vi "Main_Marvin.vi"() -> ()   [LabVIEW 2017]
uses:
  PCAN_Driver/ControlCAN.llb/DevType.ctl
  PCAN_Driver/ControlCAN.llb/CAN Channel.ctl
  PCAN_Driver/ControlCAN.llb/VCI_INIT_CONFIG.ctl
  PCAN_Driver/ControlCAN.llb/InitFlag.ctl
  PCAN_Driver/ControlCAN.llb/Fliter.ctl
  PCAN_Driver/ControlCAN.llb/Mode.ctl
  <vilib>/Utility/miscctls.llb/LVRowAndColumnTypeDef.ctl
  <vilib>/Utility/config.llb/Read Key (String).vi
  <vilib>/Utility/config.llb/Write Key (String).vi
  <vilib>/Utility/cursorutil.llb/Set Cursor (Icon Pict).vi
  PCAN_Driver/ControlCAN.lvlib
  <vilib>/Utility/config.llb/NI_LVConfig.lvlib
panel:
  in  "Index":string="5"
  out "Automation":bool
  out "ClosePanel 2":bool=TRUE
  out "ClosePanel":bool=TRUE
  out "Next SN":string
  out "Curret SN":string
  out "Array 5":dbl[](array[numeric])
  out "Array 4":dbl[](array[numeric])
  out "VC1500-2 Vel":dbl
  out "VC15100-1 Vel":dbl
  out "Array Test":T1(array[ring])
  out "TempAlg":bool=TRUE
  out "f":T2(ring)=enum."Empty"
  out "VC15100-2":dbl
  out "VC15100-1 Cur":dbl
  out "Auxiind":bool
  out "TempSensCalind":bool
  out "VisualInspectionResult":bool
  out "Burninind":bool
  out "TempControlind":bool
  out "MotorTempind":bool
  out "SpeedStopind":bool
  out "EnableTestind":bool
  out "ComTestind":bool
  out "SoftwareVer":string
  in  "SetSN":bool
  out "CurrentOffset":dbl
  out "Array 3":string[](array[string])
  out "Cal Value":string
  in  "Stop Burn-in":bool
  out "Array 2":dbl[](array[numeric])
  out "VISA resource name out":refnum<visa-resource-name>
  out "UUT":u8
  out "CAN Status":bool
  in  "Channel 2":T3 caption="Channel" items=["Channel 1", "Channel 2"]
  out "Config_CANAT":T9 {"DevType" items=["USB-CAN"=3, "USB-CAN2"=4]; "CanIndex" items=["通道1", "通道2"]; "VCI_INIT_CONFIG"."Fliter" items=["接收所有类型"=3, "只接收标准帧"=4, "只接收扩展帧"=7]; "VCI_INIT_CONFIG"."Mode" items=["正常工作", "自测模式（环回）", "仅侦听模式"]; "VCI_INIT_CONFIG"."InitFlag" items=["使用Flash参数", "使用界面设置参数"]}
  out "Array":u64[][](array[numeric]) format="%016x"
  out "Motor Phase Current RMS":dbl
  out "Ambient Temperature":dbl
  out "Speed error":bool
  out "Commutation err":bool
  out "Under voltage/Over voltage":bool
  out "Derated drive temp":bool
  out "Motor Over temperature":bool
  out "Motor Sensor temp Fauilre":bool
  out "Drive Over temperature":bool
  out "Drive Sensor temp Failure":bool
  out "Ambient Over temp":bool
  out "Ambient Sensor temp":bool
  out "DC Voltage":dbl
  out "DC Current":dbl
  out "Power transistor Heat sink Temp.":dbl
  out "Motor Stator Temp.":dbl
  out "Motor Speed RPM":dbl
  out "ECS State":u16
  out "Waveform Chart":dbl[](graph)
  out "UUT":string="EBAY"
  in  "Logger Path":path
  in  "Report":bool
  in  "Start":bool
  out "Table Out":string[][](table)=[["Led -Test & On/Rst.Msg.", "", "", "", "", "", "", "", "", " ", "", "", "", "", " "], ["Led Test", "", "#1", "-", "-", "", "", "", "", " ", "", "", "", "", ""], ["Com.RS232 Rst.Msg", "", "#2", "-", "-", "", "", "", "", " ", "", "", "", "", ""], ["Com.RS232 Ans.Msg", "", "#3", "-", "-", "", "", "", "", "", "", "", "", "", ""], ["", "", "", "", "", "", "", "", "", "", "", "", "", "", ""], ["Servo Voltage & Current", "", "", "", "", "", "", "", "FAIL", "", "", "", "", "", ""], ["Servo Voltage", "", "28.0", "+/-1", "V", "", "NaN", "", "FAIL", "", "6.0", "0.0", "100", "Average", ""], ["Servo Current", "", "0.15", "Max", "A", "", "NaN", "", "FAIL", "", "1.0", "0.0", "100", "Average", ""], ["", "", "", "", "", "", "", "", "", "", "", "", "", "", ""], ["Voltages Accurance", "", "", "", "", "", "", "", "FAIL", "", "", "", "", "", ""], ["Servo VCC 5V    ", "", "5.0", "+/-0.1", "V", "", "NaN", "", "FAIL", "", "1.0", "0.0", "100", "Average", ""], ["Servo VEE -6.8V", "", "-6.8", "+/-0.15", "V", "", "NaN", "", "FAIL", "", "1.0", "0.0", "100", "Average", ""], ["Ref_1_4.096V ?", "", "4.096", "+/-0.1", "V", "", "NaN", "", "FAIL", "", "1.0", "0.0", "100", "Average", ""], ["", "", "", "", "", "", "", "", "", "", "", "", "", "", ""], ["Power-Supply Changing", "", "", "", "", "", "", "", "", "", "", "", "", "", ""], ["Min. Power-Supply Volt. 18v ", "", "Led Flashes", "-", "-", "", "", "", "", "", "", "", "", "", ""], ["Max. Power-Supply Volt. 32v ", "", "Led Flashes", "-", "-", "", "", "", "", "", "", "", "", "", ""], ["Under Volt.Prot.28->5->18v", "", "Led Flashes", "-", "-", "", "", "", "", "", "", "", "", "", ""], ["", "", "", "", "", "", "", "", "", "", "", "", "", "", ""], ["Pos.Cmd.Accur.@Mode1", "", "Mxxxx=", "", "", "", "", "", "", "", "", "", "", "", ""], ["Pos.Cmnd.=0.5V F.B.", "", "59h", "+/-5", "", "", "", "", "", "", "1.0", "0.0", "1", "Average", ""], ["Pos.Cmnd.=2.0V F.B.", "", "195h", "+/-5", "", "", "", "", "", "", "1.0", "0.0", "1", "Average", ""], ["Pos.Cmnd.=4.5V F.B.", "", "3A5h", "+/-5", "", "", "", "", "", "", "1.0", "0.0", "1", "Average", ""], ["", "", "", "", "", "", "", "", "", "", "", "", "", "", ""], ["Pos.Cmd.Accur.@Mode2", "", "Mxxxx=", "", "", "", "", "", "FAIL", "", "", "", "", "", ""], ["Pos.Cmnd.=0.5V F.B", "", "59h", "+/-5", "", "", "57h", "", "PASS", "", "1.0", "0.0", "1", "Average", ""], ["Pos.Cmnd.=2.0V F.B.", "", "195h", "+/-5", "", "", "1CEh", "", "FAIL", "", "1.0", "0.0", "1", "Average", ""], ["Pos.Cmnd.=4.5V F.B.", "", "3A5h", "+/-5", "", "", "2BAh", "", "FAIL", "", "1.0", "0.0", "1", "Average", ""], ["", "", "", "", "", "", "", "", "", "", "", "", "", "", ""], ["Pot.Accur.@Mode1 ", "", "Rxxxx=", "", "", "", "", "", "FAIL", "", "", "", "", "", ""], ["Pot.simulate=0.5v Pot.Code.:", "", "173h", "+/-5", "", "", "7Bh", "", "FAIL", "", "1.0", "0.0", "1", "Average", ""], ["Pot.simulate=2.0v Pot.Code.:", "", "1F3h", "+/-5", "", "", "1F1h", "", "PASS", "", "1.0", "0.0", "1", "Average", ""], ["Pot.simulate=3.5v Pot.Code.:", "", "372h", "+/-5", "", "", "368h", "", "FAIL", "", "1.0", "0.0", "1", "Average", ""], ["", "", "", "", "", "", "", "", "", "", "", "", "", "", ""], ["Pot.Accur.@Mode2 ", "", "Rxxxx=", "", "", "", "", "", "FAIL", "", "", "", "", "", ""], ["Pot.simulate=0.5v Pot.Code.:", "", "C4h", "+/-5", "", "", "7Bh", "", "FAIL", "", "1.0", "0.0", "1", "Average", ""], ["Pot.simulate=2.0v Pot.Code.:", "", "1E3h", "+/-5", "", "", "1F1h", "", "FAIL", "", "1.0", "0.0", "1", "Average", ""], ["Pot.simulate=3.5v Pot.Code.:", "", "541h", "+/-5", "", "", "368h", "", "FAIL", "", "1.0", "0.0", "1", "Average", ""], ["", "", "", "", "", "", "", "", "", "", "", "", "", "", ""], ["Status Accur.@Mode1", "", "", "", "", "", "", "", "", "", "", "", "", "", ""], ["Pot. / Pos.Cmnd. 1.5v", "", "-1.8084", "+/-0.1", "V", "", "", "", "", "", "1.0", "0.0", "100", "Average", ""], ["Pot. / Pos.Cmnd. 2.0v", "", "-0.1584", "+/-0.1", "V", "", "", "", "", "", "1.0", "0.0", "100", "Average", ""], ["Pot. / Pos.Cmnd. 3.5v", "", "4.7916", "+/-0.1", "V", "", "", "", "", "", "1.0", "0.0", "100", "Average", ""]]
  in  "ATR":string[][](table)=[["Test Communication", "-", "-", "-", "-", ""], ["Set S/N", "-", "-", "-", "-", ""], ["Set Board Number", "-", "-", "-", "-", ""], [" ", "", "", "", "", ""], ["Test Communication", "-", "-", "-", "-", ""], ["Get S/N", "-", "-", "-", "", ""], ["Get Board Number", "-", "-", "-", "", ""], ["Get FW", "-", "-", "-", "", ""], ["Enable Motor", "", "", "", "", ""], ["Small position command", "", "", "", "", ""], ["Measure delta", "", "", "", "", ""], ["Velocity command", "", "", "", "", ""]]
  in  "Settings":bool
  in  "Refresh Button":bool
  out "Serial":bool
  in  "VISA resource name":refnum<visa-resource-name>="COM6"
  in  "Serial Com":bool
  in  "Help Button":bool
  out "Pannel User Message":string
  in  "Stop Button":bool
  # "Marvin"
  # "REDLER TECHNOLOGIES LTD"
  # "ver 1.2g"
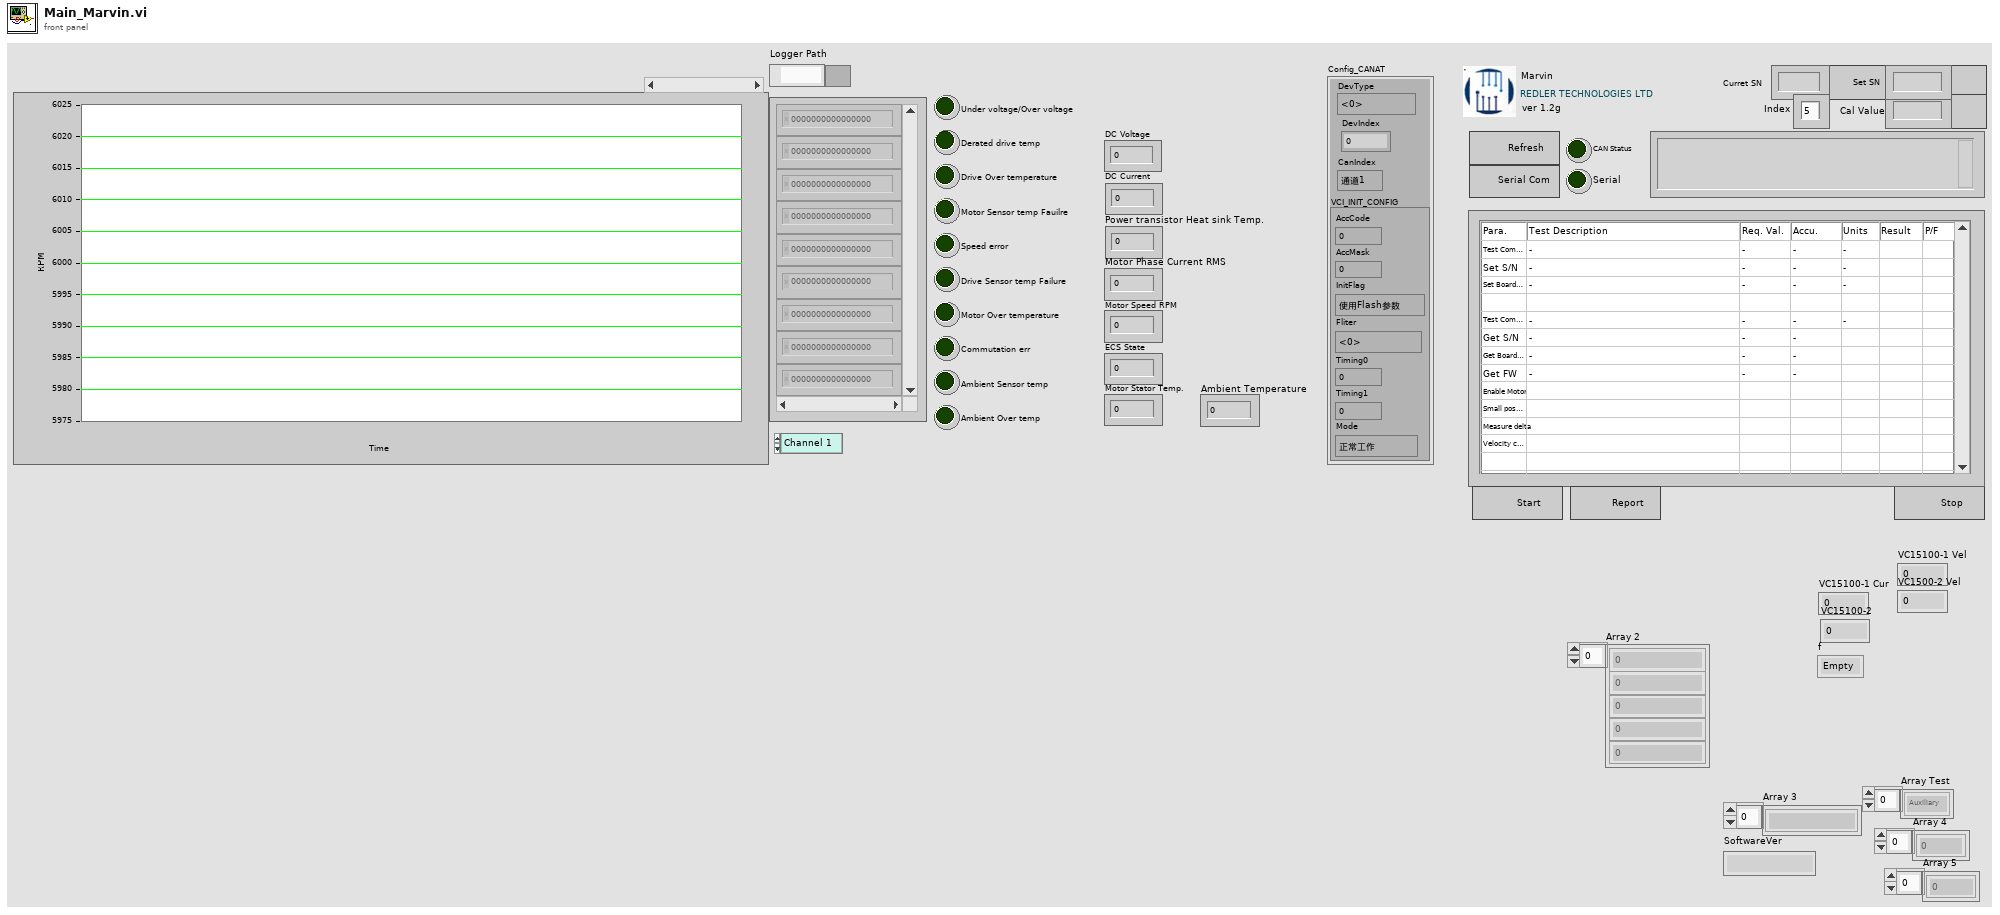
[diagram p1: front panel]
types:
  T1 = enum16{"Auxiliary", "Temp Sens Cal", "Com Test", "Enable Test", "Speed Command", "Stop Time", "Temp Control", "Burn in", "Visual Inspec", "Empty"}[]
  T2 = enum16{"Auxiliary", "Temp Sens Cal", "Com Test", "Enable Test", "Speed Command", "Stop Time", "Temp Control", "Burn in", "Visual Inspec", "Empty"}
  T3 = typedef "ControlCAN.lvlib/CAN Channel.ctl" = u32
  T4 = typedef "ControlCAN.lvlib/DevType.ctl" = u32
  T5 = typedef "ControlCAN.lvlib/VCI_INIT_CONFIG.ctl" = cluster{"AccCode":u32, "AccMask":u32, "InitFlag":T6, "Fliter":T7, "Timing0":u8, "Timing1":u8, "Mode":T8}
  T6 = typedef "ControlCAN.lvlib/InitFlag.ctl" = u32
  T7 = typedef "ControlCAN.lvlib/Fliter.ctl" = u8
  T8 = typedef "ControlCAN.lvlib/Mode.ctl" = u8
  T9 = cluster{"DevType":T4, "DevIndex":u32, "CanIndex":T3, "VCI_INIT_CONFIG":T5}
  T10 = cluster{"VISA":refnum<visa-resource-name>, "Array Test":enum16{"Auxiliary", "Temp Sens Cal", "Com Test", "Enable Test", "Speed Command", "Stop Time", "Temp Control", "Burn in", "Visual Inspec", "Empty"}[]}
  T11 = cluster{"ID":u32, "MSGTYPE":u8, "LEN":u8, "aDATA":u8[]}[]
  T12 = enum16{"Erase ATR Table", "Stop", "MainProgram", "Initialize"}
  T13 = enum8{"Enabled", "Disabled", "Disabled and Grayed Out"}
  T14 = enum16{"STOP", "VC15100-2", "RESET", "VC15100-1", "MD0"}
  T15 = typedef "NI_LVConfig.lvlib/Config Data RefNum.ctl" = refnum<k1>
  T16 = typedef "LVRowAndColumnTypeDef.ctl" = cluster{"Row":i32, "Column":i32}
  T17 = cluster{"ID":u32, "MSGTYPE":u8, "LEN":u8, "aDATA":u8[]}
  T18 = enum32{"Invalid", "Standard", "Closed", "Hidden", "Minimized", "Maximized"}
  T19 = enum16{"End", "Start", "Verify VR", "Verify UUT"}
  T20 = enum16{"open", "replace", "create", "open or create", "replace or create", "replace or create with confirmation"}
  T21 = typedef "ControlCAN.lvlib/VCI_CAN_OBJ.ctl" = cluster{"ID":u32, "TimeStamp":u32, "TimeFlag":u8, "SendType":u8, "RemoteFlag":u8, "ExternFlag":u8, "DataLen":u8, "Data":u8[], "Reserved":u8[]}
  T22 = cluster{"Type":enum16{"接收", "发送"}, "Channel":T3, "Time":timestamp, "VCI_CAN_OBJ":T21}[]
  T23 = cluster{"Type":enum16{"接收", "发送"}, "Channel":T3, "Time":timestamp, "VCI_CAN_OBJ":T21}
  T24 = typedef "LVPoint32TypeDef.ctl" = cluster{"Horizontal":i32, "Vertical":i32}
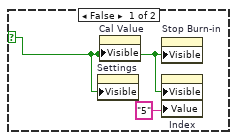
[diagram p3: hidden frame]
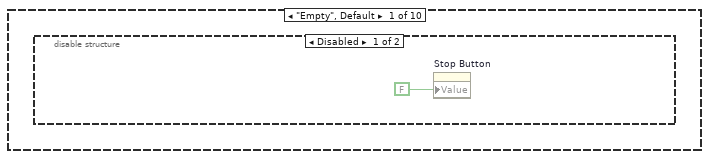
[diagram p6: hidden frame]
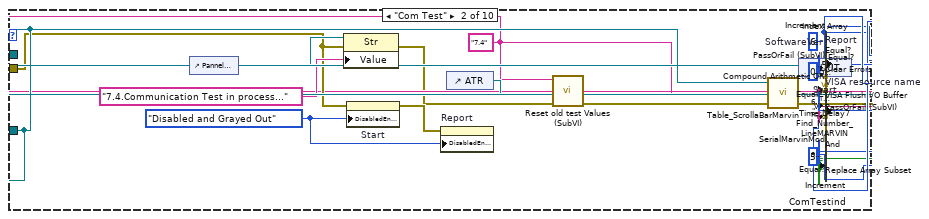
[diagram p8: hidden frame]
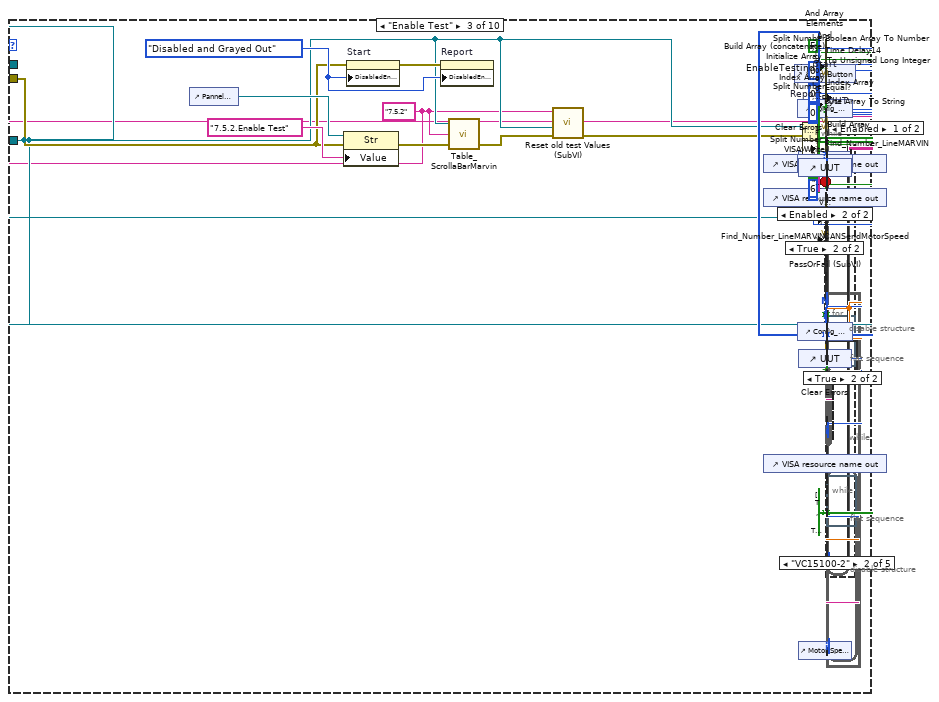
[diagram p9: hidden frame]
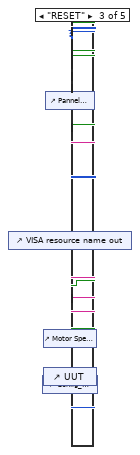
[diagram p17: hidden frame]
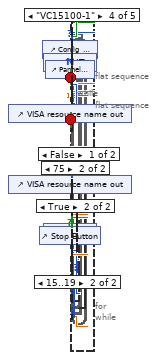
[diagram p18: hidden frame]
diagram:
  w1 = FALSE ("ClosePanel")
  w2 = "0" ("Next SN")
  w7 = 0.0 ("Val")
  (unwired) "[Marvin]\nEBAY Software Version = \"5.3.9\"\nAHU Software Version = \"5.3.8d\"\nEBAY Serial Number = \"0\"\nAHU Serial Number = \"0\""
  w21 = errorcluster {"status"=FALSE, "code"=0, "source"=""} ("error in (no error)")
  (unwired) string[][] [["6.1", "Visual Inspection", "", "", "", "", ""], ["6.1.1", "Verification of Components Not Installed", "N/A", "-", "", "", ""], ["", "", "", "", "", "", ""], ["6.1.2", "Manufacturing Defects", "N/A", "-", "", "", ""], ["", "", "", "", "", "", ""], ["6.2", "Power Supply Testing", "", "", "", "", ""], ["6.2.1", "Input Current Drawn", "", "", "", "", ""], ["6.2.1.1", "DC Input Current", "< 150", "-", "mA", "", ""], ["", "", "", "", "", "", ""], ["6.2.2", "Power Supply Voltages", "", "", "", "", ""], ["6.2.2.1", "12V", "12.0", "+/-0.500", "V", "", ""], ["6.2.2.2", "5V", "5.0", "+/-0.200", "V", "", ""], ["6.2.2.3", "3.3V", "3.3", "+/-0.100", "V", "", ""], ["6.2.2.4", "1.8V", "1.8", "+/-0.100", "V", "", ""], ["", "", "", "", "", "", ""], ["7", "Functional Test Procedure", "", "", "", "", ""], ["7.1", "Weight Check", "4180", "+/-10.00", "gr", "", ""], ["", "", "", "", "", "", ""], ["7.2", "Insulation Resistance Test", "", "", "", "", ""], ["7.2.1", "J3.B to Chassis", "> 1M", "-", "ohms", "", ""], ["7.2.2", "J1.16 to Chassis", "> 100K", "-", "ohms", "", ""], ["", "", "", "", "", "", ""], ["7.2", "Bonding Resistance", "", "", "", "", ""], ["7.2.3", "J1 Body to Chassis", "< 2m", "-", "ohms", "", ""], ["7.2.4", "J2  Body to Chassis", "< 2m", "-", "ohms", "", ""], ["7.2.5", "J3  Body to Chassis", "< 2m", "-", "ohms", "", ""], ["", "", "", "", "", "", ""], ["7.2.1", "CANbus Resistance Test", "", "", "", "", ""], ["7.2.1.1", "J1.17 to J1.18", "> 10K", "-", "ohms", "", ""], ["", "", "", "", "", "", ""], ["7.3", "Sealing Test", "N/A", "-", "", "", ""], ["", "", "", "", "", "", ""], ["7.4", "Communication Test", "", "", "", "", ""], ["7.4.1", "Serial RS-232", "N/A", "-", "", "", ""], ["7.4.2", "CAN Bus", "N/A", "-", "", "", ""], ["", "", "", "", "", "", ""], ["7.5", "Performances Tests", "", "", "", "", ""], ["7.5.1", "Reverse Polarity Test", "", "", "", "", ""], ["7.5.1.1", "DC Input Current", "< 1", "-", "mA", "", ""], ["", "", "", "", "", "", ""], ["7.5.2", "Enable Test", "", "", "", "", ""], ["7.5.2.1", "Fan Speed at Opened Enable ", "0", "-", "rpm", "", ""], ["7.5.2.2", "Fan Speed at Closed Enable ", "6000", "+/-200.0", "rpm", "", ""], ["7.5.2.3", "Motor Rotation Direction", "Counter-clockwise (Inlet)", "-", "", "", ""], ["", "", "", "", "", "", ""], ["7.5.3", "Stop Time Test ", "", "", "", "", ""], ["7.5.3.1", "Motor Stop time", "< 50", "-", "sec", "", ""], ["", "", "", "", "", "", ""], ["7.5.4", "Speed Command Test", "", "", "", "", ""], ["7.5.4.1", "Fan Speed", "6000", "+/-200.0", "rpm", "", ""], ["7.5.4.2", "Fan Speed", "11500", "+/-200.0", "rpm", "", ""], ["7.5.4.3", "Fan Speed", "15100", "+/-200.0", "rpm", "", ""], ["", "", "", "", "", "", ""], ["7.5.5", "Temperature Sensor Calibration Test", "", "", "", "", ""], ["7.5.5.1", "Sensor Reading Analog Offset", "0", "+/-0.100", ".", "", ""], ["", "", "", "", "", "", ""], ["7.5.6", "Temperature Control Algorithm Test", "", "", "", "", ""], ["7.5.6.1", "Tair <   68 ± 2 oC", "6000", "+/-200.0", "rpm", "", ""], ["7.5.6.2", "Tair >= 68 ± 2 oC", "11500", "+/-200.0", "rpm", "", ""], ["7.5.6.3", "Tair >= 88 ± 2 oC", "15100", "+/-400.0", "rpm", "", ""], ["7.5.6.4", "Tair <= 80 ± 2 oC", "11500", "+/-200.0", "rpm", "", ""], ["7.5.6.5", "Tair <= 60 ± 2 oC", "6000", "+/-200.0", "rpm", "", ""], ["", "", "", "", "", "", ""], ["7.5.7", "Burn-in Test", "", "", "", "", ""], ["7.5.7.1", "DC Input Current", "50", "+/-5.000", "A", "", ""], ["7.5.7.2", "Ambient Temperature", "25", "+/-13.00", "Deg.", "", ""], ["7.5.7.3", "After 10 min of operation", "", "", "Deg.", "", ""], ["7.5.7.4", "After 20 min of operation", "", "", "Deg.", "", ""], ["7.5.7.5", "After 30 min of operation", "", "", "Deg.", "", ""], ["7.5.7.6", "Auxiliary Cooling Fan 60 Deg", "On", "-", ".", "", ""], ["7.5.7.7", "Auxiliary Cooling Fan 55 Deg", "Off", "-", ".", "", ""]] ("data")
  n1 = disable-structure shown="Disabled" {
    frame Disabled {
      n2 = case shown="\" float\"" {
        selector: _ -> [_ _]
        tunnel: [u32 0 ("Data I") w30] -> _
        frame "Int", Default {
        }
        frame " float" {
          n3 = To Single Precision Float(number=sgl 0.0 ("Data F")) -> (single precision float=w32:sgl)
          n4 = call "Int_Float.vi"("1 Float in"=w32) -> ("1 Int out"=w31:i32)  [unwired: 1 in, 1 out]
          n5 = To Unsigned Long Integer(number=w31) -> (unsigned 32bit integer=w30:u32)
        }
      }
    }
    frame Enabled {
    }
  }
  n6 = disable-structure shown="Disabled" {
    frame Disabled {
      n7 = control-ref of="ATR"() -> (w34:refnum<vi>)
      n8 = call "Table_Put_Resultes_and_Decided_Pass_Fail.vi"("Table Ref."=w34) -> ("Table Out"=→"Table Out":string[][])  [unwired: 11 in, 3 out]
    }
    frame Enabled {
    }
  }
  n9 = disable-structure shown="Disabled" {
    frame Disabled {
      (unwired) 0.5 ("Delay Time (sec)")
      n10 = call <vilib>:"Unset Busy.vi"() -> ()  [unwired: 11 in, 1 out]
      n11 = call <vilib>:"Set Busy.vi"() -> ()  [unwired: 10 in, 2 out]
      n12 = call "Wait_Sec.vi"() -> ()  [unwired: 4 in, 1 out]
      n13 = call <vilib>:"Clear Errors.vi"() -> ()  [unwired: 6 in, 2 out]
    }
    frame Enabled {
    }
  }
  n14 = disable-structure shown="Disabled" {
    frame Disabled {
      (unwired) 5 ("disabled index (col)")
      (unwired) 3 ("index (row)")
      (unwired) 4 ("disabled index (col)")
      (unwired) 3 ("index (row)")
      n15 = property class="Tbl (strict)"() -> (reference out=w37:refnum<vi>, error out=w38:errorcluster, "Value"=w40:string[][])  [unwired: 2 in]
      n16 = Replace Array Subset(array=w40) -> (w39:string[][])  [unwired: 3 in]
      n17 = property class="Tbl (strict)"(reference=w37, error in=w38, "Value"=w39) -> (reference out=w35:refnum<vi>, error out=w36:errorcluster)
      n18 = call "PassOrFail (SubVI).vi"("error in (no error)"=w36, "Table in"=w35) -> ()  [unwired: 9 in, 1 out]
    }
    frame Enabled {
    }
  }
  n19 = disable-structure shown="Disabled" {
    frame Disabled {
      w43 = T13."Disabled and Grayed Out" ("Disabled")
      w44 = T13."Enabled" ("Disabled")
      n20 = control-ref of="Stop Button"() -> ()  [unwired: 1 out]
      n21 = control-ref of="Config_CANAT"() -> ()  [unwired: 1 out]
      n22 = control-ref of="UUT"() -> ()  [unwired: 1 out]
      n23 = control-ref of="Motor Speed RPM"() -> ()  [unwired: 1 out]
      n24 = control-ref of="Pannel User Message"() -> ()  [unwired: 1 out]
      n25 = control-ref of="ATR"() -> (w41:refnum<vi>)
      n26 = call "Reset old test Values (SubVI).vi"("Atr in"=w41) -> ()  [unwired: 10 in, 1 out]
      n27 = property on="Stop Button" class="Bool (strict)" props=["Value"]() -> ()  [unwired: 2 in, 3 out]
      n28 = property on="Start" class="Bool (strict)"("DisabledEnum"=w43) -> (error out=w42:errorcluster)  [unwired: 2 in, 1 out]
      n29 = property on="Start" class="Bool (strict)"("DisabledEnum"=w44) -> (error out=w45:errorcluster)  [unwired: 2 in, 1 out]
      n30 = property on="Report" class="Bool (strict)"(error in=w42, "DisabledEnum"=w43) -> ()  [unwired: 1 in, 2 out]
      n31 = property on="Report" class="Bool (strict)"(error in=w45, "DisabledEnum"=w44) -> ()  [unwired: 1 in, 2 out]
    }
    frame Enabled {
    }
  }
  n32 = disable-structure shown="Disabled" {
    frame Disabled {
    }
    frame Enabled {
    }
  }
  n33 = disable-structure shown="Disabled" {
    frame Disabled {
      n34 = control-ref of="Pannel User Message"() -> (w46:refnum<vi>)
      n35 = call "Write panel message (SubVI).vi"("Time to wait"=30.0, "String in"=w46) -> ()  [unwired: 9 in, 1 out]
    }
    frame Enabled {
    }
  }
  n36 = Obtain Queue(name (unnamed)="Test", element data type=T10 {"VISA"="COM1", "Array Test"=[]}, error in (no error)=w21) -> (queue out=w19:refnum<queue>)  [unwired: 2 in, 2 out]
  n37 = Obtain Queue(name (unnamed)="CAN RX Data", element data type=T11 [], error in (no error)=w21) -> (queue out=w23:refnum<queue>, error out=w13:errorcluster)  [unwired: 2 in, 1 out]
  n38 = control-ref of="ATR"() -> (w20:refnum<vi>)
  n39 = while {
    tunnel: w20 -> [w56]
    tunnel: w13 -> [w54]
    tunnel: w19 -> [w55]
    stop <- w50 stop-if-true
    n40 = Dequeue Element(queue=w55, error in (no error)=w54) -> (element=w53:T10, error out=w50:errorcluster)  [unwired: 1 in, 2 out]
    n41 = Unbundle By Name(w53) -> ("VISA"=w52:refnum<visa-resource-name>, "Array Test"=w51:T1)
    n42 = for {
      tunnel: w51 -> [w61] mode=indexing
      tunnel: w52 -> [w63]
      tunnel: w56 -> [w62]
      tunnel: w50 -> [w60]
      tunnel: [w60] -> w49
      stop <- w58 stop-if-true
      n43 = case shown="\"Temp Control\"" w61 {
        tunnel: w63 -> [_ _ _ _ _ _ _ _ w1757 _]
        tunnel: w62 -> [_ w97 w116 w768 w964 w1083 w1405 w1716 w1719 w1964]
        tunnel: w60 -> [_ w77 w132 w773 w971 w1095 w1431 w1712 w1752 w1973]
        frame "Empty", Default {
          n44 = disable-structure shown="Disabled" {
            frame Disabled {
              n45 = property on="Stop Button" class="Bool (strict)"("Value"=FALSE ("Stop Button")) -> ()  [unwired: 2 in, 2 out]
            }
            frame Enabled {
            }
          }
        }
        frame "Com Test" {
          w74 = T13."Enabled" ("Disabled")
          w75 = T13."Disabled and Grayed Out" ("Disabled")
          w98 = 6 ("disabled index (col)")
          w67 = "7.4" ("Test Paragraph")
          n46 = control-ref of="Pannel User Message"() -> (w95:refnum<vi>)
          n47 = property class="Str"(reference=w95, error in=w77, "Value"="7.4.Communication Test in process...") -> (error out=w66:errorcluster)  [unwired: 1 out]
          n48 = property on="Start" class="Bool (strict)"(error in=w77, "DisabledEnum"=w75) -> (error out=w76:errorcluster)  [unwired: 1 in, 1 out]
          n49 = property on="Report" class="Bool (strict)"(error in=w76, "DisabledEnum"=w75) -> ()  [unwired: 1 in, 2 out]
          n50 = control-ref of="ATR"() -> (w68:refnum<vi>)
          n51 = call "Reset old test Values (SubVI).vi"("error in"=w66, "Atr in"=w68, "Test Paragraph"=w67) -> ("error out"=w65:errorcluster)  [unwired: 8 in]
          n52 = call "Table_ScrollaBarMarvin.vi"("error in"=w65, "Line to focus"=w67, "reference in"=w97) -> ("error out"=w96:errorcluster)  [unwired: 2 out]
          n53 = control-ref of="UUT"() -> (w108:refnum<vi>)
          n54 = property on="SoftwareVer" class="Str"() -> ("Value"=w81:string)  [unwired: 2 in, 2 out]
          n55 = property on="VISA resource name" class="VISAName"() -> ("Value"=w92:refnum<visa-resource-name>)  [unwired: 2 in, 2 out]
          n56 = property class="Tbl (strict)"(reference=w97, error in=w96) -> (reference out=w85:refnum<vi>, error out=w112:errorcluster, "Value"=w69:string[][])
          n57 = Index Array(array=w69, index (col)=0 ("disabled index (col)")) -> (element=w113:string[])  [unwired: 1 in]
          n58 = call "Find_Number_LineMARVIN.vi"("Test Paragraph"=w67, "error in"=w112, "Row Headers[]"=w113) -> ("error out"=w110:errorcluster, "Line number"=w109:i32)  [unwired: 2 in, 2 out]
          n59 = call <vilib>:"Clear Errors.vi"("error in (no error)"=w110) -> ("error out"=w71:errorcluster)  [unwired: 5 in, 1 out]
          n60 = call "Time Delay7"("error in (no error)"=w71) -> ("error out"=w70:errorcluster)  [unwired: 10 in]
          n61 = VISA Flush I/O Buffer(VISA resource name=w92, error in (no error)=w70) -> (VISA resource name out=w90:refnum<visa-resource-name>, error out=w91:errorcluster)  [unwired: 1 in]
          n62 = call "SerialMarvinMod.vi"("error in (no error)"=w91, "write buffer"="VR\r\n", "VISA resource name"=w90) -> ("error out"=w84:errorcluster, "read buffer"=w87:string)  [unwired: 7 in]
          n63 = Equal?(x=w81, y=w87) -> (x = y?=w79:bool)
          n64 = Increment(x=w109) -> (x+1=w89:i32)
          n65 = Increment(x=w89) -> (x+1=w100:i32)
          n66 = Replace Array Subset(array=w69, new element=w87, index (row)=w89, index (col)=5 ("disabled index (col)")) -> (w86:string[][])
          n67 = property class="Tbl (strict)"(reference=w85, error in=w84, "Value"=w86) -> (error out=w83:errorcluster)  [unwired: 1 out]
          n68 = call "PassOrFail (SubVI).vi"("disabled index (col)"=w98, "index (row)"=w89, "error in (no error)"=w83, "Boolean"=w79, "Table in"=w97) -> ("error out"=w82:errorcluster)  [unwired: 6 in]
          n69 = property class="DigNum (strict)"(reference=w108, error in=w82) -> (error out=w99:errorcluster, "Value"=w107:u8)  [unwired: 1 out]
          n70 = Equal?(x=w107, y=u8 47) -> (x = y?=w103:bool)
          n71 = Equal?(x=w107, y=u8 63) -> (x = y?=w102:bool)
          n72 = Equal?(x=w107, y=u8 95) -> (x = y?=w101:bool)
          n73 = Compound Arithmetic op=OR(w103, w102, w101) -> (w80:bool)
          n74 = call "PassOrFail (SubVI).vi"("disabled index (col)"=w98, "index (row)"=w100, "error in (no error)"=w99, "Boolean"=w80, "Table in"=w97) -> ("error out"=w72:errorcluster)  [unwired: 6 in]
          n75 = property on="Start" class="Bool (strict)"(error in=w72, "DisabledEnum"=w74) -> (error out=w73:errorcluster)  [unwired: 1 in, 1 out]
          n76 = property on="Report" class="Bool (strict)"(error in=w73, "DisabledEnum"=w74) -> ()  [unwired: 1 in, 2 out]
          n77 = And(x=w80, y=w79) -> (x .and. y?=→"ComTestind":bool)
        }
        frame "Enable Test" {
          w131 = T13."Enabled" ("Disabled")
          w134 = T13."Disabled and Grayed Out" ("Disabled")
          w115 = "7.5.2" ("Test Paragraph")
          n78 = control-ref of="Pannel User Message"() -> (w150:refnum<vi>)
          n79 = property class="Str"(reference=w150, error in=w132, "Value"="7.5.2.Enable Test") -> (error out=w149:errorcluster)  [unwired: 1 out]
          n80 = property on="Start" class="Bool (strict)"(error in=w132, "DisabledEnum"=w134) -> (error out=w133:errorcluster)  [unwired: 1 in, 1 out]
          n81 = property on="Report" class="Bool (strict)"(error in=w133, "DisabledEnum"=w134) -> ()  [unwired: 1 in, 2 out]
          n82 = call "Table_ScrollaBarMarvin.vi"("error in"=w149, "Line to focus"=w115, "reference in"=w116) -> ("error out"=w188:errorcluster)  [unwired: 2 out]
          n83 = call "Reset old test Values (SubVI).vi"("error in"=w188, "Atr in"=w116, "Test Paragraph"=w115) -> ("error out"=w117:errorcluster)  [unwired: 8 in]
          n84 = control-ref of="VISA resource name out"() -> (w161:refnum<vi>)
          n85 = control-ref of="Stop Button"() -> (w127:refnum<vi>)
          n86 = control-ref of="Config_CANAT"() -> (w143:refnum<vi>)
          n87 = control-ref of="UUT"() -> (w144:refnum<vi>)
          n88 = property class="Tbl (strict)"(reference=w116, error in=w117) -> (error out=w190:errorcluster, "Value"=w191:string[][])  [unwired: 1 out]
          n89 = Initialize Array(FALSE, 14 ("dimension size")) -> (w173:bool[])
          n90 = Build Array (concatenate)(w173, bool[] [FALSE, FALSE, FALSE, FALSE, FALSE, FALSE, FALSE] ("array")) -> (w174:bool[])
          n91 = Boolean Array To Number(Boolean array=w174) -> (number=w172:u32)
          n92 = To Unsigned Long Integer(number=w172) -> (unsigned 32bit integer=w163:u32)
          n93 = Split Number(x=w163) -> (hi(x)=w168:u16, lo(x)=w169:u16)
          n94 = Split Number(x=w169) -> (hi(x)=w167:u8, lo(x)=w166:u8)
          n95 = Index Array(array=w191, index (col)=0 ("disabled index (col)")) -> (element=w192:string[])  [unwired: 1 in]
          n96 = property on="UUT" class="Str"() -> ("Value"=w125:string)  [unwired: 2 in, 2 out]
          n97 = Equal?(x=w125, y="EBAY") -> (x = y?=w123:bool)
          n98 = case shown="True" w123 {
            tunnel: [u16 12100 ("Motor Speed RPM") u16 15100 ("Motor Speed RPM")] -> w122
            tunnel: [11200.0 ("y") 14800.0 ("y")] -> w121
            tunnel: [13000.0 ("y") 16000.0 ("y")] -> w120
            tunnel: [20.0 ("y") 48.0 ("y")] -> w119
            tunnel: [15.0 ("y") 40.0 ("y")] -> w118
            frame False {
            }
            frame True {
            }
          }
          n99 = call "Find_Number_LineMARVIN.vi"("Test Paragraph"=w115, "error in"=w190, "Row Headers[]"=w192) -> ("error out"=w126:errorcluster, "Line number"=w187:i32)  [unwired: 2 in, 2 out]
          n100 = Split Number(x=w168) -> (hi(x)=w165:u8, lo(x)=w164:u8)
          n101 = Build Array(u8 75, u8 0 ("element"), u8 4 ("Length"), u8 2, w166, w167, w164, w165) -> (w171:u8[])
          n102 = Byte Array To String(unsigned byte array=w171) -> (string=w162:string)
          n103 = for {
            tunnel: w116 -> [w726]
            tunnel: w187 -> [w716]
            tunnel: u16[] [5000, 0, 5000] -> [w691] mode=indexing
            tunnel: [w714] -> w185
            tunnel: w126 -> [w692]
            tunnel: bool[] [TRUE, FALSE, TRUE] -> [w690] mode=indexing
            tunnel: bool[] [TRUE, TRUE, TRUE] -> [w689] mode=indexing
            tunnel: [w688] -> w140 mode=indexing
            i -> [w718]
            w719 = 200.0 ("y")
            n104 = control-ref of="VISA resource name out"() -> (w711:refnum<vi>)
            n105 = control-ref of="Config_CANAT"() -> (w733:refnum<vi>)
            n106 = Add(x=w691, y=w719) -> (x+y=w721:dbl)
            n107 = Increment(x=w718) -> (x+1=w717:i32)
            n108 = Subtract(x=w691, y=w719) -> (x-y=w720:dbl)
            n109 = Add(x=w716, y=w717) -> (x+y=w713:i32)
            n110 = case shown="True" w690 {
              tunnel: [bool[] [FALSE, FALSE, FALSE, FALSE, FALSE, FALSE, FALSE] ("array") bool[] [FALSE, FALSE, FALSE, TRUE, FALSE, FALSE, FALSE] ("array")] -> w698
              frame False {
              }
              frame True {
              }
            }
            n111 = Build Array (concatenate)(bool[] [FALSE, FALSE, FALSE, TRUE, FALSE, FALSE, FALSE, FALSE, FALSE, FALSE, FALSE, FALSE, FALSE, FALSE] ("array"), w698) -> (w699:bool[])
            n112 = Boolean Array To Number(Boolean array=w699) -> (number=w700:u32)
            n113 = To Unsigned Long Integer(number=w700) -> (unsigned 32bit integer=w709:u32)
            n114 = Split Number(x=w709) -> (hi(x)=w704:u16, lo(x)=w703:u16)
            n115 = Split Number(x=w703) -> (hi(x)=w705:u8, lo(x)=w706:u8)
            n116 = property class="VISAName"(reference=w711, error in=w692) -> (error out=w712:errorcluster, "Value"=w702:refnum<visa-resource-name>)  [unwired: 1 out]
            n117 = Split Number(x=w704) -> (hi(x)=w707:u8, lo(x)=w708:u8)
            n118 = Build Array(u8 75, u8 0 ("element"), u8 4 ("Length"), u8 2, w706, w705, w708, w707) -> (w701:u8[])
            n119 = Byte Array To String(unsigned byte array=w701) -> (string=w710:string)
            n120 = VISA Write(VISA resource name=w702, write buffer=w710, error in (no error)=w712) -> (error out=w693:errorcluster)  [unwired: 2 out]
            n121 = flat-sequence {
              tunnel: [w735] -> w687
              tunnel: w686 -> [w734]
              tunnel: [w734] -> w685
              frame #0 {
                n122 = call <vilib>:"High Resolution Relative Seconds.vi"() -> ("relative seconds"=w735:dbl)
              }
            }
            n123 = case shown="True" w689 {
              tunnel: w733 -> [_ w763]
              tunnel: [w758 w762] -> w686
              tunnel: w693 -> [w758 w760]
              frame False {
              }
              frame True {
                n124 = control-ref of="UUT"() -> (w764:refnum<vi>)
                n125 = call "CANSendMotorSpeed.vi"("Remote"=TRUE, "error in (no error)"=w760, "Motor Speed RPM"=u16 5000, "UUT"=w764, "Cluster in"=w763) -> ("error out"=w762:errorcluster)  [unwired: 6 in]
              }
            }
            n126 = while {
              tunnel: [w738] -> w728
              tunnel: [w755] -> w727
              tunnel: w685 -> [w754]
              tunnel: w687 -> [w752]
              stop <- w737 stop-if-true
              w749 = 15.0 ("y")
              n127 = control-ref of="Motor Speed RPM"() -> (w756:refnum<vi>)
              n128 = control-ref of="Pannel User Message"() -> (w750:refnum<vi>)
              n129 = property on="Stop Button" class="Bool (strict)"() -> ("Value"=w736:bool)  [unwired: 2 in, 2 out]
              n130 = Subtract(x=w753, y=w752) -> (x-y=w748:dbl)
              n131 = Greater Or Equal?(x=w748, y=w749) -> (x >= y?=w751:bool)
              n132 = Compound Arithmetic op=OR(w736, w751) -> (w737:bool)
              n133 = Subtract(x=w749, y=w748) -> (x-y=w740:dbl)
              n134 = Number To Fractional String(number=w740, precision (6)=i16 2) -> (F-format string=w746:string)  [unwired: 2 in]
              n135 = property class="DigNum (strict)"(reference=w756, error in=w754) -> (error out=w755:errorcluster, "Value"=w738:dbl)  [unwired: 1 out]
              n136 = Number To Decimal String(number=w738) -> (decimal integer string=w747:string)  [unwired: 1 in]
              n137 = Concatenate Strings("7.5.2.Enable Test in process...\nRemained Time: " ("string"), w746, "  sec." ("string"), "\r\n", "Motor speed [rpm]: " ("string"), w747) -> (w741:string)
              n138 = property class="Str"(reference=w750, "Value"=w741) -> ()  [unwired: 1 in, 2 out]
              n139 = flat-sequence {
                tunnel: [w757] -> w753
                frame #0 {
                  n140 = call <vilib>:"High Resolution Relative Seconds.vi"() -> ("relative seconds"=w757:dbl)
                }
              }
            }
            n141 = In Range and Coerce(upper limit=w721, x=w728, lower limit=w720) -> (In Range?=w688:bool)  [unwired: 1 out]
            n142 = call <vilib>:"Clear Errors.vi"("error in (no error)"=w727) -> ("error out"=w684:errorcluster)  [unwired: 5 in, 1 out]
            n143 = call "PassOrFail (SubVI).vi"("disabled index (col)"=6, "index (row)"=w713, "error in (no error)"=w684, "Boolean"=w688, "Table in"=w726) -> ("error out"=w730:errorcluster)  [unwired: 6 in]
            n144 = property class="Tbl (strict)"(reference=w726, error in=w730) -> (reference out=w722:refnum<vi>, error out=w731:errorcluster, "Value"=w723:string[][])
            n145 = Number To Fractional String(number=w728, precision (6)=i16 2) -> (F-format string=w725:string)  [unwired: 2 in]
            n146 = Replace Array Subset(array=w723, new element=w725, index (row)=w713, index (col)=5 ("disabled index (col)")) -> (w724:string[][])
            n147 = property class="Tbl (strict)"(reference=w722, error in=w731, "Value"=w724) -> (error out=w714:errorcluster)  [unwired: 1 out]
          }
          n148 = And Array Elements(Boolean array=w140) -> (logical AND=w139:bool)
          n149 = call <vilib>:"Clear Errors.vi"("error in (no error)"=w185) -> ("error out"=w136:errorcluster)  [unwired: 5 in, 1 out]
          n150 = disable-structure shown="Enabled" {
            disable-tunnel: w136 -> [w225 w681]
            disable-tunnel: [w224 w680] -> w142
            disable-tunnel: [w223 w682] -> w138
            disable-tunnel: T14."MD0" -> [w222 _]
            disable-tunnel: w127 -> [w221 _]
            disable-tunnel: w122 -> [w220 _]
            disable-tunnel: w121 -> [w219 _]
            disable-tunnel: w120 -> [w218 _]
            disable-tunnel: w119 -> [w217 _]
            disable-tunnel: w118 -> [w216 _]
            frame Enabled {
              n151 = while {
                tunnel: [w237] -> w223
                tunnel: w225 -> [w239]
                tunnel: [w238] -> w224
                shift-right: [w235] -> _
                shift-left: w222 -> [w236]
                tunnel: w221 -> [w231]
                tunnel: w220 -> [w230]
                tunnel: w219 -> [w229]
                tunnel: w218 -> [w228]
                tunnel: w217 -> [w227]
                tunnel: w216 -> [w226]
                stop <- w233 stop-if-true
                n152 = property on="Stop Button" class="Bool (strict)"() -> ("Value"=w232:bool)  [unwired: 2 in, 2 out]
                n153 = case shown="\"VC15100-2\"" w236 {
                  selector: w236 -> [w253 _ _ _ _]
                  tunnel: w239 -> [w254 w282 w436 w476 w642]
                  tunnel: [w254 w275 w442 w470 w641] -> w238
                  tunnel: [w246 FALSE FALSE FALSE FALSE] -> w237
                  tunnel: [w253 T14."STOP" T14."VC15100-2" w462 w645] -> w235
                  tunnel: [TRUE FALSE FALSE FALSE FALSE] -> w234
                  tunnel: w231 -> [_ w261 w420 w456 w636]
                  tunnel: w230 -> [_ w260 _ _ _]
                  tunnel: w229 -> [_ w259 _ _ _]
                  tunnel: w228 -> [_ w258 _ _ _]
                  tunnel: w227 -> [_ w257 _ w454 _]
                  tunnel: w226 -> [_ w256 _ w455 _]
                  frame "STOP", Default {
                    n154 = property on="VC15100-1 Vel" class="DigNum (strict)"() -> ("Value"=w245:dbl)  [unwired: 2 in, 2 out]
                    n155 = property on="VC1500-2 Vel" class="DigNum (strict)"() -> ("Value"=w244:dbl)  [unwired: 2 in, 2 out]
                    n156 = Subtract(x=w245, y=w244) -> (x-y=w243:dbl)
                    n157 = Absolute Value(x=w243) -> (abs(x)=w242:dbl)
                    n158 = Greater Or Equal?(x=w242, y=500.0) -> (x >= y?=w240:bool)
                    n159 = property on="VC15100-2" class="DigNum (strict)"() -> ("Value"=w252:dbl)  [unwired: 2 in, 2 out]
                    n160 = property on="VC15100-1 Cur" class="DigNum (strict)"() -> ("Value"=w251:dbl)  [unwired: 2 in, 2 out]
                    n161 = Subtract(x=w252, y=w251) -> (x-y=w248:dbl)
                    n162 = Absolute Value(x=w248) -> (abs(x)=w247:dbl)
                    n163 = Greater Or Equal?(x=w247, y=5.0) -> (x >= y?=w249:bool)
                    n164 = And(x=w240, y=w249) -> (x .and. y?=w246:bool)
                  }
                  frame "VC15100-2" {
                    n165 = control-ref of="VISA resource name out"() -> (w277:refnum<vi>)
                    n166 = control-ref of="Config_CANAT"() -> (w284:refnum<vi>)
                    n167 = control-ref of="UUT"() -> (w283:refnum<vi>)
                    n168 = call <vilib>:"Clear Errors.vi"("error in (no error)"=w279) -> ("error out"=w269:errorcluster)  [unwired: 5 in, 1 out]
                    n169 = call "CANSendMotorSpeed.vi"("Remote"=TRUE, "error in (no error)"=w282, "Motor Speed RPM"=w260, "UUT"=w283, "Cluster in"=w284) -> ("error out"=w280:errorcluster)  [unwired: 6 in]
                    n170 = flat-sequence {
                      tunnel: [w376] -> w281
                      tunnel: w280 -> [w375]
                      tunnel: [w375] -> w279
                      frame #0 {
                        n171 = call <vilib>:"High Resolution Relative Seconds.vi"() -> ("relative seconds"=w376:dbl)
                      }
                    }
                    n172 = property on="CurrentOffset" class="DigNum (strict)"() -> ("Value"=w270:dbl)  [unwired: 2 in, 2 out]
                    n173 = while {
                      tunnel: w281 -> [w400]
                      tunnel: w269 -> [w394]
                      tunnel: [w395] -> w276
                      tunnel: [w393] -> w274
                      tunnel: w261 -> [w381]
                      tunnel: w259 -> [w378]
                      tunnel: w258 -> [w377]
                      stop <- w398 stop-if-true
                      w379 = "7.5.2.4.Motor rotation direction test in process..." ("string")
                      n174 = control-ref of="Motor Speed RPM"() -> (w380:refnum<vi>)
                      n175 = control-ref of="Pannel User Message"() -> (w389:refnum<vi>)
                      n176 = property class="DigNum (strict)"(reference=w380, error in=w394) -> (error out=w395:errorcluster, "Value"=w384:dbl)  [unwired: 1 out]
                      "VC1500-2 Vel" <- w384
                      n177 = Number To Fractional String(number=w384, precision (6)=i16 2) -> (F-format string=w388:string)  [unwired: 2 in]
                      n178 = Concatenate Strings(w379, "\r\n", "Motor speed [rpm]: " ("string"), w388) -> (w383:string)
                      n179 = property class="Str"(reference=w389, "Value"=w383) -> ()  [unwired: 1 in, 2 out]
                      n180 = Greater Or Equal?(x=w384, y=w378) -> (x >= y?=w392:bool)
                      n181 = call <vilib>:"High Resolution Relative Seconds.vi"() -> ("relative seconds"=w401:dbl)
                      n182 = Subtract(x=w401, y=w400) -> (x-y=w396:dbl)
                      n183 = Less Or Equal?(x=w384, y=w377) -> (x <= y?=w391:bool)
                      n184 = And(x=w392, y=w391) -> (x .and. y?=w390:bool)
                      n185 = case shown="True" w390 {
                        selector: w390 -> [w402 w407]
                        tunnel: [w402 w406] -> w393
                        tunnel: w379 -> [_ w405]
                        tunnel: w381 -> [_ w404]
                        tunnel: w380 -> [_ w403]
                        frame False {
                        }
                        frame True {
                          n186 = flat-sequence {
                            tunnel: w407 -> [w414]
                            tunnel: [w414] -> w406
                            tunnel: w405 -> [w411]
                            tunnel: w404 -> [w410]
                            tunnel: w403 -> [w409]
                            frame #0 {
                              n187 = control-ref of="Pannel User Message"() -> (w412:refnum<vi>)
                              n188 = call "Write panel message (SubVI).vi"(4:"rpm"=w409, 5:"rpm"=TRUE ("rpm"), "Stop"=w410, "Time to wait"=20.0, "Strin"=w411, "String in"=w412) -> ()  [unwired: 5 in, 1 out]
                            }
                          }
                        }
                      }
                      n189 = Greater Or Equal?(x=w396, y=60.0) -> (x >= y?=w397:bool)
                      n190 = property on="Stop Button" class="Bool (strict)"() -> ("Value"=w382:bool)  [unwired: 2 in, 2 out]
                      n191 = Compound Arithmetic op=OR(w393, w397, w382) -> (w398:bool)
                    }
                    n192 = for {
                      N: 10 -> [_]
                      tunnel: w277 -> [w297]
                      tunnel: [w286] -> w272 mode=indexing
                      shift-right: [w287] -> w275
                      shift-left: w276 -> [w296]
                      tunnel: w256 -> [w285]
                      n193 = Byte Array To String(unsigned byte array=u8[] [75, 0, 4, 17, 0, 0, 0, 0] ("appended array")) -> (string=w294:string)
                      n194 = flat-sequence {
                        tunnel: w295 -> [w299]
                        tunnel: [w299] -> w292
                        tunnel: [w298] -> w291
                        frame #0 {
                          n195 = call <vilib>:"High Resolution Relative Seconds.vi"() -> ("relative seconds"=w298:dbl)
                        }
                      }
                      n196 = property class="VISAName"(reference=w297, error in=w296) -> (error out=w288:errorcluster, "Value"=w289:refnum<visa-resource-name>)  [unwired: 1 out]
                      n197 = VISA Write(VISA resource name=w289, write buffer=w294, error in (no error)=w288) -> (VISA resource name out=w293:refnum<visa-resource-name>, error out=w295:errorcluster)  [unwired: 1 out]
                      n198 = while {
                        tunnel: w293 -> [w313]
                        tunnel: w292 -> [w312]
                        tunnel: [w311] -> _
                        tunnel: [w310] -> w287
                        tunnel: w291 -> [w308]
                        tunnel: [w302] -> w286
                        tunnel: w285 -> [w300]
                        stop <- w304 stop-if-true
                        n199 = VISA Read(VISA resource name=w313, byte count=u32 1, error in (no error)=w312) -> (VISA resource name out=w315:refnum<visa-resource-name>, read buffer=w316:string, error out=w314:errorcluster)  [unwired: 1 out]
                        n200 = String To Byte Array(string=w316) -> (unsigned byte array=w319:u8[])
                        n201 = Index Array(array=w319, index=0) -> (element=w317:u8)
                        n202 = call <vilib>:"High Resolution Relative Seconds.vi"() -> ("relative seconds"=w309:dbl)
                        n203 = case shown="75" w317 {
                          tunnel: [w324 w329] -> w310
                          tunnel: w315 -> [w323 w338]
                          tunnel: w314 -> [w324 w337]
                          tunnel: [w323 w330] -> w311
                          tunnel: [u32 9999 w327] -> w302
                          tunnel: [FALSE w326] -> w303
                          tunnel: w300 -> [_ w325]
                          frame 0, Default {
                          }
                          frame 75 {
                            n204 = VISA Read(VISA resource name=w338, byte count=u32 3, error in (no error)=w337) -> (VISA resource name out=w333:refnum<visa-resource-name>, read buffer=w341:string, error out=w332:errorcluster)  [unwired: 1 out]
                            n205 = String To Byte Array(string=w341) -> (unsigned byte array=w331:u8[])
                            n206 = Index Array(array=w331, index #1=0 ("index")) -> (element #1=w336:u8, element #2=w334:u8)  [unwired: 2 in, 1 out]
                            n207 = Equal?(x=u8 0, y=w336) -> (x = y?=w335:bool)
                            n208 = case shown="True" w335 {
                              tunnel: [w344 w352] -> w329
                              tunnel: w334 -> [_ w359]
                              tunnel: w333 -> [w345 w358]
                              tunnel: w332 -> [w344 w357]
                              tunnel: w331 -> [_ w356]
                              tunnel: [w345 w354] -> w330
                              tunnel: [u32 9999 w348] -> w327
                              tunnel: [FALSE w347] -> w326
                              tunnel: w325 -> [_ w346]
                              frame False {
                              }
                              frame True {
                                n209 = VISA Read(VISA resource name=w358, byte count=w359, error in (no error)=w357) -> (VISA resource name out=w354:refnum<visa-resource-name>, read buffer=w353:string, error out=w352:errorcluster)  [unwired: 1 out]
                                n210 = String To Byte Array(string=w353) -> (unsigned byte array=w355:u8[])
                                n211 = Insert Into Array(array=w356, new element=w355) -> (w349:u8[])  [unwired: 1 in]
                                n212 = Index Array(array=w349, index #1=0 ("index")) -> (element #3=w350:u8)  [unwired: 2 in, 2 out]
                                n213 = case shown="15..19" w350 {
                                tunnel: w349 -> [_ w373]
                                tunnel: [u32 9999 w363] -> w348
                                tunnel: [FALSE w364] -> w347
                                tunnel: w346 -> [_ w362]
                                frame 0, Default {
                                }
                                frame 15..19 {
                                n214 = Index Array(array=w373, index #1=3 ("index")) -> (element #1=w372:u8, element #2=w371:u8, element #3=w370:u8, element #4=w369:u8)  [unwired: 3 in]
                                n215 = Join Numbers(hi=w369, lo=w370) -> ((hi.lo)=w367:u16)
                                n216 = Join Numbers(hi=w371, lo=w372) -> ((hi.lo)=w368:u16)
                                n217 = Join Numbers(hi=w367, lo=w368) -> ((hi.lo)=w365:u32)
                                n218 = Multiply(x=0.02003173828125, y=w365) -> (x*y=w363:dbl)
                                n219 = Greater Or Equal?(x=w363, y=w362) -> (x >= y?=w364:bool)
                                }
                                }
                              }
                            }
                          }
                        }
                        n220 = Subtract(x=w309, y=w308) -> (x-y=w307:dbl)
                        n221 = Greater Or Equal?(x=w307, y=2.0) -> (x >= y?=w305:bool)
                        n222 = property on="Stop Button" class="Bool (strict)"() -> ("Value"=w301:bool)  [unwired: 2 in, 2 out]
                        n223 = Compound Arithmetic op=OR(w301, w305, w303) -> (w304:bool)
                      }
                    }
                    n224 = Add Array Elements(numeric array=w272) -> (sum=w264:dbl)
                    n225 = Divide(x=w264, y=10.0 ("x")) -> (x/y=w263:dbl)
                    n226 = Subtract(x=w263, y=w270) -> (x-y=w271:dbl)
                    "VC15100-2" <- w271
                    n227 = Greater Or Equal?(x=w271, y=w257) -> (x >= y?=w273:bool)
                    n228 = And(x=w273, y=w274) -> ()  [unwired: 1 out]
                  }
                  frame "RESET" {
                    # "Venable + Power ON"
                    # "Venable + Power OFF"
                    n229 = control-ref of="VISA resource name out"() -> (w450:refnum<vi>)
                    n230 = control-ref of="Config_CANAT"() -> (w437:refnum<vi>)
                    n231 = control-ref of="Motor Speed RPM"() -> (w418:refnum<vi>)
                    n232 = control-ref of="UUT"() -> (w438:refnum<vi>)
                    n233 = control-ref of="Pannel User Message"() -> (w425:refnum<vi>)
                    n234 = Byte Array To String(unsigned byte array=u8[] [75, 0, 4, 2, 0, 0, 2, 0]) -> (string=w448:string)
                    n235 = Byte Array To String(unsigned byte array=u8[] [75, 0, 4, 2, 0, 0, 18, 0]) -> (string=w451:string)
                    n236 = property on="VISA resource name" class="VISAName"() -> ("Value"=w434:refnum<visa-resource-name>)  [unwired: 2 in, 2 out]
                    n237 = VISA Flush I/O Buffer(VISA resource name=w434) -> (VISA resource name out=w435:refnum<visa-resource-name>)  [unwired: 2 in, 1 out]
                    n238 = Concatenate Strings("EP=1\r\nMD[1]=" ("write buffer"), "1" ("string"), "\r\n" ("string")) -> (w433:string)
                    n239 = call <vilib>:"Clear Errors.vi"("error in (no error)"=w436) -> ("error out"=w416:errorcluster)  [unwired: 5 in, 1 out]
                    n240 = call "CANSendMotorSpeed.vi"("Remote"=TRUE, "error in (no error)"=w416, "Motor Speed RPM"=u16 0, "UUT"=w438, "Cluster in"=w437) -> ("error out"=w428:errorcluster)  [unwired: 6 in]
                    n241 = call <vilib>:"Clear Errors.vi"("error in (no error)"=w428) -> ("error out"=w415:errorcluster)  [unwired: 5 in, 1 out]
                    n242 = call "SerialMarvinMod.vi"("error in (no error)"=w415, "Clear Log"=FALSE, "write buffer"=w433, "VISA resource name"=w435) -> ("error out"=w427:errorcluster)  [unwired: 6 in, 1 out]
                    n243 = call <vilib>:"Clear Errors.vi"("error in (no error)"=w427) -> ("error out"=w426:errorcluster)  [unwired: 5 in, 1 out]
                    n244 = property class="VISAName"(reference=w450, error in=w426) -> (error out=w449:errorcluster, "Value"=w452:refnum<visa-resource-name>)  [unwired: 1 out]
                    n245 = VISA Write(VISA resource name=w452, write buffer=w451, error in (no error)=w449) -> (VISA resource name out=w447:refnum<visa-resource-name>, error out=w423:errorcluster)  [unwired: 1 out]
                    n246 = call "Write panel message (SubVI).vi"(4:"rpm"=w418, 5:"rpm"=FALSE ("rpm"), "PrintTime"=TRUE, "Stop"=w420, "error in (no error)"=w423, "Time to wait"=15.0, "Strin"="7.5.2.4.Motor rotation direction test in process...\nSet parameters" ("string"), "String in"=w425) -> ("error out"=w422:errorcluster)  [unwired: 3 in]
                    n247 = VISA Write(VISA resource name=w447, write buffer=w448, error in (no error)=w422) -> (error out=w442:errorcluster)  [unwired: 2 out]
                  }
                  frame "VC15100-1" {
                    n248 = control-ref of="Config_CANAT"() -> (w478:refnum<vi>)
                    n249 = control-ref of="UUT"() -> (w477:refnum<vi>)
                    n250 = call "CANSendMotorSpeed.vi"("Remote"=TRUE, "error in (no error)"=w476, "Motor Speed RPM"=u16 15100, "UUT"=w477, "Cluster in"=w478) -> ("error out"=w473:errorcluster)  [unwired: 6 in]
                    n251 = property on="CurrentOffset" class="DigNum (strict)"() -> ("Value"=w466:dbl)  [unwired: 2 in, 2 out]
                    n252 = call <vilib>:"Clear Errors.vi"("error in (no error)"=w472) -> ("error out"=w465:errorcluster)  [unwired: 5 in, 1 out]
                    n253 = flat-sequence {
                      tunnel: [w571] -> w474
                      tunnel: w473 -> [w570]
                      tunnel: [w570] -> w472
                      frame #0 {
                        n254 = call <vilib>:"High Resolution Relative Seconds.vi"() -> ("relative seconds"=w571:dbl)
                      }
                    }
                    n255 = while {
                      tunnel: w474 -> [w596]
                      tunnel: w465 -> [w591]
                      tunnel: [w590] -> w469
                      tunnel: w456 -> [w578]
                      tunnel: [w572] -> w453
                      stop <- w594 stop-if-true
                      w575 = "7.5.2.4.Motor rotation direction test in process..." ("string")
                      n256 = control-ref of="Motor Speed RPM"() -> (w576:refnum<vi>)
                      n257 = control-ref of="Pannel User Message"() -> (w582:refnum<vi>)
                      n258 = call <vilib>:"High Resolution Relative Seconds.vi"() -> ("relative seconds"=w597:dbl)
                      n259 = Subtract(x=w597, y=w596) -> (x-y=w592:dbl)
                      n260 = Greater Or Equal?(x=w592, y=60.0) -> (x >= y?=w593:bool)
                      n261 = property on="Stop Button" class="Bool (strict)"() -> ("Value"=w577:bool)  [unwired: 2 in, 2 out]
                      n262 = property class="DigNum (strict)"(reference=w576, error in=w591) -> (error out=w573:errorcluster, "Value"=w580:dbl)  [unwired: 1 out]
                      "VC15100-1 Vel" <- w580
                      n263 = Number To Fractional String(number=w580, precision (6)=i16 2) -> (F-format string=w581:string)  [unwired: 2 in]
                      n264 = Concatenate Strings(w575, "\r\n", "Motor speed [rpm]: " ("string"), w581) -> (w579:string)
                      n265 = property class="Str"(reference=w582, "Value"=w579) -> ()  [unwired: 1 in, 2 out]
                      n266 = Greater Or Equal?(x=w580, y=12800.0) -> (x >= y?=w589:bool)
                      n267 = Less Or Equal?(x=w580, y=16000.0) -> (x <= y?=w588:bool)
                      n268 = And(x=w589, y=w588) -> (x .and. y?=w586:bool)
                      n269 = case shown="False" w586 {
                        selector: w586 -> [w606 w614]
                        tunnel: [w606 w613] -> w590
                        tunnel: w575 -> [_ w612]
                        tunnel: w578 -> [_ w611]
                        tunnel: w576 -> [_ w610]
                        tunnel: [w602 w609] -> w574
                        tunnel: w573 -> [w599 w608]
                        tunnel: [w600 w607] -> w572
                        frame False {
                          n270 = control-ref of="VISA resource name out"() -> (w605:refnum<vi>)
                          n271 = control-ref of="Stop Button"() -> (w604:refnum<vi>)
                          n272 = call "Read ADC Current (SubVI).vi"("error out"=w599, "Bool Refnum"=w604, "VISAResourceName in"=w605) -> ("error out 2"=w600:errorcluster, "Result"=w603:dbl)  [unwired: 7 in]
                          n273 = Greater Or Equal?(x=w603, y=60.0) -> (x >= y?=w602:bool)
                        }
                        frame True {
                          n274 = flat-sequence {
                            tunnel: w614 -> [_]
                            tunnel: [FALSE] -> w613
                            tunnel: w612 -> [w621]
                            tunnel: w611 -> [w620]
                            tunnel: w610 -> [w619]
                            tunnel: [w618] -> w609
                            tunnel: w608 -> [w616]
                            tunnel: [w615] -> w607
                            frame #0 {
                              n275 = disable-structure shown="Enabled" {
                                disable-tunnel: w621 -> [w625 _]
                                disable-tunnel: w620 -> [w624 _]
                                disable-tunnel: w619 -> [w622 _]
                                disable-tunnel: [_ w630] -> w618
                                disable-tunnel: w616 -> [_ w629]
                                disable-tunnel: [_ w628] -> w615
                                frame Disabled {
                                n276 = control-ref of="Pannel User Message"() -> (w627:refnum<vi>)
                                n277 = call "Write panel message (SubVI).vi"(4:"rpm"=w622, 5:"rpm"=TRUE ("rpm"), "Stop"=w624, "Time to wait"=20.0, "Strin"=w625, "String in"=w627) -> ()  [unwired: 5 in, 1 out]
                                }
                                frame Enabled {
                                n278 = control-ref of="VISA resource name out"() -> (w634:refnum<vi>)
                                n279 = control-ref of="Stop Button"() -> (w633:refnum<vi>)
                                n280 = call "Read ADC Current (SubVI).vi"("error out"=w629, "Bool Refnum"=w633, "VISAResourceName in"=w634) -> ("error out 2"=w628:errorcluster, "Result"=w631:dbl)  [unwired: 7 in]
                                n281 = Greater Or Equal?(x=w631, y=60.0) -> (x >= y?=w630:bool)
                                }
                              }
                            }
                          }
                        }
                      }
                      n282 = Compound Arithmetic op=OR(w590, w593, w577, w574) -> (w594:bool)
                    }
                    n283 = for {
                      N: 10 -> [_]
                      tunnel: [w482] -> w460 mode=indexing
                      tunnel: [T14."RESET"] -> w462
                      tunnel: w453 -> [w492]
                      tunnel: [w483] -> w470
                      tunnel: w455 -> [w480]
                      n284 = control-ref of="VISA resource name out"() -> (w479:refnum<vi>)
                      n285 = Byte Array To String(unsigned byte array=u8[] [75, 0, 4, 17, 0, 0, 0, 0] ("appended array")) -> (string=w490:string)
                      n286 = property class="VISAName"(reference=w479, error in=w492) -> (error out=w484:errorcluster, "Value"=w485:refnum<visa-resource-name>)  [unwired: 1 out]
                      n287 = VISA Write(VISA resource name=w485, write buffer=w490, error in (no error)=w484) -> (VISA resource name out=w489:refnum<visa-resource-name>, error out=w491:errorcluster)  [unwired: 1 out]
                      n288 = flat-sequence {
                        tunnel: w491 -> [w494]
                        tunnel: [w494] -> w488
                        tunnel: [w493] -> w487
                        frame #0 {
                          n289 = call <vilib>:"High Resolution Relative Seconds.vi"() -> ("relative seconds"=w493:dbl)
                        }
                      }
                      n290 = while {
                        tunnel: w489 -> [w508]
                        tunnel: w488 -> [w507]
                        tunnel: [w506] -> _
                        tunnel: [w505] -> w483
                        tunnel: w487 -> [w503]
                        tunnel: [w497] -> w482
                        tunnel: w480 -> [w495]
                        stop <- w499 stop-if-true
                        n291 = call <vilib>:"High Resolution Relative Seconds.vi"() -> ("relative seconds"=w504:dbl)
                        n292 = Subtract(x=w504, y=w503) -> (x-y=w502:dbl)
                        n293 = Greater Or Equal?(x=w502, y=2.0) -> (x >= y?=w500:bool)
                        n294 = property on="Stop Button" class="Bool (strict)"() -> ("Value"=w496:bool)  [unwired: 2 in, 2 out]
                        n295 = VISA Read(VISA resource name=w508, byte count=u32 1, error in (no error)=w507) -> (VISA resource name out=w510:refnum<visa-resource-name>, read buffer=w511:string, error out=w509:errorcluster)  [unwired: 1 out]
                        n296 = String To Byte Array(string=w511) -> (unsigned byte array=w514:u8[])
                        n297 = Index Array(array=w514, index=0) -> (element=w512:u8)
                        n298 = case shown="75" w512 {
                          tunnel: [w519 w524] -> w505
                          tunnel: w510 -> [w518 w533]
                          tunnel: w509 -> [w519 w532]
                          tunnel: [w518 w525] -> w506
                          tunnel: [u32 9999 w522] -> w497
                          tunnel: [FALSE w521] -> w498
                          tunnel: w495 -> [_ w520]
                          frame 0, Default {
                          }
                          frame 75 {
                            n299 = VISA Read(VISA resource name=w533, byte count=u32 3, error in (no error)=w532) -> (VISA resource name out=w528:refnum<visa-resource-name>, read buffer=w536:string, error out=w527:errorcluster)  [unwired: 1 out]
                            n300 = String To Byte Array(string=w536) -> (unsigned byte array=w526:u8[])
                            n301 = Index Array(array=w526, index #1=0 ("index")) -> (element #1=w531:u8, element #2=w529:u8)  [unwired: 2 in, 1 out]
                            n302 = Equal?(x=u8 0, y=w531) -> (x = y?=w530:bool)
                            n303 = case shown="True" w530 {
                              tunnel: [w539 w547] -> w524
                              tunnel: w529 -> [_ w554]
                              tunnel: w528 -> [w540 w553]
                              tunnel: w527 -> [w539 w552]
                              tunnel: w526 -> [_ w551]
                              tunnel: [w540 w549] -> w525
                              tunnel: [u32 9999 w543] -> w522
                              tunnel: [FALSE w542] -> w521
                              tunnel: w520 -> [_ w541]
                              frame False {
                              }
                              frame True {
                                n304 = VISA Read(VISA resource name=w553, byte count=w554, error in (no error)=w552) -> (VISA resource name out=w549:refnum<visa-resource-name>, read buffer=w548:string, error out=w547:errorcluster)  [unwired: 1 out]
                                n305 = String To Byte Array(string=w548) -> (unsigned byte array=w550:u8[])
                                n306 = Insert Into Array(array=w551, new element=w550) -> (w544:u8[])  [unwired: 1 in]
                                n307 = Index Array(array=w544, index #1=0 ("index")) -> (element #3=w545:u8)  [unwired: 2 in, 2 out]
                                n308 = case shown="15..19" w545 {
                                tunnel: w544 -> [_ w568]
                                tunnel: [u32 9999 w558] -> w543
                                tunnel: [FALSE w559] -> w542
                                tunnel: w541 -> [_ w557]
                                frame 0, Default {
                                }
                                frame 15..19 {
                                n309 = Index Array(array=w568, index #1=3 ("index")) -> (element #1=w567:u8, element #2=w566:u8, element #3=w565:u8, element #4=w564:u8)  [unwired: 3 in]
                                n310 = Join Numbers(hi=w564, lo=w565) -> ((hi.lo)=w562:u16)
                                n311 = Join Numbers(hi=w566, lo=w567) -> ((hi.lo)=w563:u16)
                                n312 = Join Numbers(hi=w562, lo=w563) -> ((hi.lo)=w560:u32)
                                n313 = Multiply(x=0.02003173828125, y=w560) -> (x*y=w558:dbl)
                                n314 = Greater Or Equal?(x=w558, y=w557) -> (x >= y?=w559:bool)
                                }
                                }
                              }
                            }
                          }
                        }
                        n315 = Compound Arithmetic op=OR(w496, w500, w498) -> (w499:bool)
                      }
                    }
                    n316 = Add Array Elements(numeric array=w460) -> (sum=w459:dbl)
                    n317 = Divide(x=w459, y=10.0) -> (x/y=w457:dbl)
                    n318 = Subtract(x=w457, y=w466) -> (x-y=w467:dbl)
                    "VC15100-1 Cur" <- w467
                    n319 = Greater Or Equal?(x=w467, y=w454) -> (x >= y?=w468:bool)
                    n320 = And(x=w468, y=w469) -> ()  [unwired: 1 out]
                  }
                  frame "MD0" {
                    n321 = control-ref of="Pannel User Message"() -> (w639:refnum<vi>)
                    n322 = property on="Serial" class="Bool (strict)"(error in=w642) -> (error out=w638:errorcluster, "Value"=w644:bool)  [unwired: 1 in, 1 out]
                    n323 = Select(t=T14."VC15100-1", s=w644, f=T14."STOP") -> (s? t:f=w645:T14)
                    n324 = property class="Str"(reference=w639, error in=w638, "Value"="7.5.2.4.Motor rotation direction test in process..." ("string")) -> (error out=w637:errorcluster)  [unwired: 1 out]
                    n325 = case shown="True" w644 {
                      tunnel: [w648 w658] -> w641
                      tunnel: w637 -> [w648 w657]
                      tunnel: w636 -> [_ w652]
                      frame False {
                        n326 = call "Display Message to User6"() -> ()  [unwired: 10 in, 2 out]
                      }
                      frame True {
                        (unwired) TRUE ("Remote")
                        # "Venable + Power ON"
                        # "Venable + Power OFF"
                        n327 = control-ref of="VISA resource name out"() -> (w665:refnum<vi>)
                        n328 = control-ref of="Config_CANAT"() -> (w671:refnum<vi>)
                        n329 = control-ref of="UUT"() -> (w672:refnum<vi>)
                        n330 = control-ref of="Motor Speed RPM"() -> (w650:refnum<vi>)
                        n331 = control-ref of="Pannel User Message"() -> (w656:refnum<vi>)
                        n332 = Byte Array To String(unsigned byte array=u8[] [75, 0, 4, 2, 0, 0, 2, 0]) -> (string=w663:string)
                        n333 = Byte Array To String(unsigned byte array=u8[] [75, 0, 4, 2, 0, 0, 18, 0]) -> (string=w666:string)
                        n334 = property on="VISA resource name" class="VISAName"() -> ("Value"=w678:refnum<visa-resource-name>)  [unwired: 2 in, 2 out]
                        n335 = VISA Flush I/O Buffer(VISA resource name=w678) -> (VISA resource name out=w679:refnum<visa-resource-name>)  [unwired: 2 in, 1 out]
                        n336 = Concatenate Strings("EP=1\r\nMD[1]=" ("write buffer"), "0" ("string"), "\r\n" ("string")) -> (w677:string)
                        n337 = call "CANSendMotorSpeed.vi"("error in (no error)"=w657, "Motor Speed RPM"=u16 0, "UUT"=w672, "Cluster in"=w671) -> ("error out"=w669:errorcluster)  [unwired: 7 in]
                        n338 = call "SerialMarvinMod.vi"("error in (no error)"=w669, "Clear Log"=FALSE, "write buffer"=w677, "VISA resource name"=w679) -> ("error out"=w668:errorcluster)  [unwired: 6 in, 1 out]
                        n339 = call <vilib>:"Clear Errors.vi"("error in (no error)"=w668) -> ("error out"=w659:errorcluster)  [unwired: 5 in, 1 out]
                        n340 = property class="VISAName"(reference=w665, error in=w659) -> (error out=w664:errorcluster, "Value"=w667:refnum<visa-resource-name>)  [unwired: 1 out]
                        n341 = VISA Write(VISA resource name=w667, write buffer=w666, error in (no error)=w664) -> (VISA resource name out=w662:refnum<visa-resource-name>, error out=w654:errorcluster)  [unwired: 1 out]
                        n342 = call "Write panel message (SubVI).vi"(4:"rpm"=w650, 5:"rpm"=FALSE ("rpm"), "Stop"=w652, "error in (no error)"=w654, "Time to wait"=15.0, "Strin"="7.5.2.4.Motor rotation direction test in process...\nSet parameters" ("string"), "String in"=w656) -> ("error out"=w653:errorcluster)  [unwired: 4 in]
                        n343 = VISA Write(VISA resource name=w662, write buffer=w663, error in (no error)=w653) -> (error out=w658:errorcluster)  [unwired: 2 out]
                      }
                    }
                  }
                }
                n344 = Compound Arithmetic op=OR(w234, w232) -> (w233:bool)
              }
            }
            frame Disabled {
              n345 = call "Display Message to User"("error in (no error)"=w681) -> ("error out"=w680:errorcluster, "YES"=w682:bool)  [unwired: 9 in]
            }
          }
          n346 = And(x=w139, y=w138) -> (x .and. y?=→"EnableTestind":bool)
          n347 = call "CANSendMotorSpeed.vi"("Remote"=FALSE, "error in (no error)"=w142, "Motor Speed RPM"=u16 0, "UUT"=w144, "Cluster in"=w143) -> ("error out"=w141:errorcluster)  [unwired: 6 in]
          n348 = property class="Tbl (strict)"(reference=w116, error in=w141) -> (reference out=w175:refnum<vi>, error out=w182:errorcluster, "Value"=w181:string[][])
          n349 = Index Array(array=w181, index (col)=0 ("disabled index (col)")) -> (element=w180:string[])  [unwired: 1 in]
          n350 = call "Find_Number_LineMARVIN.vi"("Test Paragraph"="7.5.2.4", "error in"=w182, "Row Headers[]"=w180) -> ("error out"=w179:errorcluster, "Line number"=w176:i32)  [unwired: 2 in, 2 out]
          n351 = call "PassOrFail (SubVI).vi"("disabled index (col)"=6, "index (row)"=w176, "error in (no error)"=w179, "Boolean"=w138, "Table in"=w175) -> ("error out"=w177:errorcluster)  [unwired: 6 in]
          n352 = disable-structure shown="Enabled" {
            disable-tunnel: w177 -> [w209 w215]
            disable-tunnel: w176 -> [w206 _]
            disable-tunnel: _ -> [w205 _]
            disable-tunnel: w175 -> [w204 _]
            disable-tunnel: [w203 w215] -> w152
            frame Disabled {
              n353 = property class="Tbl (strict)"(reference=w204, error in=w209) -> (reference out=w214:refnum<vi>, error out=w210:errorcluster, "Value"=w213:string[][])
              n354 = Number To Fractional String(number=w205, precision (6)=i16 4) -> (F-format string=w207:string)  [unwired: 2 in]
              n355 = Replace Array Subset(array=w213, new element=w207, index (row)=w206, index (col)=5 ("disabled index (col)")) -> (w212:string[][])
              n356 = property class="Tbl (strict)"(reference=w214, error in=w210, "Value"=w212) -> (error out=w203:errorcluster)  [unwired: 1 out]
            }
            frame Enabled {
            }
          }
          n357 = property class="VISAName"(reference=w161, error in=w152) -> (error out=w160:errorcluster, "Value"=w170:refnum<visa-resource-name>)  [unwired: 1 out]
          n358 = VISA Write(VISA resource name=w170, write buffer=w162, error in (no error)=w160) -> (error out=w129:errorcluster)  [unwired: 2 out]
          n359 = call <vilib>:"Clear Errors.vi"("error in (no error)"=w129) -> ("error out"=w128:errorcluster)  [unwired: 5 in, 1 out]
          n360 = call "Time Delay14"("error in (no error)"=w128) -> ("error out"=w114:errorcluster)  [unwired: 10 in]
          n361 = property on="Start" class="Bool (strict)"(error in=w114, "DisabledEnum"=w131) -> (error out=w130:errorcluster)  [unwired: 1 in, 1 out]
          n362 = property on="Report" class="Bool (strict)"(error in=w130, "DisabledEnum"=w131) -> ()  [unwired: 1 in, 2 out]
        }
        frame "Speed Command" {
          w774 = T13."Disabled and Grayed Out" ("Disabled")
          w778 = T13."Enabled" ("Disabled")
          w858 = "7.5.3" ("Test Paragraph")
          w767 = "7.5.4" ("Test Paragraph")
          n363 = control-ref of="Pannel User Message"() -> (w789:refnum<vi>)
          n364 = property class="Str"(reference=w789, error in=w773, "Value"="7.5.4.Speed Command Test") -> (error out=w788:errorcluster)  [unwired: 1 out]
          n365 = property on="Start" class="Bool (strict)"(error in=w773, "DisabledEnum"=w774) -> (error out=w775:errorcluster)  [unwired: 1 in, 1 out]
          n366 = Initialize Array(FALSE, 14 ("dimension size")) -> (w836:bool[])
          n367 = property on="Report" class="Bool (strict)"(error in=w775, "DisabledEnum"=w774) -> ()  [unwired: 1 in, 2 out]
          n368 = Build Array (concatenate)(w836, bool[] [FALSE, FALSE, FALSE, TRUE, FALSE, FALSE, FALSE] ("array")) -> (w837:bool[])
          n369 = call "Table_ScrollaBarMarvin.vi"("error in"=w788, "Line to focus"=w767, "reference in"=w768) -> ("error out"=w869:errorcluster)  [unwired: 2 out]
          n370 = Boolean Array To Number(Boolean array=w837) -> (number=w835:u32)
          n371 = call "Reset old test Values (SubVI).vi"("error in"=w869, "Atr in"=w768, "Test Paragraph"=w767) -> ("error out"=w769:errorcluster)  [unwired: 8 in]
          n372 = control-ref of="VISA resource name out"() -> (w800:refnum<vi>)
          n373 = control-ref of="VISA resource name out"() -> (w824:refnum<vi>)
          n374 = control-ref of="Config_CANAT"() -> (w866:refnum<vi>)
          n375 = control-ref of="UUT"() -> (w865:refnum<vi>)
          n376 = property class="Tbl (strict)"(reference=w768, error in=w769) -> (error out=w871:errorcluster, "Value"=w872:string[][])  [unwired: 1 out]
          n377 = To Unsigned Long Integer(number=w835) -> (unsigned 32bit integer=w826:u32)
          n378 = Initialize Array(FALSE, 14 ("dimension size")) -> (w812:bool[])
          n379 = Build Array (concatenate)(w812, bool[] [FALSE, FALSE, FALSE, FALSE, FALSE, FALSE, FALSE] ("array")) -> (w813:bool[])
          n380 = Boolean Array To Number(Boolean array=w813) -> (number=w811:u32)
          n381 = To Unsigned Long Integer(number=w811) -> (unsigned 32bit integer=w802:u32)
          n382 = Split Number(x=w802) -> (hi(x)=w807:u16, lo(x)=w808:u16)
          n383 = Split Number(x=w808) -> (hi(x)=w806:u8, lo(x)=w805:u8)
          n384 = property on="UUT" class="Str"() -> ("Value"=w772:string)  [unwired: 2 in, 2 out]
          n385 = Equal?(x=w772, y="EBAY") -> (x = y?=w770:bool)
          n386 = case shown="False" w770 {
            tunnel: [u16[] [6000, 9000, 12100] u16[] [6000, 11500, 15100]] -> w867
            frame False {
            }
            frame True {
            }
          }
          n387 = Split Number(x=w826) -> (hi(x)=w831:u16, lo(x)=w832:u16)
          n388 = Split Number(x=w807) -> (hi(x)=w804:u8, lo(x)=w803:u8)
          n389 = Build Array(u8 75, u8 0 ("element"), u8 4 ("Length"), u8 2, w805, w806, w803, w804) -> (w810:u8[])
          n390 = Byte Array To String(unsigned byte array=w810) -> (string=w801:string)
          n391 = Split Number(x=w832) -> (hi(x)=w830:u8, lo(x)=w829:u8)
          n392 = Concatenate Strings("7.5.3.Stop Time Test in process... ", "\r\n", "Motor Speed [rpm]: " ("string")) -> (w783:string)
          n393 = Index Array(array=w872, index (col)=0 ("disabled index (col)")) -> (element=w873:string[])  [unwired: 1 in]
          n394 = Split Number(x=w831) -> (hi(x)=w828:u8, lo(x)=w827:u8)
          n395 = Build Array(u8 75, u8 0 ("element"), u8 4 ("Length"), u8 2, w829, w830, w827, w828) -> (w834:u8[])
          n396 = Byte Array To String(unsigned byte array=w834) -> (string=w825:string)
          n397 = call "Find_Number_LineMARVIN.vi"("Test Paragraph"=w767, "error in"=w871, "Row Headers[]"=w873) -> ("error out"=w815:errorcluster, "Line number"=w868:i32)  [unwired: 2 in, 2 out]
          n398 = property class="VISAName"(reference=w824, error in=w815) -> (error out=w823:errorcluster, "Value"=w833:refnum<visa-resource-name>)  [unwired: 1 out]
          n399 = VISA Write(VISA resource name=w833, write buffer=w825, error in (no error)=w823) -> (error out=w814:errorcluster)  [unwired: 2 out]
          n400 = flat-sequence {
            tunnel: [w877] -> w862
            tunnel: w861 -> [w876]
            tunnel: [w876] -> w860
            frame #0 {
              n401 = call <vilib>:"High Resolution Relative Seconds.vi"() -> ("relative seconds"=w877:dbl)
            }
          }
          n402 = for {
            tunnel: w814 -> [w921]
            tunnel: w768 -> [w918]
            tunnel: w868 -> [w907]
            tunnel: w867 -> [w910] mode=indexing
            tunnel: [w905] -> w864
            tunnel: [w897] -> w782 mode=indexing
            i -> [w909]
            w911 = 200.0 ("y")
            n403 = control-ref of="Config_CANAT"() -> (w927:refnum<vi>)
            n404 = control-ref of="Motor Speed RPM"() -> (w926:refnum<vi>)
            n405 = control-ref of="UUT"() -> (w928:refnum<vi>)
            n406 = Add(x=w910, y=w911) -> (x+y=w913:dbl)
            n407 = Subtract(x=w910, y=w911) -> (x-y=w912:dbl)
            n408 = Increment(x=w909) -> (x+1=w908:i32)
            n409 = Add(x=w907, y=w908) -> (x+y=w904:i32)
            n410 = call "CANSendMotorSpeed.vi"("Remote"=TRUE, "error in (no error)"=w921, "Motor Speed RPM"=w910, "UUT"=w928, "Cluster in"=w927) -> ("error out"=w902:errorcluster)  [unwired: 6 in]
            n411 = call <vilib>:"High Resolution Relative Seconds.vi"() -> ("relative seconds"=w898:dbl)
            n412 = while {
              tunnel: w902 -> [w948]
              tunnel: [w948] -> w901
              tunnel: "7.5.4.Speed Command Test" ("Value") -> [w945]
              tunnel: "Time to wait: " ("Value") -> [w943]
              tunnel: w898 -> [w941]
              stop <- w933 stop-if-true
              n413 = control-ref of="Pannel User Message"() -> (w947:refnum<vi>)
              n414 = call <vilib>:"High Resolution Relative Seconds.vi"() -> ("relative seconds"=w942:dbl)
              n415 = Subtract(x=w942, y=w941) -> (x-y=w939:dbl)
              n416 = property on="Stop Button" class="Bool (strict)"() -> ("Value"=w932:bool)  [unwired: 2 in, 2 out]
              n417 = Subtract(x=35.0, y=w939) -> (x-y=w934:dbl)
              n418 = Less Or Equal To 0?(x=w934) -> (x <= 0?=w940:bool)
              n419 = Compound Arithmetic op=OR(w940, w932) -> (w933:bool)
              n420 = Number To Fractional String(number=w934, precision (6)=i16 2) -> (F-format string=w936:string)  [unwired: 2 in]
              n421 = property on="Motor Speed RPM" class="DigNum (strict)"() -> ("Value"=w930:dbl)  [unwired: 2 in, 2 out]
              n422 = Number To Fractional String(number=w930, precision (6)=i16 2) -> (F-format string=w929:string)  [unwired: 2 in]
              n423 = Concatenate Strings(w945, "\r\n", w943, w936, "  Sec.\nMotor speed [rpm]: " ("string"), w929) -> (w946:string)
              n424 = property class="Str"(reference=w947, "Value"=w946) -> ()  [unwired: 1 in, 2 out]
            }
            n425 = property class="DigNum (strict)"(reference=w926, error in=w901) -> (error out=w919:errorcluster, "Value"=w920:dbl)  [unwired: 1 out]
            n426 = In Range and Coerce(upper limit=w913, x=w920, lower limit=w912) -> (In Range?=w897:bool)  [unwired: 1 out]
            n427 = call "PassOrFail (SubVI).vi"("disabled index (col)"=6, "index (row)"=w904, "error in (no error)"=w919, "Boolean"=w897, "Table in"=w918) -> ("error out"=w923:errorcluster)  [unwired: 6 in]
            n428 = property class="Tbl (strict)"(reference=w918, error in=w923) -> (reference out=w914:refnum<vi>, error out=w924:errorcluster, "Value"=w915:string[][])
            n429 = Number To Fractional String(number=w920, precision (6)=i16 2) -> (F-format string=w917:string)  [unwired: 2 in]
            n430 = Replace Array Subset(array=w915, new element=w917, index (row)=w904, index (col)=5 ("disabled index (col)")) -> (w916:string[][])
            n431 = property class="Tbl (strict)"(reference=w914, error in=w924, "Value"=w916) -> (error out=w905:errorcluster)  [unwired: 1 out]
          }
          n432 = call "CANSendMotorSpeed.vi"("Remote"=TRUE, "error in (no error)"=w864, "Motor Speed RPM"=u16 0, "UUT"=w865, "Cluster in"=w866) -> ("error out"=w861:errorcluster)  [unwired: 6 in]
          n433 = while {
            tunnel: w862 -> [w893]
            tunnel: w860 -> [w887]
            tunnel: [w888] -> w839
            tunnel: [w884] -> w851
            tunnel: w783 -> [w881]
            stop <- w891 stop-if-true
            n434 = control-ref of="Motor Speed RPM"() -> (w896:refnum<vi>)
            n435 = control-ref of="Pannel User Message"() -> (w886:refnum<vi>)
            n436 = call <vilib>:"High Resolution Relative Seconds.vi"() -> ("relative seconds"=w894:dbl)
            n437 = Subtract(x=w894, y=w893) -> (x-y=w888:dbl)
            n438 = property class="DigNum (strict)"(reference=w896, error in=w887) -> (error out=w885:errorcluster, "Value"=w879:dbl)  [unwired: 1 out]
            n439 = Number To Fractional String(number=w879, precision (6)=i16 2) -> (F-format string=w880:string)  [unwired: 2 in]
            n440 = Concatenate Strings(w881, w880) -> (w882:string)
            n441 = property class="Str"(reference=w886, error in=w885, "Value"=w882) -> (error out=w884:errorcluster)  [unwired: 1 out]
            n442 = Less Or Equal?(x=w879, y=0.0) -> (x <= y?=w890:bool)
            n443 = Greater Or Equal?(x=w888, y=50.0) -> (x >= y?=w889:bool)
            n444 = property on="Stop Button" class="Bool (strict)"() -> ("Value"=w878:bool)  [unwired: 2 in, 2 out]
            n445 = Compound Arithmetic op=OR(w890, w889, w878) -> (w891:bool)
          }
          n446 = Less?(x=w839, y=50.0) -> (x < y?=w781:bool)
          n447 = call "Table_ScrollaBarMarvin.vi"("error in"=w851, "Line to focus"=w858, "reference in"=w768) -> ("error out"=w859:errorcluster)  [unwired: 2 out]
          n448 = property class="Tbl (strict)"(reference=w768, error in=w859) -> (reference out=w838:refnum<vi>, error out=w856:errorcluster, "Value"=w855:string[][])
          n449 = Index Array(array=w855, index (col)=0 ("disabled index (col)")) -> (element=w854:string[])  [unwired: 1 in]
          n450 = call "Find_Number_LineMARVIN.vi"("Test Paragraph"=w858, "error in"=w856, "Row Headers[]"=w854) -> ("error out"=w852:errorcluster, "Line number"=w853:i32)  [unwired: 2 in, 2 out]
          n451 = Build Array (concatenate)(w782, w781) -> (w780:bool[])
          n452 = And Array Elements(Boolean array=w780) -> (logical AND=→"SpeedStopind":bool)
          n453 = Increment(x=w853) -> (x+1=w840:i32)
          n454 = call "PassOrFail (SubVI).vi"("disabled index (col)"=6, "index (row)"=w840, "error in (no error)"=w852, "Boolean"=w781, "Table in"=w838) -> ("error out"=w844:errorcluster)  [unwired: 6 in]
          n455 = property class="Tbl (strict)"(reference=w838, error in=w844) -> (reference out=w849:refnum<vi>, error out=w845:errorcluster, "Value"=w848:string[][])
          n456 = Number To Fractional String(number=w839, precision (6)=i16 2) -> (F-format string=w841:string)  [unwired: 2 in]
          n457 = Replace Array Subset(array=w848, new element=w841, index (row)=w840, index (col)=5 ("disabled index (col)")) -> (w847:string[][])
          n458 = property class="Tbl (strict)"(reference=w849, error in=w845, "Value"=w847) -> (error out=w791:errorcluster)  [unwired: 1 out]
          n459 = property class="VISAName"(reference=w800, error in=w791) -> (error out=w799:errorcluster, "Value"=w809:refnum<visa-resource-name>)  [unwired: 1 out]
          n460 = VISA Write(VISA resource name=w809, write buffer=w801, error in (no error)=w799) -> (error out=w776:errorcluster)  [unwired: 2 out]
          n461 = property on="Start" class="Bool (strict)"(error in=w776, "DisabledEnum"=w778) -> (error out=w777:errorcluster)  [unwired: 1 in, 1 out]
          n462 = property on="Report" class="Bool (strict)"(error in=w777, "DisabledEnum"=w778) -> ()  [unwired: 1 in, 2 out]
        }
        frame "Stop Time" {
          w966 = T13."Enabled" ("Disabled")
          w967 = T13."Disabled and Grayed Out" ("Disabled")
          w954 = "9.Motor Temperature  test in process..." ("Value")
          w963 = "9" ("Test Paragraph")
          # "k15 = 64\nk16 = 128"
          # "K15+Venable"
          # "Deg"
          # "K15 OFF"
          n463 = property on="Stop Button" class="Bool (strict)"("DisabledEnum"=w967) -> ()  [unwired: 2 in, 2 out]
          n464 = Byte Array To String(unsigned byte array=u8[] [75, 0, 4, 2, 0, 64, 0, 0] ("appended array")) -> ()  [unwired: 1 out]
          n465 = property on="Start" class="Bool (strict)"(error in=w971, "DisabledEnum"=w967) -> (error out=w972:errorcluster)  [unwired: 1 in, 1 out]
          n466 = property on="Report" class="Bool (strict)"(error in=w972, "DisabledEnum"=w967) -> (error out=w970:errorcluster)  [unwired: 1 in, 1 out]
          n467 = control-ref of="VISA resource name out"() -> (w992:refnum<vi>)
          n468 = control-ref of="Stop Button"() -> (w957:refnum<vi>)
          n469 = control-ref of="Config_CANAT"() -> (w983:refnum<vi>)
          n470 = control-ref of="UUT"() -> (w984:refnum<vi>)
          n471 = control-ref of="Motor Speed RPM"() -> (w955:refnum<vi>)
          n472 = control-ref of="Pannel User Message"() -> (w988:refnum<vi>)
          n473 = control-ref of="Pannel User Message"() -> (w956:refnum<vi>)
          n474 = Byte Array To String(unsigned byte array=u8[] [75, 0, 4, 2, 0, 0, 0, 0] ("appended array")) -> (string=w995:string)
          n475 = property on="Index" class="Str"() -> ("Value"=w953:string)  [unwired: 2 in, 2 out]
          n476 = Decimal String To Number(string=w953) -> (number=w952:i32)  [unwired: 2 in, 1 out]
          n477 = Subtract(x=w952, y=3 ("x")) -> (x-y=w951:i32)
          n478 = Number To Decimal String(number=w951) -> (decimal integer string=w950:string)  [unwired: 1 in]
          n479 = property class="Str"(reference=w988, error in=w970, "Value"=w954) -> (error out=w987:errorcluster)  [unwired: 1 out]
          n480 = call "Reset old test Values (SubVI).vi"("error in"=w987, "Atr in"=w964, "Test Paragraph"=w963) -> ("error out"=w965:errorcluster)  [unwired: 8 in]
          n481 = call "Table_ScrollaBarMarvin.vi"("error in"=w965, "Line to focus"=w963, "reference in"=w964) -> ("error out"=w1002:errorcluster)  [unwired: 2 out]
          n482 = property class="Tbl (strict)"(reference=w964, error in=w1002) -> (reference out=w986:refnum<vi>, error out=w1001:errorcluster, "Value"=w1000:string[][])
          n483 = Index Array(array=w1000, index (col)=0 ("disabled index (col)")) -> (element=w999:string[])  [unwired: 1 in]
          n484 = call "Find_Number_LineMARVIN.vi"("Test Paragraph"=w963, "error in"=w1001, "Row Headers[]"=w999) -> ("error out"=w997:errorcluster, "Line number"=w977:i32)  [unwired: 2 in, 2 out]
          n485 = call "Table_ScrollaBarMarvin.vi"("error in"=w997, "Line to focus"=w963, "reference in"=w986) -> ("error out"=w980:errorcluster)  [unwired: 2 out]
          n486 = call "CANSendMotorSpeed.vi"("Remote"=FALSE, "error in (no error)"=w980, "Motor Speed RPM"=u16 0, "UUT"=w984, "Cluster in"=w983) -> ("error out"=w979:errorcluster)  [unwired: 6 in]
          n487 = property class="VISAName"(reference=w992, error in=w979) -> (error out=w978:errorcluster, "Value"=w1003:refnum<visa-resource-name>)  [unwired: 1 out]
          n488 = call "Write panel message (SubVI).vi"("rpm"=w955, "Stop"=w957, "error in (no error)"=w978, "Time to wait"=5.0 ("Delay Time (sec)"), "Strin"=w954, "String in"=w956) -> ("error out"=w990:errorcluster)  [unwired: 5 in]
          n489 = call "Time Delay2"("error in (no error)"=w990) -> ("error out"=w961:errorcluster)  [unwired: 10 in]
          n490 = call "Write panel message (SubVI).vi"("rpm"=w955, "PrintTime"=FALSE, "Stop"=w957, "error in (no error)"=w961, "Time to wait"=0.01, "Strin"=w954, "String in"=w956) -> ("error out"=w960:errorcluster)  [unwired: 4 in]
          n491 = call <vilib>:"Clear Errors.vi"("error in (no error)"=w960) -> ("error out"=w962:errorcluster)  [unwired: 5 in, 1 out]
          n492 = property on="Stop Button" class="Bool (strict)"("DisabledEnum"=w966) -> ()  [unwired: 2 in, 2 out]
          n493 = for {
            tunnel: w962 -> [w1054]
            tunnel: dbl[] [1288.0, 1569.0, 1774.0] -> [w1034] mode=indexing
            tunnel: w986 -> [w1048]
            tunnel: w986 -> [w1043]
            tunnel: [w1036] -> w968
            tunnel: w1003 -> [w1042]
            tunnel: w977 -> [w1032]
            tunnel: dbl[] [60.0, 90.0, 110.0] -> [w1029] mode=indexing
            tunnel: [w1027] -> w975 mode=indexing
            tunnel: u32[] [128, 1024, 4096] -> [w1013] mode=indexing
            tunnel: w957 -> [w1010]
            tunnel: w956 -> [w1009]
            tunnel: w955 -> [w1008]
            tunnel: w954 -> [w1005]
            tunnel: w950 -> [w1004]
            i -> [w1026]
            w1035 = 3.0 ("y")
            n494 = Add(x=w1029, y=w1035) -> (x+y=w1039:dbl)
            n495 = Increment(x=w1032) -> (x+1=w1031:i32)
            n496 = Subtract(x=w1029, y=w1035) -> (x-y=w1040:dbl)
            n497 = Add(x=w1031, y=w1026) -> (x+y=w1030:i32)
            n498 = call "DegToDAC (SubVI).vi"("error in (no error)"=w1054, "R2"=10.0, "Numeric"=w1034) -> ("error out"=w1038:errorcluster)  [unwired: 7 in, 1 out]
            n499 = To Unsigned Long Integer(number=w1013) -> (unsigned 32bit integer=w1016:u32)
            n500 = Split Number(x=w1016) -> (hi(x)=w1021:u16, lo(x)=w1022:u16)
            n501 = Split Number(x=w1022) -> (hi(x)=w1020:u8, lo(x)=w1019:u8)
            n502 = Split Number(x=w1021) -> (hi(x)=w1018:u8, lo(x)=w1017:u8)
            n503 = Build Array(u8 75, u8 0 ("element"), u8 4 ("Length"), u8 2, w1019, w1020, w1017, w1018) -> (w1014:u8[])
            n504 = Byte Array To String(unsigned byte array=w1014) -> (string=w1012:string)
            n505 = VISA Write(VISA resource name=w1042, write buffer=w1012, error in (no error)=w1038) -> (error out=w1041:errorcluster)  [unwired: 2 out]
            n506 = call "Write panel message (SubVI).vi"(4:"rpm"=w1008, 5:"rpm"=FALSE ("rpm"), "PrintTime"=TRUE, "Stop"=w1010, "error in (no error)"=w1041, "Time to wait"=3.0, "Strin"=w1005, "String in"=w1009) -> ("error out"=w1033:errorcluster)  [unwired: 3 in]
            n507 = disable-structure shown="Enabled" {
              disable-tunnel: [w1058 w1068] -> w1047
              disable-tunnel: [w1056 w1064] -> w1037
              disable-tunnel: w1033 -> [w1055 w1067]
              disable-tunnel: w1004 -> [_ w1059]
              frame Disabled {
                n508 = control-ref of="Motor Stator Temp."() -> (w1057:refnum<vi>)
                n509 = property class="DigNum (strict)"(reference=w1057, error in=w1055) -> (error out=w1058:errorcluster, "Value"=w1056:dbl)  [unwired: 1 out]
              }
              frame Enabled {
                n510 = for {
                  N: 6 -> [_]
                  tunnel: [w1081] -> w1069 mode=indexing
                  tunnel: w1067 -> [w1077]
                  tunnel: [w1080] -> w1068
                  tunnel: w1059 -> [w1071]
                  n511 = Search and Replace String(input string="TA[2]\r\n" ("write buffer"), search string="2", replace string=w1071) -> (result string=w1070:string)  [unwired: 5 in, 3 out]
                  n512 = property on="VISA resource name" class="VISAName"() -> ("Value"=w1078:refnum<visa-resource-name>)  [unwired: 2 in, 2 out]
                  n513 = call "Time Delay15"("error in (no error)"=w1077) -> ("error out"=w1074:errorcluster)  [unwired: 10 in]
                  n514 = VISA Flush I/O Buffer(VISA resource name=w1078, error in (no error)=w1074) -> (VISA resource name out=w1075:refnum<visa-resource-name>, error out=w1076:errorcluster)  [unwired: 1 in]
                  n515 = call "SerialMarvinMod.vi"("error in (no error)"=w1076, "write buffer"=w1070, "VISA resource name"=w1075) -> ("error out"=w1080:errorcluster, "read buffer"=w1079:string)  [unwired: 7 in]
                  n516 = Fract/Exp String To Number(string=w1079) -> (number=w1081:dbl)  [unwired: 3 in, 1 out]
                }
                n517 = Delete From Array(array=w1069, length=1, index=0) -> (array with subset deleted=w1062:dbl[])  [unwired: 1 out]
                n518 = Add Array Elements(numeric array=w1062) -> (sum=w1065:dbl)
                n519 = Divide(x=w1065, y=5.0) -> (x/y=w1064:dbl)
              }
            }
            n520 = In Range and Coerce(upper limit=w1039, x=w1037, lower limit=w1040) -> (In Range?=w1027:bool)  [unwired: 1 out]
            n521 = call "PassOrFail (SubVI).vi"("disabled index (col)"=6, "index (row)"=w1030, "error in (no error)"=w1047, "Boolean"=w1027, "Table in"=w1043) -> ("error out"=w1051:errorcluster)  [unwired: 6 in]
            n522 = property class="Tbl (strict)"(reference=w1048, error in=w1051) -> (error out=w1044:errorcluster, "Value"=w1053:string[][])  [unwired: 1 out]
            n523 = Number To Fractional String(number=w1037, precision (6)=i16 2) -> (F-format string=w1052:string)  [unwired: 2 in]
            n524 = Replace Array Subset(array=w1053, new element=w1052, index (row)=w1030, index (col)=5 ("disabled index (col)")) -> (w1045:string[][])
            n525 = property class="Tbl (strict)"(reference=w1043, error in=w1044, "Value"=w1045) -> (error out=w1036:errorcluster)  [unwired: 1 out]
          }
          n526 = And Array Elements(Boolean array=w975) -> (logical AND=→"MotorTempind":bool)
          n527 = property class="VISAName"(reference=w992, error in=w968) -> (error out=w994:errorcluster, "Value"=w996:refnum<visa-resource-name>)  [unwired: 1 out]
          n528 = VISA Write(VISA resource name=w996, write buffer=w995, error in (no error)=w994) -> ()  [unwired: 3 out]
          n529 = property on="Start" class="Bool (strict)"(error in=w968, "DisabledEnum"=w966) -> (error out=w969:errorcluster)  [unwired: 1 in, 1 out]
          n530 = property on="Report" class="Bool (strict)"(error in=w969, "DisabledEnum"=w966) -> ()  [unwired: 1 in, 2 out]
        }
        frame "Temp Control" {
          (unwired) dbl[] [5927.0, 11480.0, 15061.0, 11530.0, 6175.0]
          w1097 = T13."Enabled" ("Disabled")
          w1099 = T13."Disabled and Grayed Out" ("Disabled")
          w1082 = "7.5.6" ("Test Paragraph")
          # "K16+Venable"
          # "Deg"
          # "K16 OFF + Venable"
          # "Venable"
          n531 = flat-sequence {
            tunnel: w1095 -> [_]
            frame #0 {
              "TempAlg" <- TRUE
            }
          }
          n532 = control-ref of="Pannel User Message"() -> (w1121:refnum<vi>)
          n533 = property class="Str"(reference=w1121, error in=w1095, "Value"="7.5.6.Temperature controle test") -> (error out=w1120:errorcluster)  [unwired: 1 out]
          n534 = property on="Start" class="Bool (strict)"(error in=w1095, "DisabledEnum"=w1099) -> (error out=w1100:errorcluster)  [unwired: 1 in, 1 out]
          n535 = call "Reset old test Values (SubVI).vi"("error in"=w1120, "Atr in"=w1083, "Test Paragraph"=w1082) -> ("error out"=w1084:errorcluster)  [unwired: 8 in]
          n536 = property on="Report" class="Bool (strict)"(error in=w1100, "DisabledEnum"=w1099) -> ()  [unwired: 1 in, 2 out]
          n537 = call "Table_ScrollaBarMarvin.vi"("error in"=w1084, "Line to focus"=w1082, "reference in"=w1083) -> ("error out"=w1141:errorcluster)  [unwired: 2 out]
          n538 = control-ref of="VISA resource name out"() -> (w1131:refnum<vi>)
          n539 = control-ref of="Config_CANAT"() -> (w1112:refnum<vi>)
          n540 = control-ref of="UUT"() -> (w1113:refnum<vi>)
          n541 = property class="Tbl (strict)"(reference=w1083, error in=w1141) -> (reference out=w1118:refnum<vi>, error out=w1140:errorcluster, "Value"=w1139:string[][])
          n542 = Byte Array To String(unsigned byte array=u8[] [75, 0, 4, 2, 0, 0, 0, 0] ("appended array")) -> (string=w1133:string)
          n543 = Index Array(array=w1139, index (col)=0 ("disabled index (col)")) -> (element=w1138:string[])  [unwired: 1 in]
          n544 = Byte Array To String(unsigned byte array=u8[] [75, 0, 4, 2, 0, 0, 2, 0] ("appended array")) -> (string=w1143:string)
          n545 = Byte Array To String(unsigned byte array=u8[] [75, 0, 4, 2, 0, 128, 2, 0] ("appended array")) -> (string=w1125:string)
          n546 = call "Find_Number_LineMARVIN.vi"("Test Paragraph"=w1082, "error in"=w1140, "Row Headers[]"=w1138) -> ("error out"=w1136:errorcluster, "Line number"=w1128:i32)  [unwired: 2 in, 2 out]
          n547 = call "Table_ScrollaBarMarvin.vi"("error in"=w1136, "Line to focus"=w1082, "reference in"=w1118) -> ("error out"=w1108:errorcluster)  [unwired: 2 out]
          n548 = call "CANSendMotorSpeed.vi"("Remote"=FALSE, "error in (no error)"=w1108, "Motor Speed RPM"=u16 0, "UUT"=w1113, "Cluster in"=w1112) -> ("error out"=w1107:errorcluster)  [unwired: 6 in]
          n549 = property class="VISAName"(reference=w1131, error in=w1107) -> (error out=w1144:errorcluster, "Value"=w1142:refnum<visa-resource-name>)  [unwired: 1 out]
          n550 = VISA Write(VISA resource name=w1142, write buffer=w1143, error in (no error)=w1144) -> (VISA resource name out=w1126:refnum<visa-resource-name>, error out=w1127:errorcluster)  [unwired: 1 out]
          n551 = call "Wait_Sec.vi"("Delay Time (sec)"=2.0, "error out"=w1127) -> ("error in"=w1123:errorcluster)  [unwired: 2 in]
          n552 = VISA Write(VISA resource name=w1126, write buffer=w1125, error in (no error)=w1123) -> (VISA resource name out=w1116:refnum<visa-resource-name>, error out=w1124:errorcluster)  [unwired: 1 out]
          n553 = call "Time Delay"("error in (no error)"=w1124) -> ("error out"=w1109:errorcluster)  [unwired: 10 in]
          n554 = while {
            tunnel: [w1165] -> w1091
            stop <- w1166 stop-if-true
            w1168 = 6050.0 ("y")
            n555 = Random Number (0-1)() -> (number: 0 to 1=w1169:dbl)
            n556 = Multiply(x=w1169, y=w1168) -> (x*y=w1165:dbl)
            n557 = In Range and Coerce(upper limit=w1168, x=w1165, lower limit=5950.0) -> (In Range?=w1166:bool)  [unwired: 1 out]
          }
          n558 = while {
            tunnel: [w1150] -> w1090
            stop <- w1151 stop-if-true
            w1153 = 11550.0 ("y")
            n559 = Random Number (0-1)() -> (number: 0 to 1=w1154:dbl)
            n560 = Multiply(x=w1154, y=w1153) -> (x*y=w1150:dbl)
            n561 = In Range and Coerce(upper limit=w1153, x=w1150, lower limit=11450.0) -> (In Range?=w1151:bool)  [unwired: 1 out]
          }
          n562 = while {
            tunnel: [w1160] -> w1089
            stop <- w1161 stop-if-true
            w1163 = 15050.0 ("y")
            n563 = Random Number (0-1)() -> (number: 0 to 1=w1164:dbl)
            n564 = Multiply(x=w1164, y=w1163) -> (x*y=w1160:dbl)
            n565 = In Range and Coerce(upper limit=w1163, x=w1160, lower limit=14950.0) -> (In Range?=w1161:bool)  [unwired: 1 out]
          }
          n566 = while {
            tunnel: [w1155] -> w1088
            stop <- w1156 stop-if-true
            w1158 = 11550.0 ("y")
            n567 = Random Number (0-1)() -> (number: 0 to 1=w1159:dbl)
            n568 = Multiply(x=w1159, y=w1158) -> (x*y=w1155:dbl)
            n569 = In Range and Coerce(upper limit=w1158, x=w1155, lower limit=11450.0) -> (In Range?=w1156:bool)  [unwired: 1 out]
          }
          n570 = while {
            tunnel: [w1145] -> w1087
            stop <- w1146 stop-if-true
            w1148 = 6050.0 ("y")
            n571 = Random Number (0-1)() -> (number: 0 to 1=w1149:dbl)
            n572 = Multiply(x=w1149, y=w1148) -> (x*y=w1145:dbl)
            n573 = In Range and Coerce(upper limit=w1148, x=w1145, lower limit=5950.0) -> (In Range?=w1146:bool)  [unwired: 1 out]
          }
          n574 = Build Array(w1091, w1090, w1089, w1088, w1087) -> (w1086:dbl[])
          n575 = To Unsigned Word Integer(number=w1086) -> (unsigned 16bit integer=w1085:u16[])
          n576 = for {
            tunnel: w1109 -> [w1212]
            tunnel: dbl[] [1202.0, 1288.0, 1472.0, 1472.0, 1379.0] -> [w1181] mode=indexing
            tunnel: dbl[] [200.0, 200.0, 400.0, 200.0, 200.0] -> [w1211] mode=indexing
            tunnel: w1128 -> [w1209]
            tunnel: w1118 -> [w1202]
            tunnel: w1118 -> [w1187]
            tunnel: [w1201] -> w1117
            tunnel: w1116 -> [w1182]
            tunnel: dbl[] [6000.0, 7000.0, 12200.0, 14500.0, 11100.0] -> [w1173] mode=indexing
            tunnel: dbl[] [50.0, 68.0, 88.0, 80.0, 60.0] -> [w1180] mode=indexing
            tunnel: dbl[] [6000.0, 11400.0, 14900.0, 11600.0, 6200.0] -> [w1178] mode=indexing
            tunnel: [w1175] -> w1104 mode=indexing
            tunnel: [w1174] -> w1103 mode=indexing
            tunnel: w1085 -> [w1172] mode=indexing
            tunnel: dbl[] [57.0, 67.0, 89.0, 79.0, 61.0] -> [w1171] mode=indexing
            i -> [w1177]
            w1193 = 6 ("disabled index (col)")
            n577 = Increment(x=w1209) -> (x+1=w1194:i32)
            n578 = Multiply(x=2, y=w1177) -> (x*y=w1210:i32)
            n579 = Add(x=w1194, y=w1210) -> (x+y=w1196:i32)
            n580 = Increment(x=w1196) -> (x+1=w1192:i32)
            n581 = disable-structure shown="Enabled" {
              disable-tunnel: w1212 -> [w1230 w1400]
              disable-tunnel: w1211 -> [w1229 _]
              disable-tunnel: [w1228 w1398] -> w1191
              disable-tunnel: w1182 -> [w1226 _]
              disable-tunnel: w1181 -> [w1225 _]
              disable-tunnel: w1180 -> [w1224 _]
              disable-tunnel: [w1222 w1400] -> w1179
              disable-tunnel: w1178 -> [w1221 _]
              disable-tunnel: w1177 -> [w1220 _]
              disable-tunnel: [w1218 w1399] -> w1176
              disable-tunnel: [w1217 w1401] -> w1175
              disable-tunnel: [w1216 w1401] -> w1174
              disable-tunnel: w1173 -> [w1213 _]
              disable-tunnel: w1172 -> [_ w1399]
              disable-tunnel: w1171 -> [_ w1398]
              frame Enabled {
                n582 = call <vilib>:"High Resolution Relative Seconds.vi"() -> ("relative seconds"=w1227:dbl)
                n583 = while {
                  tunnel: w1229 -> [w1309]
                  tunnel: w1230 -> [w1321]
                  tunnel: [w1304] -> w1214
                  tunnel: [w1289] -> w1219
                  tunnel: [w1307] -> w1217
                  tunnel: [w1297] -> w1228
                  tunnel: [w1296] -> w1216
                  tunnel: w1220 -> [w1298]
                  tunnel: w1227 -> [w1316]
                  tunnel: w1226 -> [w1312]
                  tunnel: w1213 -> [w1310]
                  shift-right: [w1311] -> _
                  shift-left: w1225 -> [w1295]
                  tunnel: w1224 -> [w1294]
                  shift-right: [w1286] -> _
                  shift-left: "" -> [w1293]
                  tunnel: [w1284] -> w1215
                  stop <- w1318 stop-if-true
                  n584 = control-ref of="Motor Speed RPM"() -> (w1320:refnum<vi>)
                  n585 = control-ref of="Ambient Temperature"() -> (w1322:refnum<vi>)
                  n586 = call <vilib>:"High Resolution Relative Seconds.vi"() -> ("relative seconds"=w1313:dbl)
                  n587 = call <vilib>:"High Resolution Relative Seconds.vi"() -> ("relative seconds"=w1317:dbl)
                  n588 = Subtract(x=w1317, y=w1316) -> (x-y=w1315:dbl)
                  n589 = Greater Or Equal?(x=w1315, y=180.0) -> (x >= y?=w1284:bool)
                  n590 = property on="Stop Button" class="Bool (strict)"() -> ("Value"=w1288:bool)  [unwired: 2 in, 2 out]
                  n591 = First Call?() -> (First Call?: T/F=w1285:bool)
                  n592 = case shown="0, 1, Default" w1298 {
                    tunnel: w1321 -> [w1370 w1377]
                    tunnel: [w1370 w1376] -> w1292
                    tunnel: w1312 -> [_ w1375]
                    tunnel: w1295 -> [_ w1374]
                    tunnel: [TRUE FALSE] -> w1308
                    frame 10 {
                    }
                    frame 0, 1, Default {
                      n593 = call "DegToDAC (SubVI).vi"("error in (no error)"=w1377, "R2"=0.0, "Numeric"=w1374) -> ("error out"=w1378:errorcluster, "output array"=w1373:u8[])  [unwired: 7 in]
                      n594 = Byte Array To String(unsigned byte array=w1373) -> (string=w1379:string)
                      n595 = VISA Write(VISA resource name=w1375, write buffer=w1379, error in (no error)=w1378) -> (error out=w1376:errorcluster)  [unwired: 2 out]
                    }
                  }
                  n596 = property class="DigNum (strict)"(reference=w1322, error in=w1292) -> (error out=w1319:errorcluster, "Value"=w1297:dbl)  [unwired: 1 out]
                  n597 = property class="DigNum (strict)"(reference=w1320, error in=w1319) -> (error out=w1291:errorcluster, "Value"=w1304:dbl)  [unwired: 1 out]
                  n598 = Number To Fractional String(number=w1297, precision (6)=i16 2) -> (F-format string=w1302:string)  [unwired: 2 in]
                  n599 = Number To Fractional String(number=w1304, precision (6)=i16 2) -> (F-format string=w1300:string)  [unwired: 2 in]
                  n600 = Concatenate Strings("\r\n", "Temp: " ("string"), w1302, "  Speed: " ("string"), w1300) -> (w1287:string)
                  n601 = case shown="True" w1285 {
                    tunnel: w1287 -> [w1323 _]
                    tunnel: [w1323 ""] -> w1286
                    frame False {
                    }
                    frame True {
                    }
                  }
                  n602 = case shown="1, 2" w1298 {
                    tunnel: w1297 -> [w1329 w1335 w1338]
                    tunnel: [w1330 w1336 w1339] -> w1296
                    tunnel: w1294 -> [w1328 w1331 _]
                    frame 3, 4 {
                      w1327 = 2.0 ("y")
                      n603 = Add(x=w1327, y=w1328) -> (x+y=w1326:dbl)
                      n604 = Subtract(x=w1328, y=w1327) -> (x-y=w1325:dbl)
                      n605 = In Range and Coerce(upper limit=w1326, x=w1329, lower limit=w1325) -> (In Range?=w1330:bool)  [unwired: 1 out]
                    }
                    frame 1, 2 {
                      w1334 = 2.0 ("y")
                      n606 = Add(x=w1334, y=w1331) -> (x+y=w1333:dbl)
                      n607 = Subtract(x=w1331, y=w1334) -> (x-y=w1332:dbl)
                      n608 = In Range and Coerce(upper limit=w1333, x=w1335, lower limit=w1332) -> (In Range?=w1336:bool)  [unwired: 1 out]
                    }
                    frame Default {
                      n609 = Less Or Equal?(x=w1338, y=65.0) -> (x <= y?=w1339:bool)
                    }
                  }
                  n610 = case shown="3, 4" w1298 {
                    tunnel: [w1345 w1362] -> w1307
                    tunnel: [w1349 w1366] -> w1311
                    tunnel: w1295 -> [w1348 w1365]
                    tunnel: w1304 -> [w1343 w1357]
                    tunnel: w1310 -> [w1342 w1361]
                    tunnel: w1309 -> [w1347 w1364]
                    tunnel: w1291 -> [w1341 w1355]
                    tunnel: [w1341 w1355] -> w1290
                    frame 0, 1, Default {
                      n611 = Add(x=10.0, y=w1348) -> (x+y=w1349:dbl)
                      n612 = Greater Or Equal?(x=w1343, y=w1342) -> (x >= y?=w1344:bool)
                      n613 = Add(x=w1342, y=w1347) -> (x+y=w1350:dbl)
                      n614 = Subtract(x=w1342, y=w1347) -> (x-y=w1351:dbl)
                      n615 = In Range and Coerce(upper limit=w1350, x=w1343, lower limit=w1351) -> (In Range?=w1340:bool)  [unwired: 1 out]
                      n616 = Compound Arithmetic op=OR(w1344, w1340) -> (w1345:bool)
                    }
                    frame 3, 4 {
                      n617 = Subtract(x=w1365, y=10.0 ("x")) -> (x-y=w1366:dbl)
                      n618 = Less Or Equal?(x=w1357, y=w1361) -> (x <= y?=w1359:bool)
                      n619 = Greater Or Equal?(x=w1357, y=5800.0) -> (x >= y?=w1358:bool)
                      n620 = property on="Stop Button" class="Bool (strict)"() -> ("Value"=w1354:bool)  [unwired: 2 in, 2 out]
                      n621 = Not(x=w1354) -> (.not. x?=w1353:bool)
                      n622 = Compound Arithmetic op=AND(w1359, w1358, w1353) -> (w1360:bool)
                      n623 = Add(x=w1361, y=w1364) -> (x+y=w1367:dbl)
                      n624 = Subtract(x=w1361, y=w1364) -> (x-y=w1368:dbl)
                      n625 = In Range and Coerce(upper limit=w1367, x=w1357, lower limit=w1368) -> (In Range?=w1352:bool)  [unwired: 1 out]
                      n626 = Compound Arithmetic op=OR(w1360, w1352) -> (w1362:bool)
                    }
                  }
                  n627 = Compound Arithmetic op=OR(w1307, w1308, w1284, w1288) -> (w1318:bool)
                  n628 = while {
                    tunnel: w1290 -> [w1382]
                    tunnel: w1313 -> [w1396]
                    tunnel: [w1382] -> w1289
                    tunnel: w1293 -> [w1383]
                    stop <- w1381 stop-if-true
                    n629 = control-ref of="Pannel User Message"() -> (w1384:refnum<vi>)
                    n630 = property on="Stop Button" class="Bool (strict)"() -> ("Value"=w1380:bool)  [unwired: 2 in, 2 out]
                    n631 = call <vilib>:"High Resolution Relative Seconds.vi"() -> ("relative seconds"=w1397:dbl)
                    n632 = Subtract(x=w1397, y=w1396) -> (x-y=w1394:dbl)
                    n633 = Subtract(x=4.0, y=w1394) -> (x-y=w1389:dbl)
                    n634 = Less Or Equal To 0?(x=w1389) -> (x <= 0?=w1395:bool)
                    n635 = Compound Arithmetic op=OR(w1395, w1380) -> (w1381:bool)
                    n636 = Number To Fractional String(number=w1389, precision (6)=i16 2) -> (F-format string=w1391:string)  [unwired: 2 in]
                    n637 = Concatenate Strings("7.5.6.Temperature controle test" ("Value"), "\r\n", "Time to wait: " ("Value"), w1391, "  Sec." ("string"), w1383) -> (w1386:string)
                    n638 = property class="Str"(reference=w1384, "Value"=w1386) -> ()  [unwired: 1 in, 2 out]
                  }
                }
                n639 = case shown="False" w1215 {
                  tunnel: [w1237 w1283] -> w1222
                  tunnel: w1221 -> [w1236 _]
                  tunnel: w1220 -> [w1235 _]
                  tunnel: w1219 -> [w1234 w1283]
                  tunnel: [w1231 w1282] -> w1218
                  tunnel: w1214 -> [_ w1282]
                  frame False {
                    n640 = flat-sequence {
                      tunnel: w1234 -> [w1239]
                      tunnel: [w1239] -> w1233
                      tunnel: [w1238] -> w1232
                      frame #0 {
                        n641 = call <vilib>:"High Resolution Relative Seconds.vi"() -> ("relative seconds"=w1238:dbl)
                      }
                    }
                    n642 = while {
                      tunnel: w1233 -> [w1262]
                      tunnel: [w1261] -> w1237
                      tunnel: w1236 -> [w1260]
                      tunnel: w1235 -> [w1259]
                      tunnel: w1232 -> [w1254]
                      tunnel: [w1248] -> w1231
                      stop <- w1257 stop-if-true
                      w1244 = 120.0 ("y")
                      n643 = control-ref of="Motor Speed RPM"() -> (w1263:refnum<vi>)
                      n644 = control-ref of="Pannel User Message"() -> (w1253:refnum<vi>)
                      n645 = property class="DigNum (strict)"(reference=w1263, error in=w1262) -> (error out=w1261:errorcluster, "Value"=w1248:dbl)  [unwired: 1 out]
                      n646 = property on="Stop Button" class="Bool (strict)"() -> ("Value"=w1246:bool)  [unwired: 2 in, 2 out]
                      n647 = call <vilib>:"High Resolution Relative Seconds.vi"() -> ("relative seconds"=w1255:dbl)
                      n648 = Subtract(x=w1255, y=w1254) -> (x-y=w1243:dbl)
                      n649 = Number To Fractional String(number=w1248, precision (6)=i16 2) -> (F-format string=w1250:string)  [unwired: 2 in]
                      n650 = Subtract(x=w1244, y=w1243) -> (x-y=w1242:dbl)
                      n651 = Number To Fractional String(number=w1242, precision (6)=i16 2) -> (F-format string=w1240:string)  [unwired: 2 in]
                      n652 = Concatenate Strings("7.5.6.Temperature controle test\n" ("string"), "Motor speed [rpm]: " ("string"), w1250, "\nTimeout [sec]: " ("string"), w1240) -> (w1247:string)
                      n653 = property class="Str"(reference=w1253, "Value"=w1247) -> ()  [unwired: 1 in, 2 out]
                      n654 = Greater Or Equal?(x=w1243, y=w1244) -> (x >= y?=w1256:bool)
                      n655 = case shown="3, 4" w1259 {
                        tunnel: w1248 -> [w1265 w1271 w1277]
                        tunnel: [w1267 w1273 w1279] -> w1258
                        tunnel: w1260 -> [w1268 w1274 _]
                        frame 3, 4 {
                          n656 = Greater Or Equal?(x=w1265, y=5700.0) -> (x >= y?=w1266:bool)
                          n657 = Less Or Equal?(x=w1265, y=w1268) -> (x <= y?=w1269:bool)
                          n658 = And(x=w1266, y=w1269) -> (x .and. y?=w1267:bool)
                        }
                        frame 1, 2 {
                          n659 = Greater Or Equal?(x=w1271, y=w1274) -> (x >= y?=w1275:bool)
                          n660 = Less Or Equal?(x=w1271, y=15300.0) -> (x <= y?=w1272:bool)
                          n661 = And(x=w1275, y=w1272) -> (x .and. y?=w1273:bool)
                        }
                        frame Default {
                          n662 = Greater Or Equal?(x=w1277, y=5800.0) -> (x >= y?=w1281:bool)
                          n663 = Less Or Equal?(x=w1277, y=6200.0) -> (x <= y?=w1278:bool)
                          n664 = And(x=w1281, y=w1278) -> (x .and. y?=w1279:bool)
                        }
                      }
                      n665 = Compound Arithmetic op=OR(w1258, w1256, w1246) -> (w1257:bool)
                    }
                  }
                  frame True {
                  }
                }
              }
              frame Disabled {
                w1401 = TRUE ("Boolean")
              }
            }
            n666 = call "PassOrFail (SubVI).vi"("disabled index (col)"=w1193, "index (row)"=w1196, "error in (no error)"=w1179, "Boolean"=w1175, "Table in"=w1187) -> ("error out"=w1206:errorcluster)  [unwired: 6 in]
            n667 = property class="Tbl (strict)"(reference=w1202, error in=w1206) -> (reference out=w1205:refnum<vi>, error out=w1189:errorcluster, "Value"=w1208:string[][])
            n668 = Number To Fractional String(number=w1191, precision (6)=i16 2) -> (F-format string=w1198:string)  [unwired: 2 in]
            n669 = Number To Fractional String(number=w1176, precision (6)=i16 2) -> (F-format string=w1207:string)  [unwired: 2 in]
            n670 = Replace Array Subset(array=w1208, new element=w1207, index (row)=w1196, index (col)=5 ("disabled index (col)")) -> (w1190:string[][])
            n671 = property class="Tbl (strict)"(reference=w1187, error in=w1189, "Value"=w1190) -> (reference out=w1185:refnum<vi>, error out=w1188:errorcluster)
            n672 = call "PassOrFail (SubVI).vi"("disabled index (col)"=w1193, "index (row)"=w1192, "error in (no error)"=w1188, "Boolean"=w1174, "Table in"=w1187) -> ("error out"=w1186:errorcluster)  [unwired: 6 in]
            n673 = property class="Tbl (strict)"(reference=w1185, error in=w1186) -> (error out=w1183:errorcluster, "Value"=w1184:string[][])  [unwired: 1 out]
            n674 = Replace Array Subset(array=w1184, new element=w1198, index (row)=w1192, index (col)=5 ("disabled index (col)")) -> (w1197:string[][])
            n675 = property class="Tbl (strict)"(reference=w1205, error in=w1183, "Value"=w1197) -> (error out=w1201:errorcluster)  [unwired: 1 out]
          }
          n676 = property class="VISAName"(reference=w1131, error in=w1117) -> (error out=w1096:errorcluster, "Value"=w1134:refnum<visa-resource-name>)  [unwired: 1 out]
          n677 = VISA Write(VISA resource name=w1134, write buffer=w1133, error in (no error)=w1096) -> ()  [unwired: 3 out]
          n678 = property on="Start" class="Bool (strict)"(error in=w1096, "DisabledEnum"=w1097) -> (error out=w1098:errorcluster)  [unwired: 1 in, 1 out]
          n679 = property on="Report" class="Bool (strict)"(error in=w1098, "DisabledEnum"=w1097) -> (error out=w1094:errorcluster)  [unwired: 1 in, 1 out]
          n680 = property on="TempAlg" class="Bool (strict)"(error in=w1094, "Value"=FALSE ("TempAlg")) -> ()  [unwired: 1 in, 2 out]
          n681 = Build Array (concatenate)(w1104, w1103) -> (w1102:bool[])
          n682 = And Array Elements(Boolean array=w1102) -> (logical AND=→"TempControlind":bool)
        }
        frame "Burn in" {
          w1411 = TRUE ("rpm")
          w1413 = FALSE ("PrintTime")
          w1429 = T13."Enabled" ("Disabled")
          w1432 = T13."Disabled and Grayed Out" ("Disabled")
          (unwired) "EP=1r\nVC=15100\r\n" ("write buffer")
          (unwired) dbl[] [60.0, 60.0, 60.0]
          w1497 = 13.0 ("y")
          w1496 = 25.0 ("x")
          w1495 = 2 ("disabled index (col)")
          w1502 = 6 ("disabled index (col)")
          w1521 = 400.0 ("y")
          w1520 = 15100.0 ("x")
          w1427 = "7.5.7.Burn-in test in process" ("Value")
          w1406 = "7.5.7" ("Test Paragraph")
          # "k16+Venable"
          # "K15 + Venable + 90deg OFF"
          # "Venable"
          n683 = Byte Array To String(unsigned byte array=u8[] [75, 0, 4, 2, 0, 0, 2, 0] ("appended array")) -> ()  [unwired: 1 out]
          n684 = property on="Start" class="Bool (strict)"(error in=w1431, "DisabledEnum"=w1432) -> (error out=w1433:errorcluster)  [unwired: 1 in, 1 out]
          n685 = property on="Report" class="Bool (strict)"(error in=w1433, "DisabledEnum"=w1432) -> (error out=w1404:errorcluster)  [unwired: 1 in, 1 out]
          n686 = control-ref of="Pannel User Message"() -> (w1529:refnum<vi>)
          n687 = control-ref of="VISA resource name out"() -> (w1534:refnum<vi>)
          n688 = Concatenate Strings(w1427, "\nFull speed operation" ("string")) -> (w1426:string)
          n689 = property class="Str"(reference=w1529, error in=w1404, "Value"=w1427) -> (reference out=w1418:refnum<vi>, error out=w1460:errorcluster)
          n690 = control-ref of="Stop Button"() -> (w1419:refnum<vi>)
          n691 = control-ref of="Config_CANAT"() -> (w1447:refnum<vi>)
          n692 = control-ref of="Config_CANAT"() -> (w1455:refnum<vi>)
          n693 = control-ref of="Config_CANAT"() -> (w1462:refnum<vi>)
          n694 = control-ref of="UUT"() -> (w1448:refnum<vi>)
          n695 = control-ref of="Power transistor Heat sink Temp."() -> (w1498:refnum<vi>)
          n696 = control-ref of="UUT"() -> (w1454:refnum<vi>)
          n697 = control-ref of="UUT"() -> (w1463:refnum<vi>)
          n698 = control-ref of="Motor Speed RPM"() -> (w1527:refnum<vi>)
          n699 = control-ref of="Motor Speed RPM"() -> (w1412:refnum<vi>)
          n700 = Byte Array To String(unsigned byte array=u8[] [75, 0, 4, 2, 0, 0, 0, 0] ("appended array")) -> (string=w1537:string)
          n701 = Add(x=w1520, y=w1521) -> (x+y=w1522:dbl)
          n702 = Add(x=w1496, y=w1497) -> (x+y=w1499:dbl)
          n703 = property on="UUT" class="Str"() -> ("Value"=w1410:string)  [unwired: 2 in, 2 out]
          n704 = Equal?(x=w1410, y="EBAY") -> (x = y?=w1408:bool)
          n705 = case shown="False" w1408 {
            tunnel: [28.0 ("x") 50.0 ("x")] -> w1513
            tunnel: [5.0 ("y") 7.0 ("y")] -> w1512
            frame False {
            }
            frame True {
            }
          }
          n706 = Add(x=w1513, y=w1512) -> (x+y=w1511:dbl)
          n707 = Subtract(x=w1520, y=w1521) -> (x-y=w1523:dbl)
          n708 = Subtract(x=w1496, y=w1497) -> (x-y=w1500:dbl)
          n709 = Byte Array To String(unsigned byte array=u8[] [75, 0, 4, 2, 0, 0, 2, 0] ("appended array")) -> (string=w1548:string)
          n710 = Subtract(x=w1513, y=w1512) -> (x-y=w1510:dbl)
          n711 = property on="CurrentOffset" class="DigNum (strict)"() -> ("Value"=w1440:dbl)  [unwired: 2 in, 2 out]
          n712 = disable-structure shown="Enabled" {
            disable-tunnel: w1463 -> [w1655 _]
            disable-tunnel: w1462 -> [w1654 _]
            disable-tunnel: u16 0 ("Motor Speed RPM") -> [w1652 _]
            disable-tunnel: w1460 -> [w1651 w1656]
            disable-tunnel: [w1650 w1656] -> w1459
            frame Disabled {
              n713 = call "CANSendMotorSpeed.vi"("Remote"=FALSE, "error in (no error)"=w1651, "Motor Speed RPM"=w1652, "UUT"=w1655, "Cluster in"=w1654) -> ("error out"=w1650:errorcluster)  [unwired: 6 in]
            }
            frame Enabled {
            }
          }
          n714 = call "Reset old test Values (SubVI).vi"("error in"=w1459, "Atr in"=w1405, "Test Paragraph"=w1406) -> ("error out"=w1407:errorcluster)  [unwired: 8 in]
          n715 = call "Table_ScrollaBarMarvin.vi"("error in"=w1407, "Line to focus"=w1406, "reference in"=w1405) -> ("error out"=w1546:errorcluster)  [unwired: 2 out]
          n716 = property class="Tbl (strict)"(reference=w1405, error in=w1546) -> (reference out=w1476:refnum<vi>, error out=w1545:errorcluster, "Value"=w1544:string[][])
          n717 = Index Array(array=w1544, index (col)=0 ("disabled index (col)")) -> (element=w1543:string[])  [unwired: 1 in]
          n718 = call "Find_Number_LineMARVIN.vi"("Test Paragraph"=w1406, "error in"=w1545, "Row Headers[]"=w1543) -> ("error out"=w1541:errorcluster, "Line number"=w1515:i32)  [unwired: 2 in, 2 out]
          n719 = call "Table_ScrollaBarMarvin.vi"("error in"=w1541, "Line to focus"=w1406, "reference in"=w1476) -> ("error out"=w1540:errorcluster)  [unwired: 2 out]
          n720 = property class="VISAName"(reference=w1534, error in=w1540) -> (error out=w1549:errorcluster, "Value"=w1547:refnum<visa-resource-name>)  [unwired: 1 out]
          n721 = VISA Write(VISA resource name=w1547, write buffer=w1548, error in (no error)=w1549) -> (VISA resource name out=w1532:refnum<visa-resource-name>, error out=w1533:errorcluster)  [unwired: 1 out]
          n722 = call "Wait_Sec.vi"("Delay Time (sec)"=0.0, "error out"=w1533) -> ("error in"=w1443:errorcluster)  [unwired: 2 in]
          n723 = property class="DigNum (strict)"(reference=w1498, error in=w1443) -> (error out=w1442:errorcluster, "Value"=w1491:dbl)  [unwired: 1 out]
          n724 = In Range and Coerce(upper limit=w1499, x=w1491, lower limit=w1500) -> (In Range?=w1437:bool)  [unwired: 1 out]
          n725 = Number To Fractional String(number=w1491, precision (6)=i16 2) -> (F-format string=w1506:string)  [unwired: 2 in]
          n726 = call "Write panel message (SubVI).vi"("rpm"=w1412, "Stop"=w1419, "error in (no error)"=w1442, "Time to wait"=10.0 ("Delay Time (sec)"), "Strin"=w1427, "String in"=w1418) -> ("error out"=w1457:errorcluster)  [unwired: 5 in]
          n727 = call "CANSendMotorSpeed.vi"("Remote"=TRUE, "error in (no error)"=w1457, "Motor Speed RPM"=u16 15100, "UUT"=w1454, "Cluster in"=w1455) -> ("error out"=w1456:errorcluster)  [unwired: 6 in]
          n728 = call "Write panel message (SubVI).vi"(4:"rpm"=w1412, 5:"rpm"=w1411, "PrintTime"=w1413, "Stop"=w1419, "error in (no error)"=w1456, "Time to wait"=30.0 ("Delay Time (sec)"), "Strin"=w1426, "String in"=w1418) -> ("error out"=w1526:errorcluster)  [unwired: 3 in]
          n729 = call "Write panel message (SubVI).vi"(4:"rpm"=w1412, 5:"rpm"=w1411, "PrintTime"=w1413, "Stop"=w1419, "error in (no error)"=w1526, "Time to wait"=1.0, "Strin"="7.5.7.Burn-in test in process.\nDC current measure.", "String in"=w1418) -> ("error out"=w1420:errorcluster)  [unwired: 3 in]
          n730 = Add(x=w1491, y=25.0) -> (x+y=w1485:dbl)
          n731 = Number To Fractional String(number=w1485, precision (6)=i16 2) -> (F-format string=w1489:string)  [unwired: 2 in]
          n732 = Concatenate Strings("< " ("string"), w1489) -> (w1488:string)
          n733 = Increment(x=w1515) -> (x+1=w1503:i32)
          n734 = Increment(x=w1503) -> (x+1=w1501:i32)
          n735 = Increment(x=w1501) -> (x+1=w1482:i32)
          n736 = Increment(x=w1482) -> (x+1=w1494:i32)
          n737 = Increment(x=w1494) -> (x+1=w1493:i32)
          n738 = Increment(x=w1493) -> (x+1=w1481:i32)
          n739 = for {
            N: 10 -> [_]
            tunnel: w1532 -> [w1575]
            tunnel: [w1566] -> w1415 mode=indexing
            tunnel: w1420 -> [w1574]
            tunnel: [w1567] -> w1524
            stop <- w1564 stop-if-true
            # "Get Current by ADC (2)"
            n740 = Byte Array To String(unsigned byte array=u8[] [75, 0, 4, 17, 0, 0, 0, 0] ("appended array")) -> (string=w1573:string)
            n741 = call "Time Delay8"("error in (no error)"=w1574) -> ("error out"=w1565:errorcluster)  [unwired: 10 in]
            n742 = VISA Write(VISA resource name=w1575, write buffer=w1573, error in (no error)=w1565) -> (VISA resource name out=w1571:refnum<visa-resource-name>, error out=w1570:errorcluster)  [unwired: 1 out]
            n743 = property on="Stop Button" class="Bool (strict)"() -> ("Value"=w1564:bool)  [unwired: 2 in, 2 out]
            n744 = flat-sequence {
              tunnel: w1570 -> [w1577]
              tunnel: [w1577] -> w1569
              tunnel: [w1576] -> w1568
              frame #0 {
                n745 = call <vilib>:"High Resolution Relative Seconds.vi"() -> ("relative seconds"=w1576:dbl)
              }
            }
            n746 = while {
              tunnel: w1571 -> [w1590]
              tunnel: w1569 -> [w1589]
              tunnel: [w1588] -> _
              tunnel: [w1587] -> w1567
              tunnel: w1568 -> [w1585]
              tunnel: [w1579] -> w1566
              stop <- w1581 stop-if-true
              n747 = call <vilib>:"High Resolution Relative Seconds.vi"() -> ("relative seconds"=w1586:dbl)
              n748 = Subtract(x=w1586, y=w1585) -> (x-y=w1584:dbl)
              n749 = Greater Or Equal?(x=w1584, y=10.0) -> (x >= y?=w1582:bool)
              n750 = property on="Stop Button" class="Bool (strict)"() -> ("Value"=w1578:bool)  [unwired: 2 in, 2 out]
              n751 = VISA Read(VISA resource name=w1590, byte count=u32 1, error in (no error)=w1589) -> (VISA resource name out=w1592:refnum<visa-resource-name>, read buffer=w1593:string, error out=w1591:errorcluster)  [unwired: 1 out]
              n752 = String To Byte Array(string=w1593) -> (unsigned byte array=w1596:u8[])
              n753 = Index Array(array=w1596, index=0) -> (element=w1594:u8)
              n754 = case shown="75" w1594 {
                tunnel: [w1601 w1605] -> w1587
                tunnel: w1592 -> [w1600 w1614]
                tunnel: w1591 -> [w1601 w1613]
                tunnel: [w1600 w1606] -> w1588
                tunnel: [u32 9999 w1603] -> w1579
                tunnel: [FALSE w1602] -> w1580
                frame 0, Default {
                }
                frame 75 {
                  n755 = VISA Read(VISA resource name=w1614, byte count=u32 3, error in (no error)=w1613) -> (VISA resource name out=w1609:refnum<visa-resource-name>, read buffer=w1617:string, error out=w1608:errorcluster)  [unwired: 1 out]
                  n756 = String To Byte Array(string=w1617) -> (unsigned byte array=w1607:u8[])
                  n757 = Index Array(array=w1607, index #1=0 ("index")) -> (element #1=w1612:u8, element #2=w1610:u8)  [unwired: 2 in, 1 out]
                  n758 = Equal?(x=u8 0, y=w1612) -> (x = y?=w1611:bool)
                  n759 = case shown="True" w1611 {
                    tunnel: [w1620 w1627] -> w1605
                    tunnel: w1610 -> [_ w1634]
                    tunnel: w1609 -> [w1621 w1633]
                    tunnel: w1608 -> [w1620 w1632]
                    tunnel: w1607 -> [_ w1631]
                    tunnel: [w1621 w1629] -> w1606
                    tunnel: [u32 9999 w1623] -> w1603
                    tunnel: [FALSE w1622] -> w1602
                    frame False {
                    }
                    frame True {
                      n760 = VISA Read(VISA resource name=w1633, byte count=w1634, error in (no error)=w1632) -> (VISA resource name out=w1629:refnum<visa-resource-name>, read buffer=w1628:string, error out=w1627:errorcluster)  [unwired: 1 out]
                      n761 = String To Byte Array(string=w1628) -> (unsigned byte array=w1630:u8[])
                      n762 = Insert Into Array(array=w1631, new element=w1630) -> (w1624:u8[])  [unwired: 1 in]
                      n763 = Index Array(array=w1624, index #1=0 ("index")) -> (element #3=w1625:u8)  [unwired: 2 in, 2 out]
                      n764 = case shown="15..19" w1625 {
                        tunnel: w1624 -> [_ w1648]
                        tunnel: [u32 9999 w1637] -> w1623
                        tunnel: [FALSE w1638] -> w1622
                        frame 0, Default {
                        }
                        frame 15..19 {
                          n765 = Index Array(array=w1648, index #1=3 ("index")) -> (element #1=w1647:u8, element #2=w1646:u8, element #3=w1645:u8, element #4=w1644:u8)  [unwired: 3 in]
                          n766 = Join Numbers(hi=w1644, lo=w1645) -> ((hi.lo)=w1642:u16)
                          n767 = Join Numbers(hi=w1646, lo=w1647) -> ((hi.lo)=w1643:u16)
                          n768 = Join Numbers(hi=w1642, lo=w1643) -> ((hi.lo)=w1640:u32)
                          n769 = Multiply(x=0.02003173828125, y=w1640) -> (x*y=w1637:dbl)
                          n770 = Greater Or Equal?(x=w1637, y=40.0) -> (x >= y?=w1638:bool)
                        }
                      }
                    }
                  }
                }
              }
              n771 = Compound Arithmetic op=OR(w1578, w1582, w1580) -> (w1581:bool)
            }
          }
          n772 = call <vilib>:"Clear Errors.vi"("error in (no error)"=w1524) -> ("error out"=w1451:errorcluster)  [unwired: 5 in, 1 out]
          n773 = property class="DigNum (strict)"(reference=w1527, error in=w1451) -> (error out=w1444:errorcluster, "Value"=w1486:dbl)  [unwired: 1 out]
          n774 = In Range and Coerce(upper limit=w1522, x=w1486, lower limit=w1523) -> (In Range?=w1438:bool)  [unwired: 1 out]
          n775 = Number To Fractional String(number=w1486, precision (6)=i16 2) -> (F-format string=w1507:string)  [unwired: 2 in]
          n776 = property class="Tbl (strict)"(reference=w1476, error in=w1444) -> (reference out=w1514:refnum<vi>, error out=w1471:errorcluster, "Value"=w1519:string[][])
          n777 = for {
            tunnel: w1415 -> [_] mode=indexing
            shift-right: [w1554] -> w1414
            shift-left: w1415 -> [w1557]
            n778 = Search 1D Array(1D array=w1557, element=9999.0) -> (index of element=w1555:i32)  [unwired: 1 in]
            n779 = Greater Or Equal To 0?(x=w1555) -> (x >= 0?=w1556:bool)
            n780 = case shown="True" w1556 {
              tunnel: w1557 -> [w1559 w1562]
              tunnel: w1555 -> [_ w1561]
              tunnel: [w1559 w1560] -> w1554
              frame False {
              }
              frame True {
                n781 = Delete From Array(array=w1562, length=1, index=w1561) -> (deleted portion=w1560:dbl[])  [unwired: 1 out]
              }
            }
          }
          n782 = Add Array Elements(numeric array=w1414) -> (sum=w1423:dbl)
          n783 = Divide(x=w1423, y=10.0) -> (x/y=w1422:dbl)
          n784 = Subtract(x=w1422, y=w1440) -> (x-y=w1441:dbl)
          n785 = In Range and Coerce(upper limit=w1511, x=w1441, lower limit=w1510) -> (In Range?=w1436:bool)  [unwired: 1 out]
          n786 = Number To Fractional String(number=w1441, precision (6)=i16 2) -> (F-format string=w1518:string)  [unwired: 2 in]
          n787 = Replace Array Subset(array=w1519, new element=w1518, index (row)=w1503, index (col)=5 ("disabled index (col)")) -> (w1479:string[][])
          n788 = property class="Tbl (strict)"(reference=w1476, error in=w1471, "Value"=w1479) -> (reference out=w1478:refnum<vi>, error out=w1470:errorcluster)
          n789 = call "PassOrFail (SubVI).vi"("disabled index (col)"=w1502, "index (row)"=w1503, "error in (no error)"=w1470, "Boolean"=w1436, "Table in"=w1514) -> ("error out"=w1469:errorcluster)  [unwired: 6 in]
          n790 = property class="Tbl (strict)"(reference=w1478, error in=w1469) -> (reference out=w1474:refnum<vi>, error out=w1468:errorcluster, "Value"=w1477:string[][])
          n791 = Replace Array Subset(array=w1477, new element=w1507, index (row)=w1501, index (col)=5 ("disabled index (col)")) -> (w1475:string[][])
          n792 = property class="Tbl (strict)"(reference=w1474, error in=w1468, "Value"=w1475) -> (reference out=w1473:refnum<vi>, error out=w1467:errorcluster)
          n793 = call "PassOrFail (SubVI).vi"("disabled index (col)"=w1502, "index (row)"=w1501, "error in (no error)"=w1467, "Boolean"=w1438, "Table in"=w1476) -> ("error out"=w1466:errorcluster)  [unwired: 6 in]
          n794 = property class="Tbl (strict)"(reference=w1473, error in=w1466) -> (error out=w1465:errorcluster, "Value"=w1472:string[][])  [unwired: 1 out]
          n795 = Replace Array Subset(array=w1472, new element #1=w1506, index (row) #1=w1482, index (col) #1=5 ("disabled index (col)"), new element #2=w1488, index (row) #2=w1494, index (col) #2=w1495, new element #3=w1488, index (row) #3=w1493, index (col) #3=w1495, new element #4=w1488, index (row) #4=w1481, index (col) #4=w1495) -> (w1504:string[][])
          n796 = property class="Tbl (strict)"(reference=w1476, error in=w1465, "Value"=w1504) -> (error out=w1464:errorcluster)  [unwired: 1 out]
          n797 = call "PassOrFail (SubVI).vi"("disabled index (col)"=w1502, "index (row)"=w1482, "error in (no error)"=w1464, "Boolean"=w1437, "Table in"=w1476) -> ("error out"=w1403:errorcluster)  [unwired: 6 in]
          n798 = property on="Stop Burn-in" class="Bool"(error in=w1403, "Visible"=TRUE) -> (error out=w1402:errorcluster)  [unwired: 1 in, 1 out]
          n799 = for {
            tunnel: w1402 -> [w1681]
            tunnel: dbl[] [600.0, 600.0, 600.0] -> [w1678] mode=indexing
            tunnel: w1485 -> [w1675]
            tunnel: w1482 -> [w1672]
            tunnel: w1405 -> [w1666]
            tunnel: [w1658] -> w1446
            tunnel: [w1657] -> w1439 mode=indexing
            i -> [w1671]
            n800 = control-ref of="Power transistor Heat sink Temp."() -> (w1677:refnum<vi>)
            n801 = Increment(x=w1671) -> (x+1=w1670:i32)
            n802 = Add(x=w1672, y=w1670) -> (x+y=w1664:i32)
            n803 = flat-sequence {
              tunnel: [w1705] -> _
              tunnel: [w1705] -> w1680
              tunnel: [w1706] -> w1679
              tunnel: w1681 -> [w1705]
              frame #0 {
                n804 = call <vilib>:"High Resolution Relative Seconds.vi"() -> ("relative seconds"=w1706:dbl)
              }
            }
            n805 = while {
              tunnel: w1680 -> [w1700]
              tunnel: w1679 -> [w1703]
              tunnel: w1678 -> [w1694]
              tunnel: [w1691] -> w1676
              stop <- w1690 stop-if-true
              w1688 = i16 2 ("precision (6)")
              n806 = control-ref of="Pannel User Message"() -> (w1699:refnum<vi>)
              n807 = call <vilib>:"High Resolution Relative Seconds.vi"() -> ("relative seconds"=w1704:dbl)
              n808 = property on="Stop Button" class="Bool (strict)"() -> ("Value"=w1689:bool)  [unwired: 2 in, 2 out]
              n809 = Subtract(x=w1704, y=w1703) -> (x-y=w1693:dbl)
              n810 = Greater Or Equal?(x=w1693, y=w1694) -> (x >= y?=w1702:bool)
              n811 = Compound Arithmetic op=OR(w1689, "Stop Burn-in", w1702) -> (w1690:bool)
              n812 = Subtract(x=w1694, y=w1693) -> (x-y=w1695:dbl)
              n813 = Number To Fractional String(number=w1695, precision (6)=i16 2) -> (F-format string=w1696:string)  [unwired: 2 in]
              n814 = property on="Power transistor Heat sink Temp." class="DigNum (strict)"() -> ("Value"=w1687:dbl)  [unwired: 2 in, 2 out]
              n815 = Number To Fractional String(number=w1687, precision (6)=w1688) -> (F-format string=w1684:string)  [unwired: 2 in]
              n816 = property on="Motor Speed RPM" class="DigNum (strict)"() -> ("Value"=w1686:dbl)  [unwired: 2 in, 2 out]
              n817 = Number To Fractional String(number=w1686, precision (6)=w1688) -> (F-format string=w1682:string)  [unwired: 2 in]
              n818 = Concatenate Strings("Remained Time: " ("string"), w1696, "\nPCB Temp. [Deg]: " ("string"), w1684, "\nMotor speed [rpm]: " ("string"), w1682) -> (w1692:string)
              n819 = property class="Str"(reference=w1699, error in=w1700, "Value"=w1692) -> (error out=w1691:errorcluster)  [unwired: 1 out]
            }
            n820 = property class="DigNum (strict)"(reference=w1677, error in=w1676) -> (error out=w1667:errorcluster, "Value"=w1668:dbl)  [unwired: 1 out]
            n821 = Less Or Equal?(x=w1668, y=w1675) -> (x <= y?=w1657:bool)
            n822 = property class="Tbl (strict)"(reference=w1666, error in=w1667) -> (reference out=w1661:refnum<vi>, error out=w1660:errorcluster, "Value"=w1663:string[][])
            n823 = Number To Fractional String(number=w1668, precision (6)=i16 2) -> (F-format string=w1669:string)  [unwired: 2 in]
            n824 = Replace Array Subset(array=w1663, new element=w1669, index (row)=w1664, index (col)=5 ("disabled index (col)")) -> (w1662:string[][])
            n825 = property class="Tbl (strict)"(reference=w1661, error in=w1660, "Value"=w1662) -> (error out=w1659:errorcluster)  [unwired: 1 out]
            n826 = call "PassOrFail (SubVI).vi"("disabled index (col)"=6, "index (row)"=w1664, "error in (no error)"=w1659, "Boolean"=w1657, "Table in"=w1661) -> ("error out"=w1658:errorcluster)  [unwired: 6 in]
          }
          n827 = call "CANSendMotorSpeed.vi"("Remote"=FALSE, "error in (no error)"=w1446, "Motor Speed RPM"=u16 0, "UUT"=w1448, "Cluster in"=w1447) -> ("error out"=w1445:errorcluster)  [unwired: 6 in]
          n828 = property on="Stop Burn-in" class="Bool"(error in=w1445, "Visible"=FALSE) -> (error out=w1428:errorcluster)  [unwired: 1 in, 1 out]
          n829 = property class="VISAName"(reference=w1534, error in=w1428) -> (error out=w1536:errorcluster, "Value"=w1538:refnum<visa-resource-name>)  [unwired: 1 out]
          n830 = VISA Write(VISA resource name=w1538, write buffer=w1537, error in (no error)=w1536) -> ()  [unwired: 3 out]
          n831 = property on="Start" class="Bool (strict)"(error in=w1428, "DisabledEnum"=w1429) -> (error out=w1430:errorcluster)  [unwired: 1 in, 1 out]
          n832 = property on="Report" class="Bool (strict)"(error in=w1430, "DisabledEnum"=w1429) -> ()  [unwired: 1 in, 2 out]
          n833 = Build Array (concatenate)(w1439, w1438, w1437, w1436) -> (w1435:bool[])
          n834 = And Array Elements(Boolean array=w1435) -> (logical AND=→"Burninind":bool)
        }
        frame "Visual Inspec" {
          w1710 = T13."Enabled" ("Disabled")
          w1713 = T13."Disabled and Grayed Out" ("Disabled")
          n835 = property on="Start" class="Bool (strict)"(error in=w1712, "DisabledEnum"=w1713) -> (error out=w1714:errorcluster)  [unwired: 1 in, 1 out]
          n836 = property on="Report" class="Bool (strict)"(error in=w1714, "DisabledEnum"=w1713) -> (error out=w1711:errorcluster)  [unwired: 1 in, 1 out]
          n837 = call "VisualInspection.vi"("error in (no error)"=w1711, "TableRef"=w1716) -> ("error out"=w1708:errorcluster, "VisualInspectionResult"=w1715:bool)  [unwired: 8 in]
          "VisualInspectionResult" <- w1715
          n838 = property on="Automation" class="Bool (strict)"() -> ("Value"=w1707:bool)  [unwired: 2 in, 2 out]
          n839 = case shown="True" w1707 {
            tunnel: w1715 -> [_ w1717]
            frame False {
            }
            frame True {
              n840 = property on="SetSN" class="Bool (strict)"("Val(Sgnl)"=w1717) -> ()  [unwired: 2 in, 2 out]
            }
          }
          n841 = property on="Start" class="Bool (strict)"(error in=w1708, "DisabledEnum"=w1710) -> (error out=w1709:errorcluster)  [unwired: 1 in, 1 out]
          n842 = property on="Report" class="Bool (strict)"(error in=w1709, "DisabledEnum"=w1710) -> ()  [unwired: 1 in, 2 out]
        }
        frame "Temp Sens Cal" {
          w1749 = T13."Enabled" ("Disabled")
          w1753 = T13."Disabled and Grayed Out" ("Disabled")
          w1728 = "7.5.5.Temperature sensor calibration test in process..." ("Value")
          w1733 = FALSE ("Clear Log")
          w1720 = "7.5.5" ("Test Paragraph")
          # "K15 OFF + Venable"
          # "K15 OFF + Venable"
          n843 = property on="Start" class="Bool (strict)"(error in=w1752, "DisabledEnum"=w1753) -> (error out=w1754:errorcluster)  [unwired: 1 in, 1 out]
          n844 = property on="Report" class="Bool (strict)"(error in=w1754, "DisabledEnum"=w1753) -> (error out=w1751:errorcluster)  [unwired: 1 in, 1 out]
          n845 = VISA Flush I/O Buffer(VISA resource name=w1757, error in (no error)=w1751) -> (VISA resource name out=w1736:refnum<visa-resource-name>, error out=w1756:errorcluster)  [unwired: 1 in]
          n846 = control-ref of="VISA resource name out"() -> (w1744:refnum<vi>)
          n847 = control-ref of="Config_CANAT"() -> (w1723:refnum<vi>)
          n848 = control-ref of="UUT"() -> (w1724:refnum<vi>)
          n849 = control-ref of="Pannel User Message"() -> (w1759:refnum<vi>)
          n850 = Byte Array To String(unsigned byte array=u8[] [75, 0, 4, 2, 0, 0, 0, 0] ("appended array")) -> (string=w1738:string)
          n851 = Concatenate Strings("EP=1\r\nAO" ("string"), "[", "1" ("string"), "]=0", "\r\n" ("write buffer")) -> (w1763:string)
          n852 = Byte Array To String(unsigned byte array=u8[] [75, 0, 4, 2, 0, 0, 16, 0] ("appended array")) -> (string=w1745:string)
          n853 = property class="Str"(reference=w1759, error in=w1756, "Value"=w1728) -> (error out=w1758:errorcluster)  [unwired: 1 out]
          n854 = call "Reset old test Values (SubVI).vi"("error in"=w1758, "Atr in"=w1719, "Test Paragraph"=w1720) -> ("error out"=w1721:errorcluster)  [unwired: 8 in]
          n855 = call "Table_ScrollaBarMarvin.vi"("error in"=w1721, "Line to focus"=w1720, "reference in"=w1719) -> ("error out"=w1770:errorcluster)  [unwired: 2 out]
          n856 = property class="Tbl (strict)"(reference=w1719, error in=w1770) -> (error out=w1772:errorcluster, "Value"=w1773:string[][])  [unwired: 1 out]
          n857 = Index Array(array=w1773, index (col)=0 ("disabled index (col)")) -> (element=w1774:string[])  [unwired: 1 in]
          n858 = call "Find_Number_LineMARVIN.vi"("Test Paragraph"=w1720, "error in"=w1772, "Row Headers[]"=w1774) -> ("error out"=w1769:errorcluster, "Line number"=w1767:i32)  [unwired: 2 in, 2 out]
          n859 = property on="Serial" class="Bool (strict)"(error in=w1769) -> (error out=w1762:errorcluster, "Value"=w1768:bool)  [unwired: 1 in, 1 out]
          n860 = call "CANSendMotorSpeed.vi"("Remote"=TRUE, "error in (no error)"=w1762, "Motor Speed RPM"=u16 0, "UUT"=w1724, "Cluster in"=w1723) -> ("error out"=w1727:errorcluster)  [unwired: 6 in]
          n861 = call "Time Delay13"("error in (no error)"=w1727) -> ("error out"=w1722:errorcluster)  [unwired: 10 in]
          n862 = call "SerialMarvinMod.vi"("error in (no error)"=w1722, "Clear Log"=w1733, "write buffer"=w1763, "VISA resource name"=w1736) -> ("error out"=w1742:errorcluster)  [unwired: 6 in, 1 out]
          n863 = property class="VISAName"(reference=w1744, error in=w1742) -> (error out=w1746:errorcluster, "Value"=w1747:refnum<visa-resource-name>)  [unwired: 1 out]
          n864 = VISA Write(VISA resource name=w1747, write buffer=w1745, error in (no error)=w1746) -> (VISA resource name out=w1737:refnum<visa-resource-name>, error out=w1740:errorcluster)  [unwired: 1 out]
          n865 = call "Time Delay6"("error in (no error)"=w1740) -> ("error out"=w1739:errorcluster)  [unwired: 10 in]
          n866 = VISA Write(VISA resource name=w1737, write buffer=w1738, error in (no error)=w1739) -> (error out=w1734:errorcluster)  [unwired: 2 out]
          n867 = call "SerialMarvinMod.vi"("error in (no error)"=w1734, "Clear Log"=w1733, "write buffer"="AO[1]\r\n", "VISA resource name"=w1736) -> ("error out"=w1718:errorcluster, "read buffer"=w1732:string)  [unwired: 6 in]
          n868 = Equal?(x=w1732, y="") -> (x = y?=w1729:bool)
          n869 = And(x=w1768, y=w1729) -> (x .and. y?=w1730:bool)
          n870 = case shown="True" w1730 {
            selector: w1730 -> [w1776 _]
            tunnel: w1718 -> [w1781 _]
            tunnel: w1719 -> [w1780 w1817]
            tunnel: w1767 -> [w1779 w1816]
            tunnel: w1736 -> [_ w1820]
            tunnel: [w1776 w1808] -> w1755
            tunnel: [w1775 w1787] -> w1748
            tunnel: w1728 -> [_ w1805]
            tunnel: w1718 -> [_ w1804]
            frame False {
              n871 = Increment(x=w1779) -> (x+1=w1778:i32)
              n872 = call "PassOrFail (SubVI).vi"("disabled index (col)"=6, "index (row)"=w1778, "error in (no error)"=w1775, "Boolean"=w1776, "Table in"=w1780) -> ()  [unwired: 6 in, 1 out]
              n873 = flat-sequence {
                tunnel: w1781 -> [w1782]
                tunnel: [w1782] -> w1775
                frame #0 {
                  n874 = One Button Dialog(message="Please establish RS connection.") -> ()  [unwired: 1 in, 1 out]
                }
              }
            }
            frame True {
              (unwired) dbl[] [0.68545] ("Val 2")
              (unwired) dbl[] [0.69103] ("Val 2")
              (unwired) u32[] [2048]
              # "Max"
              n875 = control-ref of="Stop Button"() -> (w1799:refnum<vi>)
              n876 = control-ref of="Motor Speed RPM"() -> (w1797:refnum<vi>)
              n877 = control-ref of="Pannel User Message"() -> (w1798:refnum<vi>)
              n878 = To Unsigned Long Integer(number=u32 0) -> (unsigned 32bit integer=w1837:u32)
              n879 = Split Number(x=w1837) -> (hi(x)=w1843:u16, lo(x)=w1844:u16)
              n880 = Split Number(x=w1844) -> (hi(x)=w1842:u8, lo(x)=w1841:u8)
              n881 = Increment(x=w1816) -> (x+1=w1828:i32)
              n882 = Split Number(x=w1843) -> (hi(x)=w1840:u8, lo(x)=w1839:u8)
              n883 = Build Array(u8 75, u8 0 ("element"), u8 4 ("Length"), u8 2, w1841, w1842, w1839, w1840) -> (w1835:u8[])
              n884 = Byte Array To String(unsigned byte array=w1835) -> (string=w1848:string)
              n885 = Byte Array To String(unsigned byte array=u8[] [75, 0, 4, 2, 0, 0, 16, 0] ("appended array")) -> (string=w1803:string)
              n886 = for {
                tunnel: u32[] [64, 512, 2048, 8192] -> [w1893] mode=indexing
                tunnel: w1820 -> [w1922]
                tunnel: dbl[] [0.59774, 0.65238, 0.68545, 0.71584] ("Val 2") -> [w1882] mode=indexing
                tunnel: [w1879] -> w1855 mode=indexing
                tunnel: [w1921] -> w1849
                tunnel: [w1897] -> w1800
                tunnel: [w1879] -> w1814 mode=indexing
                tunnel: [w1920] -> w1811 mode=indexing
                tunnel: dbl[] [0.60155, 0.65733, 0.69103, 0.72203] ("Val 2") -> [w1918] mode=indexing
                tunnel: [w1919] -> w1807 mode=indexing
                tunnel: [w1916] -> w1806 mode=indexing
                tunnel: w1805 -> [w1915]
                tunnel: w1804 -> [w1888]
                n887 = control-ref of="VISA resource name out"() -> (w1907:refnum<vi>)
                n888 = control-ref of="Stop Button"() -> (w1913:refnum<vi>)
                n889 = control-ref of="Motor Speed RPM"() -> (w1914:refnum<vi>)
                n890 = control-ref of="Pannel User Message"() -> (w1912:refnum<vi>)
                n891 = To Unsigned Long Integer(number=w1893) -> (unsigned 32bit integer=w1904:u32)
                n892 = Split Number(x=w1904) -> (hi(x)=w1899:u16, lo(x)=w1898:u16)
                n893 = Split Number(x=w1898) -> (hi(x)=w1900:u8, lo(x)=w1901:u8)
                n894 = Split Number(x=w1899) -> (hi(x)=w1902:u8, lo(x)=w1903:u8)
                n895 = Build Array(u8 75, u8 0 ("element"), u8 4 ("Length"), u8 2, w1901, w1900, w1903, w1902) -> (w1905:u8[])
                n896 = Byte Array To String(unsigned byte array=w1905) -> (string=w1906:string)
                n897 = call "Write panel message (SubVI).vi"("rpm"=w1914, "PrintTime"=FALSE, "Stop"=w1913, "error in (no error)"=w1888, "Time to wait"=0.1, "Strin"="7.5.5.Temperature sensor calibration test in process...", "String in"=w1912) -> ("error out"=w1911:errorcluster)  [unwired: 4 in]
                n898 = property class="VISAName"(reference=w1907, error in=w1911) -> (error out=w1908:errorcluster, "Value"=w1897:refnum<visa-resource-name>)  [unwired: 1 out]
                n899 = VISA Flush I/O Buffer(VISA resource name=w1897, error in (no error)=w1908) -> (VISA resource name out=w1910:refnum<visa-resource-name>, error out=w1909:errorcluster)  [unwired: 1 in]
                n900 = VISA Write(VISA resource name=w1910, write buffer=w1906, error in (no error)=w1909) -> (error out=w1887:errorcluster)  [unwired: 2 out]
                n901 = call "Time Delay3"("error in (no error)"=w1887) -> ("error out"=w1886:errorcluster)  [unwired: 10 in]
                n902 = while {
                  tunnel: w1922 -> [w1956]
                  tunnel: [w1926] -> _
                  tunnel: [w1954] -> w1920
                  tunnel: [w1924] -> w1885
                  tunnel: w1882 -> [w1925]
                  tunnel: [w1941] -> w1919
                  tunnel: w1918 -> [w1942]
                  tunnel: [w1955] -> w1921
                  shift-right: [w1934] -> w1916
                  shift-left: 0.0 -> [w1935]
                  tunnel: w1915 -> [w1932]
                  tunnel: w1886 -> [w1928]
                  tunnel: [w1927] -> w1884 mode=indexing
                  i -> [w1939]
                  stop <- w1940 stop-if-true
                  n903 = control-ref of="Stop Button"() -> (w1930:refnum<vi>)
                  n904 = control-ref of="Motor Speed RPM"() -> (w1929:refnum<vi>)
                  n905 = control-ref of="Pannel User Message"() -> (w1931:refnum<vi>)
                  n906 = Equal?(x=w1939, y=10) -> (x = y?=w1937:bool)
                  n907 = property on="Stop Button" class="Bool (strict)"() -> ("Value"=w1936:bool)  [unwired: 2 in, 2 out]
                  n908 = Compound Arithmetic op=OR(w1936, w1937) -> (w1940:bool)
                  n909 = Concatenate Strings("TA" ("string"), "[", "Index", "]", "\r\n" ("write buffer")) -> (w1948:string)
                  n910 = call "Write panel message (SubVI).vi"("rpm"=w1929, "PrintTime"=FALSE, "Stop"=w1930, "error in (no error)"=w1928, "Time to wait"=0.5 ("Delay Time (sec)"), "Strin"=w1932, "String in"=w1931) -> ("error out"=w1946:errorcluster)  [unwired: 4 in]
                  n911 = call "SerialMarvinMod.vi"("error in (no error)"=w1946, "Clear Log"=FALSE, "write buffer"=w1948, "VISA resource name"=w1956) -> ("error out"=w1955:errorcluster, "read buffer"=w1954:string)  [unwired: 6 in]
                  n912 = Fract/Exp String To Number(string=w1954) -> (number=w1927:dbl)  [unwired: 3 in, 1 out]
                  n913 = Subtract(x=w1927, y=w1925) -> (x-y=w1926:dbl)
                  n914 = Multiply(x=w1925, y=0.015) -> (x*y=w1943:dbl)
                  n915 = Subtract(x=w1925, y=w1943) -> (x-y=w1941:dbl)
                  n916 = In Range and Coerce(upper limit=w1942, x=w1927, lower limit=w1941) -> (In Range?=w1923:bool)  [unwired: 1 out]
                  n917 = case shown="True" w1923 {
                    tunnel: w1927 -> [w1958 w1961]
                    tunnel: [w1957 w1960] -> w1924
                    tunnel: w1935 -> [w1959 w1962]
                    tunnel: [w1957 w1960] -> w1934
                    frame False {
                      n918 = Max & Min(x=w1959, y=w1958) -> (max(x,y)=w1957:dbl)  [unwired: 1 out]
                    }
                    frame True {
                      n919 = Max & Min(x=w1962, y=w1961) -> (max(x,y)=w1960:dbl)  [unwired: 1 out]
                    }
                  }
                }
                n920 = Add Array Elements(numeric array=w1884) -> (sum=w1883:dbl)
                n921 = Divide(x=w1883, y=11.0 ("x")) -> (x/y=w1881:dbl)
                n922 = Subtract(x=w1885, y=w1882) -> ()  [unwired: 1 out]
                n923 = Subtract(x=w1881, y=w1882) -> (x-y=w1879:dbl)
              }
              "Array 2" <- w1814
              "Array 3" <- w1811
              "Array 4" <- w1807
              "Array 5" <- w1806
              n924 = Add Array Elements(numeric array=w1855) -> (sum=w1854:dbl)
              n925 = Divide(x=w1854, y=4.0) -> (x/y=w1813:dbl)
              n926 = In Range and Coerce(upper limit=0.1, x=w1813, lower limit=-0.1) -> (In Range?=w1809:bool)  [unwired: 1 out]
              n927 = And(x=w1809, y=w1809) -> (x .and. y?=w1808:bool)
              n928 = Number To Fractional String(number=w1813, precision (6)=i16 7) -> (F-format string=w1812:string)  [unwired: 2 in]
              n929 = Concatenate Strings("EP=1\r\nAO" ("string"), "[", "1" ("string"), "]=", w1812, "\r\n" ("write buffer")) -> (w1823:string)
              n930 = call "PassOrFail (SubVI).vi"("disabled index (col)"=6, "index (row)"=w1828, "error in (no error)"=w1849, "Boolean"=w1809, "Table in"=w1817) -> ("error out"=w1830:errorcluster)  [unwired: 6 in]
              n931 = property class="Tbl (strict)"(reference=w1817, error in=w1830) -> (reference out=w1834:refnum<vi>, error out=w1833:errorcluster, "Value"=w1831:string[][])
              n932 = Number To Fractional String(number=w1813, precision (6)=i16 4) -> (F-format string=w1818:string)  [unwired: 2 in]
              n933 = Replace Array Subset(array=w1831, new element=w1818, index (row)=w1828, index (col)=5 ("disabled index (col)")) -> (w1832:string[][])
              n934 = property class="Tbl (strict)"(reference=w1834, error in=w1833, "Value"=w1832) -> (error out=w1790:errorcluster)  [unwired: 1 out]
              n935 = case shown="True" w1809 {
                tunnel: w1823 -> [_ w1867]
                tunnel: w1790 -> [w1857 w1866]
                tunnel: w1820 -> [w1856 w1861]
                tunnel: ["0" ("read buffer") w1859] -> w1819
                tunnel: [w1857 w1863] -> w1789
                frame False {
                  n936 = VISA Flush I/O Buffer(VISA resource name=w1856, error in (no error)=w1857) -> ()  [unwired: 1 in, 2 out]
                }
                frame True {
                  n937 = call "SerialMarvinMod.vi"("error in (no error)"=w1866, "Clear Log"=FALSE, "write buffer"=w1867, "VISA resource name"=w1861) -> ("error out"=w1865:errorcluster)  [unwired: 6 in, 1 out]
                  n938 = disable-structure shown="Enabled" {
                    disable-tunnel: w1865 -> [w1875 w1878]
                    disable-tunnel: [w1872 w1876] -> w1863
                    disable-tunnel: "AO[1]\r\n" ("write buffer") -> [w1871 _]
                    disable-tunnel: w1861 -> [w1870 w1877]
                    disable-tunnel: FALSE ("Clear Log") -> [w1869 _]
                    disable-tunnel: [w1868 _] -> w1859
                    frame Disabled {
                      n939 = call "Time Delay4"("error in (no error)"=w1875) -> ("error out"=w1874:errorcluster)  [unwired: 10 in]
                      n940 = call "SerialMarvinMod.vi"("error in (no error)"=w1874, "Clear Log"=w1869, "write buffer"=w1871, "VISA resource name"=w1870) -> ("error out"=w1873:errorcluster)  [unwired: 6 in, 1 out]
                      n941 = call "SerialMarvinMod.vi"("error in (no error)"=w1873, "Clear Log"=w1869, "write buffer"=w1871, "VISA resource name"=w1870) -> ("error out"=w1872:errorcluster, "read buffer"=w1868:string)  [unwired: 6 in]
                    }
                    frame Enabled {
                      n942 = VISA Flush I/O Buffer(VISA resource name=w1877, error in (no error)=w1878) -> (error out=w1876:errorcluster)  [unwired: 1 in, 1 out]
                    }
                  }
                }
              }
              n943 = Equal?(x=w1812, y=w1819) -> ()  [unwired: 1 out]
              n944 = VISA Write(VISA resource name=w1800, write buffer=w1803, error in (no error)=w1789) -> (error out=w1801:errorcluster)  [unwired: 2 out]
              n945 = call <vilib>:"Clear Errors.vi"("error in (no error)"=w1801) -> ("error out"=w1794:errorcluster)  [unwired: 5 in, 1 out]
              n946 = call "Write panel message (SubVI).vi"(4:"rpm"=w1797, 5:"rpm"=FALSE ("rpm"), "PrintTime"=TRUE, "Stop"=w1799, "error in (no error)"=w1794, "Time to wait"=15.0, "Strin"="7.5.5.Temperature sensor calibration test in process...", "String in"=w1798) -> ("error out"=w1791:errorcluster)  [unwired: 3 in]
              n947 = VISA Write(VISA resource name=w1800, write buffer=w1848, error in (no error)=w1791) -> (error out=w1788:errorcluster)  [unwired: 2 out]
              n948 = call <vilib>:"Clear Errors.vi"("error in (no error)"=w1788) -> ("error out"=w1787:errorcluster)  [unwired: 5 in, 1 out]
              n949 = call "PassOrFail (SubVI).vi"("disabled index (col)"=6, "index (row)"=w1816, "error in (no error)"=w1787, "Boolean"=w1809, "Table in"=w1817) -> ()  [unwired: 6 in, 1 out]
            }
          }
          "TempSensCalind" <- w1755
          n950 = property on="Start" class="Bool (strict)"(error in=w1748, "DisabledEnum"=w1749) -> (error out=w1750:errorcluster)  [unwired: 1 in, 1 out]
          n951 = property on="Report" class="Bool (strict)"(error in=w1750, "DisabledEnum"=w1749) -> ()  [unwired: 1 in, 2 out]
        }
        frame "Auxiliary" {
          w1970 = T13."Enabled" ("Disabled")
          w1974 = T13."Disabled and Grayed Out" ("Disabled")
          w1967 = "8.Auxiliary test" ("Value")
          w1965 = "8" ("Test Paragraph")
          # "K20 OFF"
          # "K20 ON"
          # "OFF"
          n952 = property on="Start" class="Bool (strict)"(error in=w1973, "DisabledEnum"=w1974) -> (error out=w1975:errorcluster)  [unwired: 1 in, 1 out]
          n953 = property on="Report" class="Bool (strict)"(error in=w1975, "DisabledEnum"=w1974) -> (error out=w1972:errorcluster)  [unwired: 1 in, 1 out]
          n954 = control-ref of="Pannel User Message"() -> (w1989:refnum<vi>)
          n955 = control-ref of="VISA resource name out"() -> (w1992:refnum<vi>)
          n956 = property class="Str"(reference=w1989, error in=w1972, "Value"=w1967) -> (reference out=w1968:refnum<vi>, error out=w1988:errorcluster)
          n957 = Build Array(u8[] [75, 0, 4, 2, 0, 0, 8, 0] ("appended array"), u8[] [75, 0, 4, 2, 0, 0, 0, 0] ("appended array")) -> (w1984:u8[][])
          n958 = Byte Array To String(unsigned byte array=u8[] [75, 0, 4, 2, 0, 0, 0, 0] ("appended array")) -> (string=w1994:string)
          n959 = call "Reset old test Values (SubVI).vi"("error in"=w1988, "Atr in"=w1964, "Test Paragraph"=w1965) -> ("error out"=w1966:errorcluster)  [unwired: 8 in]
          n960 = call "Table_ScrollaBarMarvin.vi"("error in"=w1966, "Line to focus"=w1965, "reference in"=w1964) -> ("error out"=w2002:errorcluster)  [unwired: 2 out]
          n961 = property class="Tbl (strict)"(reference=w1964, error in=w2002) -> (reference out=w1983:refnum<vi>, error out=w2001:errorcluster, "Value"=w2000:string[][])
          n962 = Index Array(array=w2000, index (col)=0 ("disabled index (col)")) -> (element=w1999:string[])  [unwired: 1 in]
          n963 = call "Find_Number_LineMARVIN.vi"("Test Paragraph"=w1965, "error in"=w2001, "Row Headers[]"=w1999) -> ("error out"=w1997:errorcluster, "Line number"=w1987:i32)  [unwired: 2 in, 2 out]
          n964 = call "Table_ScrollaBarMarvin.vi"("error in"=w1997, "Line to focus"=w1965, "reference in"=w1983) -> ("error out"=w1996:errorcluster)  [unwired: 2 out]
          n965 = property class="VISAName"(reference=w1992, error in=w1996) -> (error out=w1980:errorcluster, "Value"=w2003:refnum<visa-resource-name>)  [unwired: 1 out]
          n966 = call "Wait_Sec.vi"("Delay Time (sec)"=2.0, "error out"=w1980) -> ("error in"=w1991:errorcluster)  [unwired: 2 in]
          n967 = call <vilib>:"Clear Errors.vi"("error in (no error)"=w1991) -> ("error out"=w1963:errorcluster)  [unwired: 5 in, 1 out]
          n968 = for {
            tunnel: w2003 -> [w2060]
            tunnel: w1963 -> [w2058]
            tunnel: w1984 -> [w2054] mode=indexing
            tunnel: w1983 -> [w2040]
            tunnel: w1987 -> [w2043]
            tunnel: [w2041] -> w1982
            tunnel: dbl[] [0.3, 1.7] -> [w2026] mode=indexing
            tunnel: [w2009] -> w1979 mode=indexing
            tunnel: [w2008] -> w1978 mode=indexing
            tunnel: w1968 -> [w2019]
            tunnel: w1967 -> [w2017]
            i -> [w2024]
            stop <- w2011 stop-if-true
            w2047 = 6 ("disabled index (col)")
            n969 = control-ref of="Stop Button"() -> (w2018:refnum<vi>)
            n970 = control-ref of="Motor Speed RPM"() -> (w2014:refnum<vi>)
            n971 = property on="Stop Button" class="Bool (strict)"() -> ("Value"=w2012:bool)  [unwired: 2 in, 2 out]
            n972 = Equal To 0?(x=w2024) -> (x = 0?=w2023:bool)
            n973 = Select(t="Please turn-on heat gun." ("Message"), s=w2023, f="Please turn-off heat gun." ("Message")) -> ()  [unwired: 1 out]
            n974 = Byte Array To String(unsigned byte array=w2054) -> (string=w2059:string)
            n975 = VISA Write(VISA resource name=w2060, write buffer=w2059, error in (no error)=w2058) -> (VISA resource name out=w2055:refnum<visa-resource-name>, error out=w2057:errorcluster)  [unwired: 1 out]
            n976 = call "Write panel message (SubVI).vi"("rpm"=w2014, "PrintTime"=FALSE, "Stop"=w2018, "error in (no error)"=w2057, "Time to wait"=10.0 ("Delay Time (sec)"), "Strin"=w2017, "String in"=w2019) -> ("error out"=w2020:errorcluster)  [unwired: 4 in]
            n977 = Multiply(x=w2024, y=2) -> (x*y=w2036:i32)
            n978 = Increment(x=w2036) -> (x+1=w2037:i32)
            n979 = Add(x=w2043, y=w2037) -> (x+y=w2038:i32)
            n980 = Increment(x=w2038) -> (x+1=w2048:i32)
            n981 = flat-sequence {
              tunnel: w2020 -> [w2288]
              tunnel: [w2288] -> w2053
              tunnel: [w2287] -> w2004
              frame #0 {
                n982 = call <vilib>:"High Resolution Relative Seconds.vi"() -> ("relative seconds"=w2287:dbl)
              }
            }
            n983 = while {
              tunnel: w2004 -> [w2129]
              tunnel: w2055 -> [w2128]
              tunnel: w2053 -> [w2117]
              tunnel: [w2085] -> w2039
              tunnel: [w2076] -> w2042
              tunnel: w2024 -> [w2116]
              tunnel: [w2115] -> w2009
              tunnel: [w2095] -> w2008
              tunnel: w2026 -> [w2114]
              tunnel: w2024 -> [w2074]
              tunnel: w2019 -> [w2107]
              tunnel: w2018 -> [w2106]
              tunnel: w2017 -> [w2103]
              shift-right: [w2093] -> _
              shift-left: 0.0 ("Value") -> [w2092]
              tunnel: w2014 -> [w2089]
              shift-right: [w2082] -> _
              shift-left: 0.0 ("Value") -> [w2083]
              shift-right: [w2075] -> _
              shift-left: 0.0 ("Value") -> [w2077]
              shift-right: [w2080] -> _
              shift-left: 0.0 ("Value") -> [w2079]
              tunnel: [w2081] -> w2006
              tunnel: w2004 -> [w2078]
              stop <- w2111 stop-if-true
              w2096 = 500.0 ("y")
              # "Get Ebay fan by ADC (3)"
              n984 = control-ref of="Power transistor Heat sink Temp."() -> (w2118:refnum<vi>)
              n985 = call <vilib>:"High Resolution Relative Seconds.vi"() -> ("relative seconds"=w2119:dbl)
              n986 = Byte Array To String(unsigned byte array=u8[] [75, 0, 4, 18, 0, 0, 0, 0] ("appended array")) -> (string=w2127:string)
              n987 = VISA Write(VISA resource name=w2128, write buffer=w2127, error in (no error)=w2117) -> (VISA resource name out=w2112:refnum<visa-resource-name>, error out=w2113:errorcluster)  [unwired: 1 out]
              n988 = property on="Stop Button" class="Bool (strict)"() -> ("Value"=w2109:bool)  [unwired: 2 in, 2 out]
              n989 = Subtract(x=w2119, y=w2129) -> (x-y=w2091:dbl)
              n990 = Subtract(x=w2096, y=w2091) -> (x-y=w2101:dbl)
              n991 = Number To Fractional String(number=w2101, precision (6)=i16 2) -> (F-format string=w2100:string)  [unwired: 2 in]
              n992 = Greater Or Equal?(x=w2091, y=w2096) -> (x >= y?=w2110:bool)
              n993 = VISA Read(VISA resource name=w2112, byte count=u32 1, error in (no error)=w2113) -> (VISA resource name out=w2121:refnum<visa-resource-name>, read buffer=w2122:string, error out=w2120:errorcluster)  [unwired: 1 out]
              n994 = String To Byte Array(string=w2122) -> (unsigned byte array=w2125:u8[])
              n995 = Index Array(array=w2125, index=0) -> (element=w2123:u8)
              n996 = case shown="75" w2123 {
                tunnel: [w2230 w2236] -> w2084
                tunnel: w2121 -> [_ w2244]
                tunnel: w2120 -> [w2230 w2243]
                tunnel: [FALSE w2234] -> w2095
                tunnel: [u32 9999 w2233] -> _
                tunnel: w2114 -> [_ w2232]
                tunnel: w2074 -> [_ w2231]
                frame 0, Default {
                }
                frame 75 {
                  n997 = VISA Read(VISA resource name=w2244, byte count=u32 3, error in (no error)=w2243) -> (VISA resource name out=w2239:refnum<visa-resource-name>, read buffer=w2247:string, error out=w2238:errorcluster)  [unwired: 1 out]
                  n998 = String To Byte Array(string=w2247) -> (unsigned byte array=w2237:u8[])
                  n999 = Index Array(array=w2237, index #1=0 ("index")) -> (element #1=w2242:u8, element #2=w2240:u8)  [unwired: 2 in, 1 out]
                  n1000 = Equal?(x=u8 0, y=w2242) -> (x = y?=w2241:bool)
                  n1001 = case shown="True" w2241 {
                    tunnel: [w2250 w2258] -> w2236
                    tunnel: w2240 -> [_ w2264]
                    tunnel: w2239 -> [_ w2263]
                    tunnel: w2238 -> [w2250 w2262]
                    tunnel: w2237 -> [_ w2261]
                    tunnel: [FALSE w2253] -> w2234
                    tunnel: [u32 9999 w2254] -> w2233
                    tunnel: w2232 -> [_ w2252]
                    tunnel: w2231 -> [_ w2251]
                    frame False {
                    }
                    frame True {
                      n1002 = VISA Read(VISA resource name=w2263, byte count=w2264, error in (no error)=w2262) -> (read buffer=w2259:string, error out=w2258:errorcluster)  [unwired: 2 out]
                      n1003 = String To Byte Array(string=w2259) -> (unsigned byte array=w2260:u8[])
                      n1004 = Insert Into Array(array=w2261, new element=w2260) -> (w2255:u8[])  [unwired: 1 in]
                      n1005 = Index Array(array=w2255, index #1=0 ("index")) -> (element #3=w2256:u8)  [unwired: 2 in, 2 out]
                      n1006 = case shown="15..19" w2256 {
                        tunnel: w2255 -> [_ w2279]
                        tunnel: [u32 9999 w2270] -> w2254
                        tunnel: [FALSE w2269] -> w2253
                        tunnel: w2252 -> [_ w2268]
                        tunnel: w2251 -> [_ w2267]
                        frame 0, Default {
                        }
                        frame 15..19 {
                          n1007 = Index Array(array=w2279, index #1=3 ("index")) -> (element #1=w2278:u8, element #2=w2277:u8, element #3=w2276:u8, element #4=w2275:u8)  [unwired: 3 in]
                          n1008 = Join Numbers(hi=w2275, lo=w2276) -> ((hi.lo)=w2273:u16)
                          n1009 = Join Numbers(hi=w2277, lo=w2278) -> ((hi.lo)=w2274:u16)
                          n1010 = Join Numbers(hi=w2273, lo=w2274) -> ((hi.lo)=w2271:u32)
                          n1011 = Multiply(x=0.0008056640625, y=w2271) -> (x*y=w2270:dbl)
                          n1012 = case shown="0, Default" w2267 {
                            tunnel: w2270 -> [w2283 w2285]
                            tunnel: [w2282 w2284] -> w2269
                            tunnel: w2268 -> [w2281 w2286]
                            frame 0, Default {
                              n1013 = Less Or Equal?(x=w2283, y=w2281) -> (x <= y?=w2282:bool)
                            }
                            frame 1 {
                              n1014 = Greater Or Equal?(x=w2285, y=w2286) -> (x >= y?=w2284:bool)
                            }
                          }
                        }
                      }
                    }
                  }
                }
              }
              n1015 = property class="DigNum (strict)"(reference=w2118, error in=w2084) -> (error out=w2086:errorcluster, "Value"=w2076:dbl)  [unwired: 1 out]
              n1016 = Number To Fractional String(number=w2076, precision (6)=i16 2) -> (F-format string=w2097:string)  [unwired: 2 in]
              n1017 = Concatenate Strings(w2103, "\nTimeout [sec]: " ("string"), w2100, "\nTemperature [Deg.]: " ("string"), w2097) -> (w2105:string)
              n1018 = call "Write panel message (SubVI).vi"(4:"rpm"=w2089, 5:"rpm"=FALSE ("rpm"), "PrintTime"=FALSE, "Stop"=w2106, "Time to wait"=0.2, "Strin"=w2105, "String in"=w2107) -> ()  [unwired: 4 in, 1 out]
              n1019 = case shown="0, Default" w2116 {
                tunnel: [w2199 w2224] -> w2115
                tunnel: w2076 -> [w2206 w2226]
                tunnel: w2095 -> [w2210 w2223]
                tunnel: [w2196 w2222] -> w2094
                tunnel: [w2206 0.0 ("Value")] -> w2093
                tunnel: w2092 -> [w2207 _]
                tunnel: w2091 -> [w2203 _]
                tunnel: [w2201 FALSE] -> w2090
                tunnel: w2086 -> [w2200 w2219]
                tunnel: [w2200 w2219] -> w2085
                tunnel: w2083 -> [w2198 w2218]
                tunnel: [w2197 w2218] -> w2082
                frame 0, Default {
                  n1020 = In Range and Coerce(upper limit=63.0, x=w2206, lower limit=58.0 ("y")) -> (In Range?=w2199:bool)  [unwired: 1 out]
                  n1021 = Less Or Equal?(x=w2206, y=w2207) -> (x <= y?=w2205:bool)
                  n1022 = Greater?(x=w2203, y=200.0) -> (0:w2204:bool)
                  n1023 = And(x=w2205, y=w2204) -> (x .and. y?=w2201:bool)
                  n1024 = Compound Arithmetic op=AND(w2199, w2210) -> (w2209:bool)
                  n1025 = case shown="True" w2199 {
                    tunnel: w2198 -> [_ w2217]
                    tunnel: [0.0 ("Value") w2216] -> w2197
                    tunnel: [FALSE w2214] -> w2195
                    frame False {
                    }
                    frame True {
                      n1026 = Increment(x=w2217) -> (x+1=w2216:dbl)
                      n1027 = Greater?(x=w2216, y=15.0) -> (0:w2214:bool)
                    }
                  }
                  n1028 = Or(x=w2195, y=w2209) -> (x .or. y?=w2196:bool)
                }
                frame 1 {
                  n1029 = In Range and Coerce(upper limit=57.0, x=w2226, lower limit=53.0 ("y")) -> (In Range?=w2224:bool)  [unwired: 1 out]
                  n1030 = Compound Arithmetic op=AND(w2224, w2223) -> (w2222:bool)
                }
              }
              n1031 = case shown="0, Default" w2074 {
                tunnel: [w2137 FALSE] -> w2081
                tunnel: [w2136 w2192] -> w2080
                tunnel: w2079 -> [w2135 w2192]
                tunnel: w2078 -> [w2134 _]
                tunnel: w2077 -> [w2133 w2194]
                tunnel: w2076 -> [w2132 _]
                tunnel: [w2131 w2194] -> w2075
                frame 0, Default {
                  n1032 = disable-structure shown="Enabled" {
                    disable-tunnel: w2133 -> [w2142 w2171]
                    disable-tunnel: w2132 -> [w2141 w2179]
                    disable-tunnel: [w2140 w2178] -> w2137
                    disable-tunnel: [w2139 w2177] -> w2136
                    disable-tunnel: w2135 -> [w2138 w2175]
                    disable-tunnel: w2134 -> [_ _]
                    disable-tunnel: w2132 -> [_ w2173]
                    disable-tunnel: [_ w2172] -> w2131
                    frame Disabled {
                      n1033 = case shown="0, Default" {
                        selector: _ -> [_ _]
                        tunnel: w2142 -> [w2147 w2161]
                        tunnel: w2141 -> [w2146 w2160]
                        tunnel: w2138 -> [w2150 w2162]
                        tunnel: [w2149 w2163] -> w2140
                        tunnel: [w2148 w2164] -> w2139
                        frame 0, Default {
                          n1034 = Subtract(x=w2146, y=w2147) -> (x-y=w2143:dbl)
                          n1035 = Greater?(x=w2143, y=1.0) -> (0:w2144:bool)
                          n1036 = case shown="False" w2144 {
                            tunnel: w2150 -> [w2154 _]
                            tunnel: [w2153 0.0 ("upper limit")] -> w2148
                            tunnel: [w2151 FALSE] -> w2149
                            frame False {
                              n1037 = Increment(x=w2154) -> (x+1=w2153:dbl)
                              n1038 = Greater Or Equal?(x=w2153, y=60.0) -> (x >= y?=w2151:bool)
                            }
                            frame True {
                            }
                          }
                        }
                        frame 1 {
                          n1039 = Subtract(x=w2161, y=w2160) -> (x-y=w2159:dbl)
                          n1040 = Greater?(x=w2159, y=1.0) -> (0:w2157:bool)
                          n1041 = case shown="False" w2157 {
                            tunnel: w2162 -> [w2168 _]
                            tunnel: [w2167 0.0 ("upper limit")] -> w2164
                            tunnel: [w2165 FALSE] -> w2163
                            frame False {
                              n1042 = Increment(x=w2168) -> (x+1=w2167:dbl)
                              n1043 = Greater Or Equal?(x=w2167, y=60.0) -> (x >= y?=w2165:bool)
                            }
                            frame True {
                            }
                          }
                        }
                      }
                    }
                    frame Enabled {
                      n1044 = Greater Or Equal?(x=w2175, y=200.0) -> (x >= y?=w2174:bool)
                      n1045 = case shown="False" w2174 {
                        tunnel: w2179 -> [_ w2191]
                        tunnel: w2171 -> [_ w2190]
                        tunnel: [FALSE w2186] -> w2178
                        frame False {
                        }
                        frame True {
                          n1046 = Subtract(x=w2191, y=w2190) -> (x-y=w2189:dbl)
                          n1047 = Greater Or Equal?(x=w2189, y=1.0) -> (x >= y?=w2187:bool)
                          n1048 = Not(x=w2187) -> (.not. x?=w2186:bool)
                        }
                      }
                      n1049 = case shown="False" w2174 {
                        tunnel: [w2182 0.0] -> w2177
                        tunnel: w2175 -> [w2181 _]
                        tunnel: w2173 -> [_ w2183]
                        tunnel: [w2180 w2183] -> w2172
                        tunnel: w2171 -> [w2180 _]
                        frame False {
                          n1050 = Increment(x=w2181) -> (x+1=w2182:dbl)
                        }
                        frame True {
                        }
                      }
                    }
                  }
                }
                frame 1 {
                }
              }
              n1051 = Compound Arithmetic op=OR(w2090, w2094, w2110, w2109, w2081) -> (w2111:bool)
            }
            n1052 = call "PassOrFail (SubVI).vi"("disabled index (col)"=w2047, "index (row)"=w2038, "error in (no error)"=w2039, "Boolean"=w2009, "Table in"=w2040) -> ("error out"=w2050:errorcluster)  [unwired: 6 in]
            n1053 = property class="Tbl (strict)"(reference=w2040, error in=w2050) -> (reference out=w2031:refnum<vi>, error out=w2029:errorcluster, "Value"=w2052:string[][])
            n1054 = Number To Fractional String(number=w2042, precision (6)=i16 2) -> (F-format string=w2051:string)  [unwired: 2 in]
            n1055 = Replace Array Subset(array=w2052, new element=w2051, index (row)=w2038, index (col)=5 ("disabled index (col)")) -> (w2034:string[][])
            n1056 = property class="Tbl (strict)"(reference=w2031, error in=w2029, "Value"=w2034) -> (reference out=w2032:refnum<vi>, error out=w2028:errorcluster)
            n1057 = call "PassOrFail (SubVI).vi"("disabled index (col)"=w2047, "index (row)"=w2048, "error in (no error)"=w2028, "Boolean"=w2008, "Table in"=w2040) -> ("error out"=w2027:errorcluster)  [unwired: 6 in]
            n1058 = property class="Tbl (strict)"(reference=w2032, error in=w2027) -> (error out=w2030:errorcluster, "Value"=w2033:string[][])  [unwired: 1 out]
            n1059 = case shown="0, Default" w2024 {
              tunnel: w2008 -> [w2066 w2071]
              tunnel: [w2065 w2070] -> w2025
              tunnel: [w2064 FALSE] -> w2010
              tunnel: w2009 -> [w2063 _]
              tunnel: w2008 -> [w2062 _]
              frame 0, Default {
                n1060 = Not(x=w2062) -> (.not. x?=w2061:bool)
                n1061 = And(x=w2063, y=w2061) -> (x .and. y?=w2064:bool)
                n1062 = Select(t="ON", s=w2066, f="OFF") -> (s? t:f=w2065:string)
              }
              frame 1 {
                n1063 = Select(t="OFF", s=w2071, f="ON") -> (s? t:f=w2070:string)
              }
            }
            n1064 = Compound Arithmetic op=OR(w2006, w2010, w2012) -> (w2011:bool)
            n1065 = Replace Array Subset(array=w2033, new element=w2025, index (row)=w2048, index (col)=5 ("disabled index (col)")) -> (w2049:string[][])
            n1066 = property class="Tbl (strict)"(reference=w2031, error in=w2030, "Value"=w2049) -> (error out=w2041:errorcluster)  [unwired: 1 out]
          }
          n1067 = property class="VISAName"(reference=w1992, error in=w1982) -> (error out=w1969:errorcluster, "Value"=w1995:refnum<visa-resource-name>)  [unwired: 1 out]
          n1068 = property on="Start" class="Bool (strict)"(error in=w1969, "DisabledEnum"=w1970) -> (error out=w1971:errorcluster)  [unwired: 1 in, 1 out]
          n1069 = property on="Report" class="Bool (strict)"(error in=w1971, "DisabledEnum"=w1970) -> ()  [unwired: 1 in, 2 out]
          n1070 = VISA Write(VISA resource name=w1995, write buffer=w1994, error in (no error)=w1969) -> ()  [unwired: 3 out]
          n1071 = Build Array (concatenate)(w1979, w1978) -> (w1977:bool[])
          n1072 = And Array Elements(Boolean array=w1977) -> (logical AND=→"Auxiind":bool)
        }
      }
      n1073 = property on="Stop Button" class="Bool (strict)"() -> ("Value"=w57:bool)  [unwired: 2 in, 2 out]
      n1074 = Or(x=FALSE, y=w57) -> (x .or. y?=w58:bool)
      "f" <- w61
    }
    n1075 = property on="Pannel User Message" class="Str"(error in=w49, "Value"="You can press \"Start\" button to perform test(s).") -> ()  [unwired: 1 in, 2 out]
  }
  n1076 = call <vilib>:"Application Directory.vi"() -> ("Application Directory"=w16:path)
  n1077 = Build Path(base path=w16, name or relative path="data\\MarvinParams.ini") -> (appended path=w10:path)
  n1078 = call <vilib>:"Open Config Data.vi"("error in (no error)"=w13, "create file if necessary (T)"=FALSE, "configuration file path"=w10) -> ("error out"=w12:errorcluster, "refnum"=w11:T15)  [unwired: 7 out]
  n1079 = disable-structure shown="Disabled" {
    frame Disabled {
      n1080 = property class="Tbl (strict)"() -> (reference=w2303:refnum<vi>, error out=w2302:errorcluster, "Value"=w2295:string[][])  [unwired: 1 in, 1 out]
      n1081 = Replace Array Subset(array=w2295, index (row)=0, index (col)=5 ("disabled index (col)")) -> (w2296:string[][], new element=w2299:string)
      n1082 = Equal?(x="PASS") -> (y=w2300:string, x = y?=w2290:bool)
      n1083 = Select(t=u32 6618880, s=w2290, f=u32 16711680) -> (s? t:f=w2294:u32)
      n1084 = property class="Tbl (strict)"(reference=w2303, error in=w2302, "Active Cell"=T16 {"Row"=0, "Column"=5} ("Active Cell:Active Cell"), "Cell BG Color"=w2294) -> (error out=w2301:errorcluster)  [unwired: 1 out]
      n1085 = property class="Tbl (strict)"(reference=w2303, error in=w2301, "Value"=w2296) -> ()  [unwired: 2 out]
    }
    frame Enabled {
    }
  }
  n1086 = while {
    tunnel: [w2310] -> w9
    tunnel: [w2306] -> w8
    tunnel: [w2307] -> w6
    stop <- w2310 stop-if-true
    n1087 = call "Operator Name"() -> ("Operator Name"=w2306:string, "OK"=w2311:bool)  [unwired: 17 in, 1 out]
    n1088 = Not Equal?(x=w2306, y="") -> (x != y?=w2312:bool)
    n1089 = Equal?(x="nissim", y=w2306) -> (x = y?=w2304:bool)
    n1090 = Equal?(x="admin", y=w2306) -> (x = y?=w2308:bool)
    n1091 = And(x=w2311, y=w2312) -> (x .and. y?=w2310:bool)
    n1092 = Or(x=w2304, y=w2308) -> (x .or. y?=w2307:bool)
  }
  n1093 = while {
    shift-right: [w2334] -> _
    shift-left: w23 -> [w2336]
    shift-right: [w2332] -> _
    shift-left: _ -> [w2333]
    shift-right: [w2329] -> _
    shift-left: _ -> [w2328]
    shift-right: [w2326] -> _
    shift-left: w13 -> [w2326]
    shift-right: [w2325] -> _
    shift-left: w7 -> [w2319]
    shift-right: [w2318] -> _
    shift-left: w7 -> [w2324]
    shift-right: [w2315] -> _
    shift-left: w7 -> [w2323]
    shift-right: [w2317] -> _
    shift-left: w7 -> [w2322]
    shift-right: [w2314] -> _
    shift-left: w7 -> [w2321]
    shift-right: [w2316] -> _
    shift-left: w7 -> [w2320]
    stop <- w2335 stop-if-true
    n1094 = Dequeue Element(queue=w2336, error in (no error)=w2326) -> (queue out=w2334:refnum<queue>, element=w2327:T11, error out=w2335:errorcluster)  [unwired: 1 in, 1 out]
    n1095 = for {
      tunnel: [w2503] -> w2331 mode=indexing
      tunnel: w2327 -> [w2502] mode=indexing
      tunnel: [w2501] -> w2330 mode=indexing
      n1096 = Unbundle By Name(w2502) -> ("aDATA"=w2501:u8[])
      n1097 = call "Array Data to Single Num in Hex.vi"("aDATA"=w2501) -> ("Numeric"=w2503:u64)  [unwired: 10 in]
    }
    n1098 = Build Array (concatenate)(w2331, w2333) -> (w2332:u64[][])
    "Array" <- w2332
    n1099 = for {
      tunnel: w2330 -> [w2353] mode=indexing
      tunnel: [w2351] -> w2329
      tunnel: w2328 -> [w2350]
      tunnel: w2327 -> [w2349]
      shift-right: [w2348] -> w2325
      shift-left: w2319 -> [w2347]
      shift-right: [w2342] -> w2316
      shift-left: w2320 -> [w2341]
      shift-right: [w2346] -> w2318
      shift-left: w2324 -> [w2345]
      shift-right: [w2344] -> w2317
      shift-left: w2322 -> [w2343]
      shift-right: [w2337] -> w2314
      shift-left: w2321 -> [w2338]
      shift-right: [w2340] -> w2315
      shift-left: w2323 -> [w2339]
      i -> [w2352]
      n1100 = case shown="0, Default" w2352 {
        tunnel: w2353 -> [w2414 w2456 w2496]
        tunnel: [w2390 w2451 w2491] -> w2351
        tunnel: w2350 -> [w2391 w2451 w2491]
        tunnel: w2349 -> [w2389 _ _]
        tunnel: [w2375 w2444 w2484] -> w2348
        tunnel: [w2358 w2443 w2483] -> w2346
        tunnel: [w2357 w2441 w2482] -> w2344
        tunnel: w2347 -> [w2378 w2444 w2484]
        tunnel: w2345 -> [w2361 w2443 w2483]
        tunnel: w2343 -> [w2356 w2441 w2482]
        tunnel: [w2374 w2442 w2476] -> w2342
        tunnel: w2341 -> [w2374 w2442 w2477]
        tunnel: [w2371 w2439 w2480] -> w2340
        tunnel: w2339 -> [w2370 w2439 w2480]
        tunnel: w2338 -> [w2367 w2440 w2481]
        tunnel: [w2366 w2440 w2481] -> w2337
        frame 0, Default {
          # "Frame ID\n0x18E1273F"
          n1101 = Index Array(array=w2414, index #1=0 ("index"), index #2=1 ("index"), index #3=2 ("index"), index #4=3 ("index"), index #5=4 ("index"), index #6=5 ("index"), index #7=6 ("index"), index #8=7 ("index")) -> (element #1=w2398:u8, element #2=w2400:u8, element #3=w2401:u8, element #4=w2405:u8, element #5=w2408:u8, element #6=w2412:u8, element #7=w2413:u8, element #8=w2411:u8)
          n1102 = Number To Hexadecimal String(2:w2411) -> (0:w2424:string)  [unwired: 1 in]
          n1103 = Join Numbers(hi=w2413, lo=w2412) -> ((hi.lo)=w2430:u16)
          n1104 = Join Numbers(hi=w2401, lo=w2400) -> ((hi.lo)=w2402:u16)
          n1105 = Number To Hexadecimal String(2:w2408) -> (0:w2409:string)  [unwired: 1 in]
          n1106 = Number To Hexadecimal String(2:w2430) -> (0:w2429:string)  [unwired: 1 in]
          n1107 = Number To Hexadecimal String(2:w2398) -> (0:w2399:string)  [unwired: 1 in]
          n1108 = Number To Hexadecimal String(2:w2402) -> (0:w2403:string)  [unwired: 1 in]
          n1109 = Number To Hexadecimal String(2:w2405) -> (0:w2406:string)  [unwired: 1 in]
          n1110 = Hexadecimal String To Number(string=w2424) -> (number=w2423:u32)  [unwired: 2 in, 1 out]
          n1111 = Index Array(array=w2389, index=0) -> (element=w2387:T17)
          n1112 = To Double Precision Float(number=w2423) -> (double precision float=w2373:dbl)
          n1113 = Unbundle By Name(w2387) -> ("ID"=w2380:u32)
          n1114 = Hexadecimal String To Number(string=w2409) -> (number=w2410:u32)  [unwired: 2 in, 1 out]
          n1115 = Hexadecimal String To Number(string=w2429) -> (number=w2428:u32)  [unwired: 2 in, 1 out]
          n1116 = Hexadecimal String To Number(string=w2399) -> (number=w2396:u32)  [unwired: 2 in, 1 out]
          n1117 = Hexadecimal String To Number(string=w2403) -> (number=w2404:u32)  [unwired: 2 in, 1 out]
          n1118 = Hexadecimal String To Number(string=w2406) -> (number=w2407:u32)  [unwired: 2 in, 1 out]
          n1119 = To Double Precision Float(number=w2428) -> (double precision float=w2425:dbl)
          n1120 = To Double Precision Float(number=w2410) -> (double precision float=w2393:dbl)
          n1121 = To Double Precision Float(number=w2404) -> (double precision float=w2377:dbl)
          n1122 = To Double Precision Float(number=w2407) -> (double precision float=w2395:dbl)
          n1123 = To Unsigned Word Integer(number=w2396) -> (unsigned 16bit integer=→"ECS State":u16)
          n1124 = To Double Precision Float(number=u32 10 ("y")) -> (double precision float=w2426:dbl)
          n1125 = Subtract(x=w2393, y=50.0 ("x")) -> (x-y=w2364:dbl)
          n1126 = Subtract(x=w2395, y=50.0 ("x")) -> (x-y=w2362:dbl)
          n1127 = Divide(x=w2425, y=w2426) -> (x/y=w2369:dbl)
          n1128 = Less Than 0?(x=w2362) -> (x < 0?=w2363:bool)
          n1129 = Equal?(x=u32 417408815, y=w2380) -> (x = y?=w2381:bool)
          n1130 = Equal?(x=u32 417408831, y=w2380) -> (x = y?=w2383:bool)
          n1131 = Equal?(x=u32 417408863, y=w2380) -> (x = y?=w2382:bool)
          n1132 = Less Than 0?(x=w2364) -> (x < 0?=w2365:bool)
          n1133 = call "Filter (SubVI).vi"("Delta"=5000.0, "NewVal"=w2377, "OldVal"=w2378) -> ("Val"=w2375:dbl)  [unwired: 8 in]
          "Motor Speed RPM" <- w2375
          n1134 = Select(t=w2361, s=w2363, f=w2362) -> (s? t:f=w2360:dbl)
          n1135 = Select(t=w2356, s=w2365, f=w2364) -> (s? t:f=w2355:dbl)
          n1136 = Compound Arithmetic op=OR(w2383, w2382, w2381) -> (w2379:bool)
          n1137 = call "Filter (SubVI).vi"("Delta"=130.0, "NewVal"=w2360, "OldVal"=w2361) -> ("Val"=w2358:dbl)  [unwired: 8 in]
          "Motor Stator Temp." <- w2358
          n1138 = call "Filter (SubVI).vi"("Delta"=100.0, "NewVal"=w2355, "OldVal"=w2356) -> ("Val"=w2357:dbl)  [unwired: 8 in]
          "Power transistor Heat sink Temp." <- w2357
          n1139 = call "Filter (SubVI).vi"("Delta"=15.0, "NewVal"=w2369, "OldVal"=w2367) -> ("Val"=w2366:dbl)  [unwired: 8 in]
          "DC Voltage" <- w2366
          n1140 = call "Filter (SubVI).vi"("Delta"=15.0, "NewVal"=w2373, "OldVal"=w2370) -> ("Val"=w2371:dbl)  [unwired: 8 in]
          "DC Current" <- w2371
          n1141 = case shown="True" w2379 {
            tunnel: w2391 -> [w2431 w2434]
            tunnel: [w2431 w2433] -> w2390
            tunnel: w2377 -> [_ w2432]
            frame False {
            }
            frame True {
              n1142 = disable-structure shown="Disabled" {
                disable-tunnel: w2432 -> [w2438 _]
                frame Disabled {
                  n1143 = call <vilib>:"Application Directory.vi"() -> ("Application Directory"=w2436:path)
                  n1144 = Build Path(base path=w2436, name or relative path="RPM Log.lvm") -> (appended path=w2437:path)
                  n1145 = call "Write To Measurement File"("Signals"=w2438, "Filename"=w2437) -> ()  [unwired: 15 in, 3 out]
                }
                frame Enabled {
                }
              }
              n1146 = Build Array (concatenate)(w2432, w2434) -> (w2433:dbl[])
              "Waveform Chart" <- w2433
            }
          }
        }
        frame 1 {
          # "Framde ID\n0x18E3273F"
          n1147 = control-ref of="UUT"() -> (w2445:refnum<vi>)
          n1148 = property on="Property Node" class="DigNum (strict)"(reference=w2445) -> ("Value"=w2446:u8)  [unwired: 1 in, 2 out]
          n1149 = Index Array(array=w2456, index #1=0 ("index"), index #2=1 ("index")) -> (element #1=w2454:u8, element #2=w2448:u8)
          n1150 = Number To Boolean Array(number=w2454) -> (Boolean array=w2453:bool[])
          n1151 = Number To Boolean Array(number=w2448) -> (Boolean array=w2450:bool[])
          n1152 = Boolean To (0,1)(Boolean=w2450) -> (0, 1=w2447:i16[])
          n1153 = Boolean To (0,1)(Boolean=w2453) -> (0, 1=w2452:i16[])
          n1154 = case shown="95" w2446 {
            tunnel: w2447 -> [_ w2457]
            frame 0, Default {
            }
            frame 95 {
              n1155 = for {
                tunnel: w2457 -> [w2462] mode=indexing
                i -> [w2458]
                stop <- w2460 stop-if-true
                n1156 = Not Equal To 0?(x=w2462) -> (x != 0?=w2461:bool)
                n1157 = case shown="0, Default" w2458 {
                  tunnel: w2461 -> [w2463 w2464]
                  frame 0, Default {
                    "Ambient Sensor temp" <- w2463
                  }
                  frame 1 {
                    "Ambient Over temp" <- w2464
                  }
                }
                n1158 = Equal?(x=w2458, y=1.0) -> (x = y?=w2460:bool)
              }
            }
          }
          n1159 = for {
            tunnel: w2452 -> [w2466] mode=indexing
            i -> [w2467]
            n1160 = Not Equal To 0?(x=w2466) -> (x != 0?=w2465:bool)
            n1161 = case shown="2" w2467 {
              tunnel: w2465 -> [w2468 w2469 w2470 w2471 w2472 w2473 w2474 w2475]
              frame 0, Default {
                "Drive Sensor temp Failure" <- w2468
              }
              frame 1 {
                "Drive Over temperature" <- w2469
              }
              frame 2 {
                "Motor Sensor temp Fauilre" <- w2470
              }
              frame 3 {
                "Motor Over temperature" <- w2471
              }
              frame 4 {
                "Derated drive temp" <- w2472
              }
              frame 5 {
                "Under voltage/Over voltage" <- w2473
              }
              frame 6 {
                "Commutation err" <- w2474
              }
              frame 7 {
                "Speed error" <- w2475
              }
            }
          }
        }
        frame 2 {
          # "Frame ID\n0x18E2273F"
          n1162 = Index Array(array=w2496, index #1=0 ("index"), index #2=1 ("index")) -> (element #1=w2493:u8, element #2=w2489:u8)
          n1163 = disable-structure shown="Enabled" {
            disable-tunnel: [w2499 w2500] -> w2494
            disable-tunnel: w2493 -> [w2498 w2500]
            frame Disabled {
              n1164 = Number To Hexadecimal String(2:w2498) -> (0:w2497:string)  [unwired: 1 in]
              n1165 = Hexadecimal String To Number(string=w2497) -> (number=w2499:u32)  [unwired: 2 in, 1 out]
            }
            frame Enabled {
            }
          }
          n1166 = Number To Hexadecimal String(2:w2489) -> (0:w2487:string)  [unwired: 1 in]
          n1167 = Hexadecimal String To Number(string=w2487) -> (number=w2488:u32)  [unwired: 2 in, 1 out]
          n1168 = To Double Precision Float(number=w2488) -> (double precision float=w2486:dbl)
          n1169 = To Double Precision Float(number=w2494) -> (double precision float=→"Motor Phase Current RMS":dbl)
          n1170 = Subtract(x=w2486, y=50.0) -> (x-y=w2478:dbl)
          n1171 = Less Than 0?(x=w2478) -> (x < 0?=w2479:bool)
          n1172 = Select(t=w2477, s=w2479, f=w2478) -> (s? t:f=w2476:dbl)
          "Ambient Temperature" <- w2476
        }
      }
    }
  }
  n1173 = case shown="True" w6 {
    selector: w6 -> [w2505 w2507]
    frame False {
      n1174 = property on="Settings" class="Bool"("Visible"=w2505) -> ()  [unwired: 2 in, 2 out]
      n1175 = property on="Cal Value" class="Str"("Visible"=w2505) -> ()  [unwired: 2 in, 2 out]
      n1176 = property on="Stop Burn-in" class="Bool"("Visible"=w2505) -> ()  [unwired: 2 in, 2 out]
      n1177 = property on="Index" class="Str"("Visible"=w2505, "Value"="5" ("Index")) -> ()  [unwired: 2 in, 2 out]
    }
    frame True {
      n1178 = property on="Settings" class="Bool"("Visible"=w2507) -> ()  [unwired: 2 in, 2 out]
      n1179 = property on="Cal Value" class="Str"("Visible"=w2507) -> ()  [unwired: 2 in, 2 out]
      n1180 = property on="Index" class="Str"("Visible"=w2507, "Value"="5" ("Index")) -> ()  [unwired: 2 in, 2 out]
      n1181 = property on="Stop Burn-in" class="Bool"("Visible"=w2507) -> ()  [unwired: 2 in, 2 out]
    }
  }
  n1182 = local write "Next SN"(w2) -> ()
  n1183 = control-ref of="This VI"() -> (w5:refnum<vi>)
  n1184 = register-events "Register For Events"(w5) -> (reference out=w4:refnum<event-registration>)  [unwired: 2 in, 1 out]
  n1185 = local write "ClosePanel"(w1) -> ()
  n1186 = while {
    shift-right: [w2528] -> _
    shift-left: T12."Initialize" -> [w2527]
    shift-right: [w2512] -> _
    shift-left: "" -> [w2515]
    shift-right: [w2523] -> _
    shift-left: _ -> [w2522]
    shift-right: [w2521] -> _
    shift-left: w23 -> [w2519]
    shift-right: [w2520] -> _
    shift-left: refnum<vi> refnum ("Config_CANAT") -> [w2518]
    shift-right: [w2516] -> _
    shift-left: w19 -> [w2517]
    tunnel: w12 -> [_]
    tunnel: w11 -> [w2514]
    tunnel: w10 -> [w2513]
    tunnel: w13 -> [w2525]
    tunnel: [w2524] -> _
    tunnel: w9 -> [_]
    tunnel: w8 -> [w2511]
    tunnel: w4 -> [w2510]
    shift-right: [w2508] -> _
    shift-left: 1 -> [w2509]
    tunnel: w2 -> [_]
    tunnel: w1 -> [_]
    stop <- w2526 stop-if-true
    n1187 = case shown="\"MainProgram\"" w2527 {
      tunnel: [T12."MainProgram" w2715 w2848 T12."Erase ATR Table"] -> w2528
      tunnel: [FALSE w2716 FALSE FALSE] -> w2526
      tunnel: [w2535 w2705 w2842 w3846] -> w2524
      tunnel: w2525 -> [_ w2702 w2846 _]
      tunnel: ["Initialization State..." w2713 w2830 "Initialization State..."] -> w2512
      tunnel: [w2581 w2710 w2843 w3857] -> w2523
      tunnel: w2522 -> [w2581 w2712 w2844 _]
      tunnel: [w2570 w2711 w2838 w3851] -> w2521
      tunnel: [w2569 w2709 w2839 w3853] -> w2520
      tunnel: w2519 -> [w2570 w2714 w2841 w3851]
      tunnel: w2518 -> [w2569 w2706 w2840 _]
      tunnel: w2517 -> [w2568 w2708 w2837 w3850]
      tunnel: [w2568 w2707 w2836 w3850] -> w2516
      tunnel: w2515 -> [_ w2703 w2832 _]
      tunnel: w2514 -> [_ _ w2835 _]
      tunnel: w2513 -> [w2542 _ w2829 _]
      tunnel: w2511 -> [_ _ w2828 _]
      tunnel: w2510 -> [_ _ w2827 _]
      tunnel: w2509 -> [w2534 w2699 w2826 w3845]
      tunnel: [w2534 w2699 w2825 w3845] -> w2508
      frame "Erase ATR Table", Default {
        w2539 = T13."Enabled" ("Disabled")
        w2550 = "Marvin" ("section")
        w2564 = refnum<visa-resource-name> "COM1" ("VISA resource name")
        w2576 = FALSE ("Visible")
        # "2"
        # "Venbale"
        # "Power ON"
        n1188 = call <vilib>:"Open Config Data.vi"("create file if necessary (T)"=FALSE, "configuration file path"=w2542) -> ("refnum"=w2540:T15)  [unwired: 7 in, 2 out]
        n1189 = property on="Serial Com" class="Bool"(error in=errorcluster {"status"=FALSE, "code"=0, "source"=""} ("error out"), "Visible"=TRUE) -> (error out=w2565:errorcluster)  [unwired: 1 in, 1 out]
        n1190 = case shown="False" w2552 {
          tunnel: ["AHU Software Version" ("key") "EBAY Software Version" ("key")] -> w2549
          tunnel: ["AHU Serial Number" ("key") "EBAY Serial Number" ("key")] -> w2548
          frame False {
          }
          frame True {
          }
        }
        n1191 = property on="VISA resource name" class="VISAName"(error in=w2565, "Visible"=w2576, "Value"=w2564) -> (error out=w2578:errorcluster)  [unwired: 1 in, 1 out]
        n1192 = property on="VISA resource name" class="VISAName"(error in=w2565, "Value"=w2564) -> ()  [unwired: 1 in, 2 out]
        n1193 = property on="Serial" class="Bool (strict)"(error in=w2578, "Value"=w2576) -> (error out=w2572:errorcluster)  [unwired: 1 in, 1 out]
        n1194 = flat-sequence {
          tunnel: [w2675] -> w2552
          tunnel: w2572 -> [w2674]
          tunnel: [w2673] -> w2546
          frame #0 {
            n1195 = disable-structure shown="Disabled" {
              frame Disabled {
                n1196 = Two Button Dialog(message="Please select the Unit Under Test.", 1:"AHU" ("F button name (\"Cancel\")"), 2:"EBAY" ("T button name (\"OK\")")) -> ()  [unwired: 1 out]
              }
              frame Enabled {
              }
            }
            n1197 = call "Select UUT"("error in (no error)"=w2674) -> ("EBAY"=w2675:bool, "error out"=w2673:errorcluster)  [unwired: 17 in]
          }
        }
        n1198 = call-poly <vilib>:"Read Key.vi"("section"=w2550, "error in (no error)"=w2546, "key"=w2549, "refnum"=w2540) -> ("error out"=w2547:errorcluster, "value"=→"SoftwareVer":string, "refnum out"=w2551:T15)  [unwired: 2 in, 3 out]
        n1199 = call-poly <vilib>:"Read Key.vi"("section"=w2550, "error in (no error)"=w2547, "key"=w2548, "refnum"=w2551) -> ("value"=w2545:string)  [unwired: 2 in, 5 out]
        n1200 = Decimal String To Number(string=w2545) -> (number=w2544:i32)  [unwired: 2 in, 1 out]
        n1201 = Increment(x=w2544) -> (x+1=w2533:i32)
        n1202 = Number To Decimal String(number=w2533) -> (decimal integer string=→"Next SN":string)  [unwired: 1 in]
        n1203 = case shown="False" w2552 {
          tunnel: [string[][] [["6.1", "Visual Inspection", "", "", "", "", ""], ["6.1.1", "Verification of Components Not Installed", "N/A", "-", "", "", ""], ["", "", "", "", "", "", ""], ["6.1.2", "Manufacturing Defects", "N/A", "-", "", "", ""], ["", "", "", "", "", "", ""], ["6.2", "Power Supply Testing", "", "", "", "", ""], ["6.2.1", "Input Current Drawn", "", "", "", "", ""], ["6.2.1.1", "DC Input Current", "< 150", "-", "mA", "", ""], ["", "", "", "", "", "", ""], ["6.2.2", "Power Supply Voltages", "", "", "", "", ""], ["6.2.2.1", "12V", "12.0", "+/-0.500", "V", "", ""], ["6.2.2.2", "5V", "5.0", "+/-0.200", "V", "", ""], ["6.2.2.3", "3.3V", "3.3", "+/-0.100", "V", "", ""], ["6.2.2.4", "1.8V", "1.8", "+/-0.100", "V", "", ""], ["", "", "", "", "", "", ""], ["7", "Functional Test Procedure", "", "", "", "", ""], ["7.1", "Weight Check", "3800", "+/-100.0", "gr", "", ""], ["", "", "", "", "", "", ""], ["7.2", "Insulation Resistance Test", "", "", "", "", ""], ["7.2.1", "J3.B to Chassis", "> 1M", "-", "W", "", ""], ["7.2.2", "J1.16 to Chassis", "> 100K", "-", "W", "", ""], ["", "", "", "", "", "", ""], ["7.2", "Bonding Resistance", "", "", "", "", ""], ["7.2.3", "J1 Body to Chassis", "< 2m", "-", "W", "", ""], ["7.2.4", "J2  Body to Chassis", "< 2m", "-", "W", "", ""], ["7.2.5", "J3  Body to Chassis", "< 2m", "-", "W", "", ""], ["", "", "", "", "", "", ""], ["7.2.1", "CANbus Resistance Test", "", "", "", "", ""], ["7.2.1.1", "J1.17 to J1.18", "> 10K", "-", "W", "", ""], ["", "", "", "", "", "", ""], ["7.3", "Sealing Test", "N/A", "-", "", "", ""], ["", "", "", "", "", "", ""], ["7.4", "Communication Test", "", "", "", "", ""], ["7.4.1", "Serial RS-232", "N/A", "-", "", "gf", "hfg"], ["7.4.2", "CAN Bus", "N/A", "-", "", "hfg", "hfg"], ["", "", "", "", "", "", ""], ["7.5", "Performances Tests", "", "", "", "", ""], ["7.5.1", "Reverse Polarity Test", "", "", "", "", ""], ["7.5.1.1", "DC Input Current", "< 1", "-", "mA", "", ""], ["", "", "", "", "", "", ""], ["7.5.2", "Enable Test", "", "", "", "", ""], ["7.5.2.1", "Fan Speed at Opened Enable ", "5000", "+/-200.0", "rpm", "", ""], ["7.5.2.2", "Fan Speed at Opened Enable ", "0", "+/-200.0", "rpm", "", ""], ["7.5.2.3", "Fan Speed at Closed Enable ", "5000", "+/-200.0", "rpm", "", ""], ["7.5.2.4", "Motor Rotation Direction", "Counter-clockwise (Inlet)", "-", "", "", ""], ["", "", "", "", "", "", ""], ["7.5.3", "Stop Time Test ", "", "", "", "", ""], ["7.5.3.1", "Motor Stop time", "< 50", "-", "sec", "", ""], ["", "", "", "", "", "", ""], ["7.5.4", "Speed Command Test", "", "", "", "", ""], ["7.5.4.1", "Fan Speed", "6000", "+/-200.0", "rpm", "", ""], ["7.5.4.2", "Fan Speed", "9000", "+/-200.0", "rpm", "", ""], ["7.5.4.3", "Fan Speed", "12100", "+/-200.0", "rpm", "", ""], ["", "", "", "", "", "", ""], ["7.5.5", "Temperature Sensor Calibration Test", "", "", "", "", ""], ["7.5.5.1", "Sensor Reading Analog Offset", "0", "+/-0.100", ".", "", ""], ["", "", "", "", "", "", ""], ["7.5.6", "Burn-in Test", "", "", "", "", ""], ["7.5.6.1", "DC Input Current", "28", "+/-5.000", "A", "", ""], ["7.5.6.2", "Ambient Temperature", "25", "+/-13.00", "ºC", "", ""], ["7.5.6.3", "After 10 min of operation", "", "", "ºC", "", ""], ["7.5.6.4", "After 20 min of operation", "", "", "ºC", "", ""], ["7.5.6.5", "After 30 min of operation", "", "", "ºC", "", ""], ["", "", "", "", "", "", ""], ["9", "Motor Temp. Test", "", "", "", "", ""], ["9.1", "60 Degree", "60", "+/-3.00", "ºC", "", ""], ["9.2", "90 Degree", "90", "+/-3.00", "ºC", "", ""], ["9.3", "110 Degree", "110", "+/-3.00", "ºC", "", ""]] ("data") string[][] [["6.1", "Visual Inspection", "", "", "", "", ""], ["6.1.1", "Verification of Components Not Installed", "N/A", "-", "", "", ""], ["", "", "", "", "", "", ""], ["6.1.2", "Manufacturing Defects", "N/A", "-", "", "", ""], ["", "", "", "", "", "", ""], ["6.2", "Power Supply Testing", "", "", "", "", ""], ["6.2.1", "Input Current Drawn", "", "", "", "", ""], ["6.2.1.1", "DC Input Current", "< 150", "-", "mA", "", ""], ["", "", "", "", "", "", ""], ["6.2.2", "Power Supply Voltages", "", "", "", "", ""], ["6.2.2.1", "12V", "12.0", "+/-0.500", "V", "", ""], ["6.2.2.2", "5V", "5.0", "+/-0.200", "V", "", ""], ["6.2.2.3", "3.3V", "3.3", "+/-0.100", "V", "", ""], ["6.2.2.4", "1.8V", "1.8", "+/-0.100", "V", "", ""], ["", "", "", "", "", "", ""], ["7", "Functional Test Procedure", "", "", "", "", ""], ["7.1", "Weight Check", "4180", "+/-10.00", "gr", "", ""], ["", "", "", "", "", "", ""], ["7.2", "Insulation Resistance Test", "", "", "", "", ""], ["7.2.1", "J3.B to Chassis", "> 1M", "-", "W", "", ""], ["7.2.2", "J1.16 to Chassis", "> 100K", "-", "W", "", ""], ["", "", "", "", "", "", ""], ["7.2", "Bonding Resistance", "", "", "", "", ""], ["7.2.3", "J1 Body to Chassis", "< 2m", "-", "W", "", ""], ["7.2.4", "J2  Body to Chassis", "< 2m", "-", "W", "", ""], ["7.2.5", "J3  Body to Chassis", "< 2m", "-", "W", "", ""], ["", "", "", "", "", "", ""], ["7.2.1", "CANbus Resistance Test", "", "", "", "", ""], ["7.2.1.1", "J1.17 to J1.18", "> 10K", "-", "W", "", ""], ["", "", "", "", "", "", ""], ["7.3", "Sealing Test", "N/A", "-", "", "", ""], ["", "", "", "", "", "", ""], ["7.4", "Communication Test", "", "", "", "", ""], ["7.4.1", "Serial RS-232", "N/A", "-", "", "", ""], ["7.4.2", "CAN Bus", "N/A", "-", "", "", ""], ["", "", "", "", "", "", ""], ["7.5", "Performances Tests", "", "", "", "", ""], ["7.5.1", "Reverse Polarity Test", "", "", "", "", ""], ["7.5.1.1", "DC Input Current", "< 1", "-", "mA", "", ""], ["", "", "", "", "", "", ""], ["7.5.2", "Enable Test", "", "", "", "", ""], ["7.5.2.1", "Fan Speed before Opened Enable ", "5000", "+/-200.0", "rpm", "", ""], ["7.5.2.2", "Fan Speed at Opened Enable ", "0", "+/-200.0", "rpm", "", ""], ["7.5.2.3", "Fan Speed at Closed Enable ", "5000", "+/-200.0", "rpm", "", ""], ["7.5.2.4", "Motor Rotation Direction", "Counter-clockwise (Inlet)", "-", "", "", ""], ["", "", "", "", "", "", ""], ["7.5.3", "Stop Time Test ", "", "", "", "", ""], ["7.5.3.1", "Motor Stop time", "< 50", "-", "sec", "", ""], ["", "", "", "", "", "", ""], ["7.5.4", "Speed Command Test", "", "", "", "", ""], ["7.5.4.1", "Fan Speed", "6000", "+/-200.0", "rpm", "", ""], ["7.5.4.2", "Fan Speed", "11500", "+/-200.0", "rpm", "", ""], ["7.5.4.3", "Fan Speed", "15100", "+/-200.0", "rpm", "", ""], ["", "", "", "", "", "", ""], ["7.5.5", "Temperature Sensor Calibration Test", "", "", "", "", ""], ["7.5.5.1", "Sensor Reading Analog Offset", "0", "+/-0.100", ".", "", ""], ["", "", "", "", "", "", ""], ["7.5.6", "Temperature Control Algorithm Test", "", "", "", "", ""], ["7.5.6.1", "Tair <   68 ± 2 oC", "6000", "+/-200.0", "rpm", "", ""], ["7.5.6.2", "Measured Temp.", "", "", "ºC", "", ""], ["7.5.6.3", "Tair >= 68 ± 2 oC", "11500", "+/-200.0", "rpm", "", ""], ["7.5.6.4", "Transition Temp.", "", "", "ºC.", "", ""], ["7.5.6.5", "Tair >= 88 ± 2 oC", "15100", "+/-400.0", "rpm", "", ""], ["7.5.6.6", "Transition Temp.", "", "", "ºC", "", ""], ["7.5.6.7", "Tair <= 80 ± 2 oC", "11500", "+/-200.0", "rpm", "", ""], ["7.5.6.8", "Transition Temp.", "", "", "ºC", "", ""], ["7.5.6.9", "Tair <= 60 ± 2 oC", "6000", "+/-200.0", "rpm", "", ""], ["7.5.6.10", "Transition Temp.", "", "", "ºC", "", ""], ["", "", "", "", "", "", ""], ["7.5.7", "Burn-in Test", "", "", "", "", ""], ["7.5.7.1", "DC Input Current", "50", "+/-7.000", "A", "", ""], ["7.5.7.2", "Fan Speed", "15100", "+/-400.0", "rpm", "", ""], ["7.5.7.3", "Ambient Temperature", "25", "+/-13.00", "ºC", "", ""], ["7.5.7.4", "After 10 min of operation", "", "-", "ºC", "", ""], ["7.5.7.5", "After 20 min of operation", "", "-", "ºC", "", ""], ["7.5.7.6", "After 30 min of operation", "", "-", "ºC", "", ""], ["", "", "", "", "", "", ""], ["8", "Auxiliary Fan Test", "", "", "", "", ""], ["8.1", "Auxiliary Cooling Fan ON", "60", "+/-2.00", "ºC", "", ""], ["8.2", "Fan status", "ON", "-", "-", "", ""], ["8.3", "Auxiliary Cooling Fan OFF", "55", "+/-2.00", "ºC", "", ""], ["8.4", "Fan status", "OFF", "-", "-", "", ""], ["", "", "", "", "", "", ""], ["9", "Motor Temp. Test", "", "", "", "", ""], ["9.1", "60 Degree", "60", "+/-3.00", "ºC", "", ""], ["9.2", "90 Degree", "90", "+/-3.00", "ºC", "", ""], ["9.3", "110 Degree", "110", "+/-3.00", "ºC", "", ""]] ("data")] -> w2574
          tunnel: ["AHU" "EBAY"] -> w2573
          tunnel: [w2679 w2682] -> w2571
          tunnel: w2546 -> [w2679 w2682]
          frame False {
          }
          frame True {
          }
        }
        "UUT" <- w2573
        n1204 = for {
          tunnel: w2574 -> [w2689] mode=indexing
          tunnel: w2571 -> [w2687]
          tunnel: [w2686] -> w2567
          tunnel: w2574 -> [w2685]
          i -> [w2688]
          n1205 = for {
            tunnel: w2689 -> [_] mode=indexing
            tunnel: w2688 -> [w2695]
            tunnel: w2687 -> [w2692]
            tunnel: [w2691] -> w2686
            tunnel: w2685 -> [w2690]
            i -> [w2696]
            n1206 = Bundle By Name(cluster=T16 {"Row"=0, "Column"=0} ("Active Cell:Active Cell"), "Row"=w2695, "Column"=w2696) -> (w2694:T16)
            n1207 = control-ref of="ATR"() -> (w2693:refnum<vi>)
            n1208 = property class="Tbl (strict)"(reference=w2693, error in=w2692, "Active Cell"=w2694, "Cell BG Color"=u32 16777226, "Value"=w2690) -> (error out=w2691:errorcluster)  [unwired: 1 out]
          }
        }
        n1209 = property on="Automation" class="Bool (strict)"("Value"=FALSE ("Automation")) -> ()  [unwired: 2 in, 2 out]
        n1210 = call "COM EvolutionBoard.vi"("error in (no error)"=w2567, "VISA resource name 2"=refnum<visa-resource-name> "COM1" ("VISA resource name")) -> ("error out"=w2556:errorcluster, ".not. x?"=w2557:bool, "VISA resource name out"=w2554:refnum<visa-resource-name>)  [unwired: 7 in]
        "VISA resource name out" <- w2554
        n1211 = Byte Array To String(unsigned byte array=u8[] [75, 0, 4, 2, 0, 0, 0, 0] ("appended array")) -> (string=w2559:string)
        n1212 = Byte Array To String(unsigned byte array=u8[] [75, 0, 4, 2, 0, 0, 0, 0] ("appended array")) -> (string=w2563:string)
        n1213 = case shown="True" w2557 {
          tunnel: w2556 -> [w2588 w2594]
          tunnel: [w2587 w2591] -> w2555
          tunnel: w2554 -> [w2586 w2595]
          tunnel: [w2586 w2590] -> w2553
          frame False {
            n1214 = call "Display Message to User4"("error in (no error)"=w2588) -> ("error out"=w2587:errorcluster)  [unwired: 9 in, 1 out]
          }
          frame True {
            n1215 = Byte Array To String(unsigned byte array=u8[] [75, 0, 4, 17, 0, 0, 0, 0] ("appended array")) -> (string=w2598:string)
            n1216 = VISA Write(VISA resource name=w2595, write buffer=w2598, error in (no error)=w2594) -> (VISA resource name out=w2593:refnum<visa-resource-name>, error out=w2599:errorcluster)  [unwired: 1 out]
            n1217 = while {
              tunnel: w2593 -> [w2613]
              tunnel: w2597 -> [w2612]
              tunnel: [w2611] -> w2590
              tunnel: [w2610] -> w2591
              tunnel: w2592 -> [w2608]
              tunnel: [w2602] -> w2589
              stop <- w2604 stop-if-true
              n1218 = VISA Read(VISA resource name=w2613, byte count=u32 1, error in (no error)=w2612) -> (VISA resource name out=w2615:refnum<visa-resource-name>, read buffer=w2616:string, error out=w2614:errorcluster)  [unwired: 1 out]
              n1219 = String To Byte Array(string=w2616) -> (unsigned byte array=w2619:u8[])
              n1220 = Index Array(array=w2619, index=0) -> (element=w2617:u8)
              n1221 = call <vilib>:"High Resolution Relative Seconds.vi"() -> ("relative seconds"=w2609:dbl)
              n1222 = Subtract(x=w2609, y=w2608) -> (x-y=w2607:dbl)
              n1223 = Greater Or Equal?(x=w2607, y=10.0) -> (x >= y?=w2605:bool)
              n1224 = case shown="75" w2617 {
                tunnel: [w2624 w2628] -> w2610
                tunnel: w2615 -> [w2623 w2637]
                tunnel: w2614 -> [w2624 w2636]
                tunnel: [w2623 w2629] -> w2611
                tunnel: [u32 9999 w2626] -> w2602
                tunnel: [FALSE w2625] -> w2603
                frame 0, Default {
                }
                frame 75 {
                  n1225 = VISA Read(VISA resource name=w2637, byte count=u32 3, error in (no error)=w2636) -> (VISA resource name out=w2632:refnum<visa-resource-name>, read buffer=w2640:string, error out=w2631:errorcluster)  [unwired: 1 out]
                  n1226 = String To Byte Array(string=w2640) -> (unsigned byte array=w2630:u8[])
                  n1227 = Index Array(array=w2630, index #1=0 ("index")) -> (element #1=w2635:u8, element #2=w2633:u8)  [unwired: 2 in, 1 out]
                  n1228 = Equal?(x=u8 0, y=w2635) -> (x = y?=w2634:bool)
                  n1229 = case shown="True" w2634 {
                    tunnel: [w2643 w2650] -> w2628
                    tunnel: w2633 -> [_ w2657]
                    tunnel: w2632 -> [w2644 w2656]
                    tunnel: w2631 -> [w2643 w2655]
                    tunnel: w2630 -> [_ w2654]
                    tunnel: [w2644 w2652] -> w2629
                    tunnel: [u32 9999 w2646] -> w2626
                    tunnel: [FALSE w2645] -> w2625
                    frame False {
                    }
                    frame True {
                      n1230 = VISA Read(VISA resource name=w2656, byte count=w2657, error in (no error)=w2655) -> (VISA resource name out=w2652:refnum<visa-resource-name>, read buffer=w2651:string, error out=w2650:errorcluster)  [unwired: 1 out]
                      n1231 = String To Byte Array(string=w2651) -> (unsigned byte array=w2653:u8[])
                      n1232 = Insert Into Array(array=w2654, new element=w2653) -> (w2647:u8[])  [unwired: 1 in]
                      n1233 = Index Array(array=w2647, index #1=0 ("index")) -> (element #3=w2648:u8)  [unwired: 2 in, 2 out]
                      n1234 = case shown="15..19" w2648 {
                        tunnel: w2647 -> [_ w2671]
                        tunnel: [u32 9999 w2660] -> w2646
                        tunnel: [FALSE w2661] -> w2645
                        frame 0, Default {
                        }
                        frame 15..19 {
                          n1235 = Index Array(array=w2671, index #1=3 ("index")) -> (element #1=w2670:u8, element #2=w2669:u8, element #3=w2668:u8, element #4=w2667:u8)  [unwired: 3 in]
                          n1236 = Join Numbers(hi=w2669, lo=w2670) -> ((hi.lo)=w2666:u16)
                          n1237 = Join Numbers(hi=w2667, lo=w2668) -> ((hi.lo)=w2665:u16)
                          n1238 = Join Numbers(hi=w2665, lo=w2666) -> ((hi.lo)=w2663:u32)
                          n1239 = Multiply(x=0.02003173828125, y=w2663) -> (x*y=w2660:dbl)
                          n1240 = Greater Or Equal?(x=w2660, y=0.0) -> (x >= y?=w2661:bool)
                        }
                      }
                    }
                  }
                }
              }
              n1241 = Compound Arithmetic op=OR(w2605, w2603) -> (w2604:bool)
            }
            "CurrentOffset" <- w2589
            n1242 = flat-sequence {
              tunnel: w2599 -> [w2601]
              tunnel: [w2601] -> w2597
              tunnel: [w2600] -> w2592
              frame #0 {
                n1243 = call <vilib>:"High Resolution Relative Seconds.vi"() -> ("relative seconds"=w2600:dbl)
              }
            }
          }
        }
        n1244 = VISA Write(VISA resource name=w2553, write buffer=w2563, error in (no error)=w2555) -> (error out=w2561:errorcluster)  [unwired: 2 out]
        n1245 = call "Time Delay5"("error in (no error)"=w2561) -> ("error out"=w2560:errorcluster)  [unwired: 10 in]
        n1246 = VISA Write(VISA resource name=w2553, write buffer=w2559, error in (no error)=w2560) -> (error out=w2536:errorcluster)  [unwired: 2 out]
        n1247 = call <vilib>:"Clear Errors.vi"("error in (no error)"=w2536) -> ("error out"=w2535:errorcluster)  [unwired: 5 in, 1 out]
        n1248 = property on="Start" class="Bool (strict)"(error in=w2535, "DisabledEnum"=w2539) -> (error out=w2538:errorcluster)  [unwired: 1 in, 1 out]
        n1249 = property on="Report" class="Bool (strict)"(error in=w2538, "DisabledEnum"=w2539) -> (error out=w2531:errorcluster)  [unwired: 1 in, 1 out]
        n1250 = property on="ClosePanel" class="Bool (strict)"(error in=w2531, "Value"=FALSE ("ClosePanel")) -> ()  [unwired: 1 in, 2 out]
      }
      frame "Stop" {
        n1251 = disable-structure shown="Disabled" {
          disable-tunnel: w2708 -> [w2720 w2721]
          disable-tunnel: [w2719 w2721] -> w2700
          frame Disabled {
            n1252 = Preview Queue Element(queue=w2720) -> (queue out=w2719:refnum<queue>, element=w2718:T10)  [unwired: 2 in, 2 out]
            n1253 = Unbundle By Name(w2718) -> ("Array Test"=→"Array Test":T1)
          }
          frame Enabled {
          }
        }
        n1254 = property on="Stop Button" class="Bool (strict)"(error in=w2702) -> (error out=w2701:errorcluster, "Value"=w2704:bool)  [unwired: 1 in, 1 out]
        n1255 = case shown="True" w2704 {
          tunnel: [FALSE w2762] -> w2716
          tunnel: [T12."Initialize" w2761] -> w2715
          tunnel: w2714 -> [w2734 w2760]
          tunnel: ["Restarting program..." w2759] -> w2713
          tunnel: w2712 -> [w2743 w2758]
          tunnel: [w2733 w2757] -> w2711
          tunnel: [refnum<visa-resource-name> refnum ("VISA resource name") w2756] -> w2710
          tunnel: [w2723 w2755] -> w2709
          tunnel: w2700 -> [w2732 w2754]
          tunnel: [w2731 w2753] -> w2707
          tunnel: w2701 -> [w2722 w2750]
          tunnel: w2706 -> [w2723 w2752]
          tunnel: [w2735 w2751] -> w2705
          tunnel: w2703 -> [_ _]
          frame False {
            # "K15 OFF + Venable"
            n1256 = Flush Queue(queue=w2734) -> (queue out=w2733:refnum<queue>)  [unwired: 1 in, 2 out]
            n1257 = Flush Queue(queue=w2732) -> (queue out=w2731:refnum<queue>)  [unwired: 1 in, 2 out]
            n1258 = control-ref of="VISA resource name out"() -> (w2741:refnum<vi>)
            n1259 = call "Reset CAN Device.vi"("error in (no error)"=w2722, "Cluster in"=w2723) -> ()  [unwired: 9 in, 1 out]
            n1260 = Merge Errors(w2722) -> (w2735:errorcluster)
            n1261 = VISA Flush I/O Buffer(VISA resource name=w2743, error in (no error)=w2722) -> (VISA resource name out=w2730:refnum<visa-resource-name>, error out=w2724:errorcluster)  [unwired: 1 in]
            n1262 = VISA Close(VISA resource name=w2730, error in (no error)=w2722) -> (error out=w2725:errorcluster)
            n1263 = call <vilib>:"Clear Errors.vi"("error in (no error)"=w2725) -> ()  [unwired: 5 in, 2 out]
            n1264 = call <vilib>:"Clear Errors.vi"("error in (no error)"=w2724) -> ()  [unwired: 5 in, 2 out]
            n1265 = property class="VISAName"(reference=w2741, error in=w2722) -> (error out=w2738:errorcluster, "Value"=w2737:refnum<visa-resource-name>)  [unwired: 1 out]
            n1266 = Byte Array To String(unsigned byte array=u8[] [75, 0, 4, 2, 0, 0, 16, 0] ("appended array")) -> (string=w2740:string)
            n1267 = VISA Write(VISA resource name=w2737, write buffer=w2740, error in (no error)=w2738) -> (VISA resource name out=w2736:refnum<visa-resource-name>, error out=w2728:errorcluster)  [unwired: 1 out]
            n1268 = VISA Flush I/O Buffer(VISA resource name=w2736, error in (no error)=w2728) -> (VISA resource name out=w2729:refnum<visa-resource-name>, error out=w2727:errorcluster)  [unwired: 1 in]
            n1269 = VISA Close(VISA resource name=w2729, error in (no error)=w2727) -> (error out=w2726:errorcluster)
            n1270 = call <vilib>:"Clear Errors.vi"("error in (no error)"=w2726) -> ()  [unwired: 5 in, 2 out]
          }
          frame True {
            n1271 = property on="ClosePanel" class="Bool (strict)"() -> ("Value"=w2747:bool)  [unwired: 2 in, 2 out]
            n1272 = case shown="False" w2747 {
              tunnel: w2750 -> [w2765 w2767]
              tunnel: [w2764 w2767] -> w2749
              tunnel: [w2763 TRUE ("Yes")] -> w2748
              frame False {
                n1273 = call "Display Message to User7"("error in (no error)"=w2765) -> ("error out"=w2764:errorcluster, "Yes"=w2763:bool)  [unwired: 9 in]
              }
              frame True {
              }
            }
            n1274 = case shown="True" w2748 {
              tunnel: [FALSE TRUE] -> w2762
              tunnel: [T12."MainProgram" T12."Stop"] -> w2761
              tunnel: w2760 -> [w2771 w2816]
              tunnel: [w2770 w2792] -> w2751
              tunnel: ["Press \"Start\" to perform test(s)." "Program Stopped...\r\nPlease turn OFF All Power sinks"] -> w2759
              tunnel: w2758 -> [w2781 w2814]
              tunnel: [w2779 refnum<queue> refnum ("queue out")] -> w2757
              tunnel: [w2781 refnum<visa-resource-name> refnum ("VISA resource name")] -> w2756
              tunnel: [w2769 refnum<vi> refnum ("Config_CANAT")] -> w2755
              tunnel: w2754 -> [w2777 w2809]
              tunnel: [w2778 refnum<queue> refnum ("queue out")] -> w2753
              tunnel: w2749 -> [w2770 w2794]
              tunnel: w2752 -> [w2769 w2795]
              tunnel: w2747 -> [_ w2791]
              frame False {
                n1275 = call "Clear CAN Buffer.vi"("error in (no error)"=w2770, "Cluster in"=w2769) -> ()  [unwired: 8 in, 2 out]
                n1276 = Flush Queue(queue=w2771) -> (queue out=w2779:refnum<queue>)  [unwired: 1 in, 2 out]
                n1277 = property on="f" class="Enum (strict)"(error in=w2770) -> (error out=w2773:errorcluster, "Value"=w2776:T2)  [unwired: 1 in, 1 out]
                n1278 = Equal?(x=w2776, y=T2."Empty") -> (x = y?=w2774:bool)
                n1279 = case shown="False" w2774 {
                  tunnel: [w2784 w2785] -> w2768
                  tunnel: w2773 -> [w2784 w2785]
                  frame False {
                  }
                  frame True {
                  }
                }
                n1280 = property on="Stop Button" class="Bool (strict)"(error in=w2768, "Value"=FALSE ("Stop Button")) -> ()  [unwired: 1 in, 2 out]
                n1281 = Flush Queue(queue=w2777, error in (no error)=w2768) -> (queue out=w2778:refnum<queue>)  [unwired: 2 out]
              }
              frame True {
                # "K15 OFF + Venable"
                n1282 = call "Close CAN Device.vi"("error in (no error)"=w2794, "Cluster in"=w2795) -> ()  [unwired: 8 in, 2 out]
                n1283 = control-ref of="VISA resource name out"() -> (w2808:refnum<vi>)
                n1284 = Flush Queue(queue=w2816, error in (no error)=w2794) -> (queue out=w2787:refnum<queue>, error out=w2817:errorcluster)  [unwired: 1 out]
                n1285 = Release Queue(queue=w2787, force destroy? (F)=TRUE, error in (no error)=w2817) -> (error out=w2788:errorcluster)  [unwired: 2 out]
                n1286 = VISA Close(VISA resource name=w2814, error in (no error)=w2794) -> (error out=w2798:errorcluster)
                n1287 = Flush Queue(queue=w2809, error in (no error)=w2794) -> (queue out=w2786:refnum<queue>, error out=w2810:errorcluster)  [unwired: 1 out]
                n1288 = call <vilib>:"Clear Errors.vi"("error in (no error)"=w2810) -> ("error out"=w2800:errorcluster)  [unwired: 5 in, 1 out]
                n1289 = Release Queue(queue=w2786, force destroy? (F)=TRUE, error in (no error)=w2800) -> (error out=w2797:errorcluster)  [unwired: 2 out]
                n1290 = property class="VISAName"(reference=w2808, error in=w2794) -> (error out=w2804:errorcluster, "Value"=w2803:refnum<visa-resource-name>)  [unwired: 1 out]
                n1291 = Byte Array To String(unsigned byte array=u8[] [75, 0, 4, 2, 0, 0, 16, 0] ("appended array")) -> (string=w2806:string)
                n1292 = VISA Write(VISA resource name=w2803, write buffer=w2806, error in (no error)=w2804) -> (VISA resource name out=w2802:refnum<visa-resource-name>, error out=w2801:errorcluster)  [unwired: 1 out]
                n1293 = VISA Close(VISA resource name=w2802, error in (no error)=w2801) -> (error out=w2799:errorcluster)
                n1294 = Merge Errors(w2788, w2799, w2798, w2797) -> (w2796:errorcluster)
                n1295 = call <vilib>:"Clear Errors.vi"("error in (no error)"=w2796) -> ("error out"=w2793:errorcluster)  [unwired: 5 in, 1 out]
                n1296 = case shown="True" w2791 {
                  tunnel: w2793 -> [w2820 w2823]
                  tunnel: [w2820 w2821] -> w2792
                  frame False {
                  }
                  frame True {
                    n1297 = control-ref of="This VI"() -> (w2824:refnum<vi>)
                    n1298 = property class="VI"(reference=w2824, error in=w2823, "FP.State"=T18."Closed" ("Front Panel Window:State")) -> (error out=w2821:errorcluster)  [unwired: 1 out]
                  }
                }
              }
            }
          }
        }
      }
      frame "MainProgram" {
        n1299 = event shown="[5] \"Start\": Value Change" {
          selector: w2827 -> [_ _ _ _ _ _ _ _ _ _ _ _ _]
          dyn-events: _ -> [_ _ _ _ _ _ _ _ _ _ _ _ _]
          timeout: 50 -> [_ _ _ _ _ _ _ _ _ _ _ _ _]
          tunnel: [T12."MainProgram" T12."MainProgram" T12."MainProgram" T12."MainProgram" T12."MainProgram" T12."MainProgram" w3453 T12."MainProgram" T12."MainProgram" T12."MainProgram" T12."Stop" T12."MainProgram" T12."MainProgram"] -> w2848
          tunnel: [w2853 w2927 w3018 w3025 w3034 w3046 w3487 w3581 w3600 w3605 w3729 w3732 w3744] -> w2842
          tunnel: w2846 -> [w2858 w2952 w3017 w3027 w3034 w3064 w3489 w3588 w3599 w3609 w3729 w3732 w3747]
          tunnel: [w2867 w2931 w3019 w3026 w3035 w3058 w3485 w3586 w3597 w3613 w3726 w3738 w3746] -> w2843
          tunnel: w2844 -> [w2867 w2931 w3019 w3026 w3035 w3058 w3485 w3586 w3597 _ w3726 w3738 w3746]
          tunnel: w2841 -> [w2860 w2956 w3013 w3022 w3031 w3061 w3492 w3585 w3596 w3616 w3725 w3737 w3751]
          tunnel: w2840 -> [w2854 w2957 w3014 w3023 w3032 w3062 w3491 w3584 w3595 w3615 w3724 w3736 w3750]
          tunnel: [w2856 w2957 w3014 w3023 w3032 w3062 w3491 w3584 w3595 w3615 w3724 w3736 w3750] -> w2839
          tunnel: [w2859 w2956 w3013 w3022 w3031 w3061 w3492 w3585 w3596 w3616 w3725 w3737 w3751] -> w2838
          tunnel: w2837 -> [w2857 w2958 w3012 w3021 w3030 w3060 w3490 w3583 w3594 w3614 w3723 w3735 w3749]
          tunnel: [w2857 w2958 w3012 w3021 w3030 w3056 w3490 w3583 w3594 w3614 w3723 w3735 w3749] -> w2836
          tunnel: w2835 -> [_ _ _ _ _ _ _ _ _ _ _ _ _]
          tunnel: [w2851 _ _ _ _ w3055 _ _ _ _ _ _ _] -> w2831
          tunnel: w2832 -> [_ _ _ _ _ w3055 _ _ _ _ _ _ _]
          tunnel: w2829 -> [_ _ _ _ _ _ w3472 _ _ _ _ _ _]
          tunnel: w2829 -> [_ w2926 _ _ _ _ _ _ _ _ _ _ _]
          tunnel: w2828 -> [_ _ _ _ _ _ w3483 _ _ _ _ _ _]
          tunnel: w2826 -> [w2850 w2923 w3011 w3020 w3029 w3048 w3446 w3580 w3593 w3607 w3722 w3730 w3740]
          tunnel: [w2850 w2923 w3011 w3020 w3029 w3048 w3445 w3580 w3593 w3607 w3722 w3730 w3740] -> w2825
          event Timeout {
            n1300 = event-data() -> ()  [unwired: 1 in, 3 out]
            n1301 = property class="Clust (strict)"(reference=w2854, error in=w2858) -> (reference out=w2856:refnum<vi>, error out=w2855:errorcluster, "Value"=w2864:T9)
            n1302 = Unbundle By Name(w2864) -> ("DevType"=w2865:T4, "CanIndex"=w2862:T3)
            n1303 = call "VCI_Receive.vi"("CANIndex"=w2862, "DevIndex"=u32 0, "DevType"=w2865) -> ("Recieve"=w2861:T21[])  [unwired: 3 in, 5 out]
            n1304 = Empty Array?(array=w2861) -> (empty?=w2863:bool)
            n1305 = case shown="False" w2863 {
              tunnel: w2862 -> [w2887 _]
              tunnel: w2856 -> [w2885 _]
              tunnel: w2860 -> [w2884 w2920]
              tunnel: w2855 -> [w2883 w2919]
              tunnel: w2861 -> [w2888 _]
              tunnel: [w2878 w2919] -> w2853
              tunnel: [w2877 w2920] -> w2859
              tunnel: [w2876 0] -> _
              frame False {
                n1306 = call "Demo_MakeDispBuff.vi"("Channel"=w2887, "Type"=enum16{"接收", "发送"}."接收", "OBJs"=w2888) -> ("Buffer"=w2886:T22)
                n1307 = for {
                  N: 3 -> [_]
                  tunnel: w2886 -> [w2902]
                  tunnel: w2885 -> [w2901]
                  tunnel: w2884 -> [w2892]
                  tunnel: w2883 -> [w2891]
                  tunnel: [w2894] -> w2881 mode=indexing
                  tunnel: [w2892] -> w2880
                  tunnel: [w2891] -> w2879
                  tunnel: [w2890] -> w2876
                  i -> [w2890]
                  n1308 = property class="Clust (strict)"(reference=w2901) -> ("Value"=w2899:T9)  [unwired: 1 in, 2 out]
                  n1309 = Index Array(array=w2902, index=w2890) -> (element=w2895:T23)
                  n1310 = Unbundle By Name(w2895) -> ("Channel"=w2897:T3, "VCI_CAN_OBJ"=w2900:T21)  [unwired: 2 out]
                  n1311 = Unbundle By Name(w2899) -> ("CanIndex"=w2898:T3)
                  n1312 = Equal?(x=w2898, y=w2897) -> (x = y?=w2896:bool)
                  n1313 = case shown="True" w2896 {
                    tunnel: w2900 -> [_ w2913]
                    tunnel: [w2903 w2909] -> w2894
                    tunnel: T17 {"ID"=0, "MSGTYPE"=0, "LEN"=0, "aDATA"=[]} ("Msg") -> [w2903 w2908]
                    frame False {
                    }
                    frame True {
                      n1314 = Unbundle By Name(w2913) -> ("ID"=w2907:u32, "DataLen"=w2912:u8, "Data"=w2910:u8[])
                      n1315 = Bundle By Name(cluster=w2908, "ID"=w2907, "MSGTYPE"=u8 0, "LEN"=w2912, "aDATA"=w2910) -> (w2909:T17)
                      n1316 = Unbundle By Name(w2909) -> ("ID"=w2905:u32)
                      n1317 = Split Number(x=w2905) -> (lo(x)=w2906:u16)  [unwired: 1 out]
                      n1318 = Split Number(x=w2906) -> (lo(x)=w2904:u8)  [unwired: 1 out]
                      "UUT" <- w2904
                      n1319 = case shown="63" w2904 {
                        tunnel: ["EBAY 5F" "" "AHU 3F" "AHU 2F"] -> _
                        frame 95 {
                        }
                        frame Default {
                        }
                        frame 63 {
                        }
                        frame 47 {
                        }
                      }
                    }
                  }
                }
                n1320 = Enqueue Element(queue=w2880, element=w2881, error in (no error)=w2879) -> (queue out=w2877:refnum<queue>, error out=w2878:errorcluster)  [unwired: 2 out]
              }
              frame True {
              }
            }
            n1321 = property on="ClosePanel" class="Bool (strict)"() -> ("Value"=→"ClosePanel 2":bool)  [unwired: 2 in, 2 out]
            n1322 = First Call?() -> (First Call?: T/F=w2852:bool)
            n1323 = case shown="False" w2852 {
              tunnel: [w2872 "Main Program..."] -> w2851
              frame False {
                n1324 = property on="f" class="Enum (strict)"() -> ("Value"=w2871:T2)  [unwired: 2 in, 2 out]
                n1325 = Equal?(x=w2871, y=T2."Empty") -> (x = y?=w2869:bool)
                n1326 = property on="Pannel User Message" class="Str"() -> ("Value"=w2873:string)  [unwired: 2 in, 2 out]
                n1327 = Select(t="You can press \"Start\" button to perform test(s).", s=w2869, f=w2873) -> (s? t:f=w2872:string)
              }
              frame True {
              }
            }
          }
          event "SetSN": Value Change {
            w2921 = TRUE ("Report")
            n1328 = event-data() -> ()  [unwired: 1 in, 6 out]
            n1329 = property on="UUT" class="DigNum (strict)"() -> ("Value"=w2961:u8)  [unwired: 2 in, 2 out]
            n1330 = Equal?(x=w2961, y=u8 95) -> (x = y?=w2959:bool)
            n1331 = property on="ComTestind" class="Bool (strict)"() -> ("Value"=w2938:bool)  [unwired: 2 in, 2 out]
            n1332 = property on="VisualInspectionResult" class="Bool (strict)"() -> ("Value"=w2941:bool)  [unwired: 2 in, 2 out]
            n1333 = property on="Auxiind" class="Bool (strict)"() -> ("Value"=w2940:bool)  [unwired: 2 in, 2 out]
            n1334 = property on="TempSensCalind" class="Bool (strict)"() -> ("Value"=w2943:bool)  [unwired: 2 in, 2 out]
            n1335 = call <vilib>:"Clear Errors.vi"("error in (no error)"=w2952) -> ("error out"=w2950:errorcluster)  [unwired: 5 in, 1 out]
            n1336 = case shown="True" w2959 {
              tunnel: ["AHU Software Version" ("key") "EBAY Software Version" ("key")] -> _
              tunnel: ["AHU Serial Number" ("key") "EBAY Serial Number" ("key")] -> w2932
              tunnel: [TRUE ("Value") w3008] -> w2935
              frame False {
              }
              frame True {
                n1337 = property on="TempControlind" class="Bool (strict)"() -> ("Value"=w3008:bool)  [unwired: 2 in, 2 out]
              }
            }
            n1338 = VISA Flush I/O Buffer(VISA resource name=w2931, error in (no error)=w2950) -> (VISA resource name out=w2954:refnum<visa-resource-name>, error out=w2951:errorcluster)  [unwired: 1 in]
            n1339 = property on="MotorTempind" class="Bool (strict)"() -> ("Value"=w2936:bool)  [unwired: 2 in, 2 out]
            n1340 = property on="SpeedStopind" class="Bool (strict)"() -> ("Value"=w2937:bool)  [unwired: 2 in, 2 out]
            n1341 = property on="Burninind" class="Bool (strict)"() -> ("Value"=w2942:bool)  [unwired: 2 in, 2 out]
            n1342 = property on="EnableTestind" class="Bool (strict)"() -> ("Value"=w2939:bool)  [unwired: 2 in, 2 out]
            n1343 = call "SerialMarvinMod.vi"("error in (no error)"=w2951, "write buffer"="SN\r\n", "VISA resource name"=w2954) -> ("error out"=w2930:errorcluster, "read buffer"=w2949:string)  [unwired: 7 in]
            n1344 = Decimal String To Number(string=w2949) -> (number=w2948:i32)  [unwired: 2 in, 1 out]
            n1345 = Equal?(x=w2948, y=0) -> (x = y?=w2945:bool)
            n1346 = Equal?(x=w2948, y=-1) -> (x = y?=w2944:bool)
            n1347 = Build Array(w2943, w2942, w2941, w2940, w2939, w2938, w2937, w2936, w2935) -> (w2934:bool[])
            n1348 = Compound Arithmetic op=OR(w2945, w2944) -> (w2924:bool)
            n1349 = And Array Elements(Boolean array=w2934) -> (logical AND=w2933:bool)
            n1350 = And(x=w2924, y=w2933) -> (x .and. y?=w2925:bool)
            n1351 = case shown="True" w2925 {
              tunnel: w2932 -> [_ w2989]
              tunnel: w2931 -> [_ w2987]
              tunnel: w2930 -> [w2963 w2986]
              tunnel: [w2964 w2973] -> w2929
              tunnel: w2926 -> [_ w2970]
              tunnel: w2924 -> [w2962 _]
              frame False {
                n1352 = case shown="True" w2962 {
                  tunnel: [w2965 w2967] -> w2964
                  tunnel: w2963 -> [w2965 w2966]
                  frame False {
                  }
                  frame True {
                    n1353 = call "Display Message to User5"("error in (no error)"=w2966) -> ("error out"=w2967:errorcluster)  [unwired: 9 in, 1 out]
                  }
                }
              }
              frame True {
                n1354 = VISA Flush I/O Buffer(VISA resource name=w2987, error in (no error)=w2986) -> (VISA resource name out=w2981:refnum<visa-resource-name>, error out=w2988:errorcluster)  [unwired: 1 in]
                n1355 = property on="Next SN" class="Str"() -> ("Value"=w2969:string)  [unwired: 2 in, 2 out]
                n1356 = Decimal String To Number(string=w2969) -> (number=w2968:i32)  [unwired: 2 in, 1 out]
                n1357 = Number To Decimal String(number=w2968) -> (decimal integer string=w2976:string)  [unwired: 1 in]
                n1358 = Concatenate Strings("EP=1\r\nSN=" ("write buffer"), w2976, "\r\n" ("string")) -> (w2983:string)
                n1359 = call "SerialMarvinMod.vi"("error in (no error)"=w2988, "Clear Log"=FALSE, "write buffer"=w2983, "VISA resource name"=w2981) -> ("error out"=w2980:errorcluster)  [unwired: 6 in, 1 out]
                n1360 = VISA Flush I/O Buffer(VISA resource name=w2981, error in (no error)=w2980) -> (VISA resource name out=w2979:refnum<visa-resource-name>, error out=w2982:errorcluster)  [unwired: 1 in]
                n1361 = call "SerialMarvinMod.vi"("error in (no error)"=w2982, "Clear Log"=FALSE, "write buffer"="SN\r\n", "VISA resource name"=w2979) -> ("error out"=w2974:errorcluster, "read buffer"=w2977:string)  [unwired: 6 in]
                n1362 = Equal?(x=w2977, y=w2976) -> (x = y?=w2975:bool)
                n1363 = case shown="True" w2975 {
                  tunnel: w2989 -> [_ w3003]
                  tunnel: w2976 -> [_ w3002]
                  tunnel: w2974 -> [w2990 w2993]
                  tunnel: [w2990 w3000] -> w2973
                  tunnel: w2968 -> [_ w2998]
                  tunnel: w2970 -> [_ w2996]
                  frame False {
                  }
                  frame True {
                    n1364 = call <vilib>:"Open Config Data.vi"("error in (no error)"=w2993, "create file if necessary (T)"=FALSE, "configuration file path"=w2996) -> ("error out"=w2994:errorcluster, "refnum"=w2995:T15)  [unwired: 7 out]
                    n1365 = Increment(x=w2998) -> (x+1=w2992:i32)
                    n1366 = Number To Decimal String(number=w2992) -> (decimal integer string=w2991:string)  [unwired: 1 in]
                    n1367 = property on="Next SN" class="Str"("Value"=w2991) -> ()  [unwired: 2 in, 2 out]
                    n1368 = call-poly <vilib>:"Write Key.vi"("section"="Marvin", "error in (no error)"=w2994, "value"=w3002, "key"=w3003, "refnum"=w2995) -> ("error out"=w3001:errorcluster, "refnum out"=w2999:T15)  [unwired: 4 in, 1 out]
                    n1369 = call <vilib>:"Close Config Data.vi"("error in (no error)"=w3001, "refnum"=w2999) -> ("error out"=w3000:errorcluster)  [unwired: 8 in, 1 out]
                  }
                }
              }
            }
            n1370 = call <vilib>:"Clear Errors.vi"("error in (no error)"=w2929) -> ("error out"=w2927:errorcluster)  [unwired: 5 in, 1 out]
            n1371 = property on="SetSN" class="Bool (strict)"(error in=w2927, "Value"=FALSE ("SetSN")) -> (error out=w2922:errorcluster)  [unwired: 1 in, 1 out]
            n1372 = property on="Report" class="Bool (strict)"(error in=w2922, "Value"=w2921, "Val(Sgnl)"=w2921) -> ()  [unwired: 1 in, 2 out]
          }
          event "ATR", "Pannel User Message": Mouse Enter {
            n1373 = event-data() -> ()  [unwired: 1 in, 4 out]
            n1374 = call-poly <vilib>:"Set Cursor.vi"("error in (no error)"=w3017, "icon"=u16 1) -> ("error out"=w3018:errorcluster)  [unwired: 8 in, 1 out]
          }
          event "ATR", "Pannel User Message": Mouse Leave {
            n1375 = event-data() -> ()  [unwired: 1 in, 4 out]
            n1376 = call-poly <vilib>:"Set Cursor.vi"("error in (no error)"=w3027, "icon"=u16 0) -> ("error out"=w3025:errorcluster)  [unwired: 8 in, 1 out]
          }
          event "ATR": Mouse Down? {
            n1377 = event-data() -> ("Coords"=w3042:T24)  [unwired: 1 in, 4 out]
            n1378 = invoke on="ATR" class="Tbl (strict)" method="Point To Row Column"("Point"=w3042) -> ("InBounds"=w3038:bool, "CellPosition"=w3037:T16)  [unwired: 5 in, 4 out]
            n1379 = Greater Than 0?(x=w3037) -> (x > 0?=w3041:cluster{"Row":bool, "Column":bool})
            n1380 = Cluster To Array(cluster=w3041) -> (array=w3040:bool[])
            n1381 = Or Array Elements(Boolean array=w3040) -> (logical OR=w3039:bool)
            n1382 = Compound Arithmetic op=OR(w3038, w3039) -> (w3036:bool)
            n1383 = event-data("Discard?"=w3036) -> ()  [unwired: 1 in, 1 out]
          }
          event "Start": Value Change {
            w3044 = FALSE ("Stop Button")
            (unwired) T19."Start"
            n1384 = event-data() -> ()  [unwired: 1 in, 2 out]
            n1385 = call <vilib>:"Clear Errors.vi"("error in (no error)"=w3064) -> ("error out"=w3050:errorcluster)  [unwired: 5 in, 1 out]
            n1386 = property on="UUT" class="Str"(error in=w3050) -> (error out=w3049:errorcluster, "Value"=w3063:string)  [unwired: 1 in, 1 out]
            n1387 = property on="ClosePanel" class="Bool (strict)"("Value"=w3044) -> ()  [unwired: 2 in, 2 out]
            n1388 = property on="Stop Button" class="Bool (strict)"("Value"=w3044) -> ()  [unwired: 2 in, 2 out]
            n1389 = while {
              tunnel: w3063 -> [w3072]
              tunnel: [w3071] -> w3057
              tunnel: [w3070] -> w3051
              tunnel: w3049 -> [w3068]
              shift-right: [w3067] -> _
              shift-left: T19."Verify VR" -> [w3069]
              stop <- w3066 stop-if-true
              n1390 = case shown="\"Verify UUT\"" w3069 {
                tunnel: w3072 -> [_ w3088 w3207 w3233]
                tunnel: [w3077 w3087 w3201 w3252] -> w3071
                tunnel: [w3079 w3086 w3208 w3274] -> w3070
                tunnel: w3068 -> [w3076 _ w3205 w3269]
                tunnel: [T19."End" T19."Start" w3209 w3246] -> w3067
                tunnel: [w3078 TRUE w3202 w3240] -> w3066
                frame "End", Default {
                  w3079 = T1 [] items=["Auxiliary", "Temp Sens Cal", "Com Test", "Enable Test", "Speed Command", "Stop Time", "Temp Control", "Burn in", "Visual Inspec", "Empty"]
                  n1391 = call "Display Message to User10"("error in (no error)"=w3076) -> ("error out"=w3073:errorcluster)  [unwired: 9 in, 1 out]
                  n1392 = property on="Refresh Button" class="Bool (strict)"(error in=w3073, "Val(Sgnl)"=TRUE ("Value (Signaling)")) -> (error out=w3074:errorcluster)  [unwired: 1 in, 1 out]
                  n1393 = flat-sequence {
                    tunnel: w3074 -> [w3081]
                    tunnel: [TRUE] -> w3078
                    tunnel: [w3081] -> w3077
                    frame #0 {
                    }
                  }
                }
                frame "Start" {
                  n1394 = case shown="\"EBAY\"" w3088 {
                    tunnel: [w3101 w3152] -> w3086
                    tunnel: [w3100 w3151] -> w3087
                    tunnel: [w3089 w3139] -> w3083
                    frame "AHU", Default {
                      n1395 = call "Load Program Process AHU.vi"() -> ("Speed Command Test"=w3094:bool, "Enable Test"=w3095:bool, "Burn-in Test"=w3092:bool, "Auxiliary"=w3090:bool, "Temperature Sensor Calibration Test"=w3097:bool, "Communication Test"=w3096:bool, "Motor Temperature Test"=w3093:bool, "Visual Inspection"=w3091:bool, "OK"=w3098:bool, "Automation"=w3089:bool, "error out"=w3100:errorcluster)  [unwired: 8 in, 9 out]
                      n1396 = Compound Arithmetic op=OR(w3098, w3089) -> (w3099:bool)
                      n1397 = case shown="True" w3099 {
                        tunnel: [w3102 w3112] -> w3101
                        tunnel: w3089 -> [_ w3111]
                        tunnel: w3097 -> [_ w3110]
                        tunnel: w3096 -> [_ w3109]
                        tunnel: w3095 -> [_ w3108]
                        tunnel: w3094 -> [_ w3107]
                        tunnel: w3093 -> [_ w3106]
                        tunnel: w3092 -> [_ w3105]
                        tunnel: w3091 -> [_ w3104]
                        tunnel: w3090 -> [_ w3103]
                        frame False {
                          w3102 = T1 [] items=["Auxiliary", "Temp Sens Cal", "Com Test", "Enable Test", "Speed Command", "Stop Time", "Temp Control", "Burn in", "Visual Inspec", "Empty"]
                        }
                        frame True {
                          n1398 = case shown="False" w3111 {
                            tunnel: [w3137 w3138] -> w3112
                            tunnel: w3110 -> [w3129 _]
                            tunnel: w3109 -> [w3128 _]
                            tunnel: w3108 -> [w3127 _]
                            tunnel: w3107 -> [w3126 _]
                            tunnel: w3106 -> [w3125 _]
                            tunnel: w3105 -> [w3124 _]
                            tunnel: w3104 -> [w3123 _]
                            tunnel: w3103 -> [w3122 _]
                            frame False {
                              w3120 = T2."Empty" ("f")
                              n1399 = Select(t=T2."Temp Sens Cal" ("f"), s=w3129, f=w3120) -> (s? t:f=w3114:T2)
                              n1400 = Select(t=T2."Com Test" ("f"), s=w3128, f=w3120) -> (s? t:f=w3113:T2)
                              n1401 = Select(t=T2."Enable Test" ("f"), s=w3127, f=w3120) -> (s? t:f=w3116:T2)
                              n1402 = Select(t=T2."Speed Command" ("f"), s=w3126, f=w3120) -> (s? t:f=w3117:T2)
                              n1403 = Select(t=T2."Stop Time" ("f"), s=w3125, f=w3120) -> (s? t:f=w3115:T2)
                              n1404 = Select(t=T2."Burn in" ("f"), s=w3124, f=w3120) -> (s? t:f=w3118:T2)
                              n1405 = Select(t=T2."Auxiliary" ("f"), s=w3122, f=w3120) -> ()  [unwired: 1 out]
                              n1406 = Select(t=T2."Visual Inspec" ("f"), s=w3123, f=w3120) -> (s? t:f=w3119:T2)
                              n1407 = Build Array(w3113, w3114, w3115, w3116, w3117, w3118, w3119) -> (w3137:T1)
                            }
                            frame True {
                              w3138 = T1 [enum."Com Test", enum."Temp Sens Cal", enum."Stop Time", enum."Enable Test", enum."Speed Command", enum."Burn in", enum."Visual Inspec"] items=["Auxiliary", "Temp Sens Cal", "Com Test", "Enable Test", "Speed Command", "Stop Time", "Temp Control", "Burn in", "Visual Inspec", "Empty"]
                            }
                          }
                        }
                      }
                    }
                    frame "EBAY" {
                      n1408 = call "Load Program Process EBAY.vi"() -> ("Speed Command Test"=w3145:bool, "Enable Test"=w3146:bool, "Burn-in Test"=w3143:bool, "Temperature Control Algorithm Test"=w3142:bool, "Auxiliary"=w3140:bool, "Temperature Sensor Calibration Test"=w3148:bool, "Communication Test"=w3147:bool, "Motor Temperature Test"=w3144:bool, "Visual Inspection"=w3141:bool, "OK"=w3149:bool, "Automation"=w3139:bool, "error out"=w3151:errorcluster)  [unwired: 8 in, 8 out]
                      n1409 = Compound Arithmetic op=OR(w3149, w3139) -> (w3150:bool)
                      n1410 = case shown="True" w3150 {
                        tunnel: [w3153 w3164] -> w3152
                        tunnel: w3139 -> [_ w3163]
                        tunnel: w3148 -> [_ w3162]
                        tunnel: w3147 -> [_ w3161]
                        tunnel: w3146 -> [_ w3160]
                        tunnel: w3145 -> [_ w3159]
                        tunnel: w3144 -> [_ w3158]
                        tunnel: w3143 -> [_ w3157]
                        tunnel: w3142 -> [_ w3156]
                        tunnel: w3141 -> [_ w3155]
                        tunnel: w3140 -> [_ w3154]
                        frame False {
                          w3153 = T1 [] items=["Auxiliary", "Temp Sens Cal", "Com Test", "Enable Test", "Speed Command", "Stop Time", "Temp Control", "Burn in", "Visual Inspec", "Empty"]
                        }
                        frame True {
                          n1411 = case shown="False" w3163 {
                            tunnel: [w3193 w3194] -> w3164
                            tunnel: w3162 -> [w3184 _]
                            tunnel: w3161 -> [w3183 _]
                            tunnel: w3160 -> [w3182 _]
                            tunnel: w3159 -> [w3181 _]
                            tunnel: w3158 -> [w3171 _]
                            tunnel: w3157 -> [w3176 _]
                            tunnel: w3156 -> [w3175 _]
                            tunnel: w3155 -> [w3180 _]
                            tunnel: w3154 -> [w3179 _]
                            frame False {
                              w3177 = T2."Empty" ("f")
                              n1412 = Select(t=T2."Temp Sens Cal" ("f"), s=w3184, f=w3177) -> (s? t:f=w3166:T2)
                              n1413 = Select(t=T2."Com Test" ("f"), s=w3183, f=w3177) -> (s? t:f=w3165:T2)
                              n1414 = Select(t=T2."Enable Test" ("f"), s=w3182, f=w3177) -> (s? t:f=w3168:T2)
                              n1415 = Select(t=T2."Speed Command" ("f"), s=w3181, f=w3177) -> (s? t:f=w3169:T2)
                              n1416 = Select(t=T2."Stop Time" ("f"), s=w3171, f=w3177) -> (s? t:f=w3167:T2)
                              n1417 = Select(t=T2."Temp Control" ("f"), s=w3175, f=w3177) -> (s? t:f=w3170:T2)
                              n1418 = Select(t=T2."Burn in" ("f"), s=w3176, f=w3177) -> (s? t:f=w3172:T2)
                              n1419 = Select(t=T2."Visual Inspec" ("f"), s=w3180, f=w3177) -> (s? t:f=w3174:T2)
                              n1420 = Select(t=T2."Auxiliary" ("f"), s=w3179, f=w3177) -> (s? t:f=w3173:T2)
                              n1421 = Build Array(w3165, w3166, w3167, w3168, w3169, w3170, w3172, w3173, w3174) -> (w3193:T1)
                            }
                            frame True {
                              w3194 = T1 [enum."Com Test", enum."Temp Sens Cal", enum."Stop Time", enum."Enable Test", enum."Speed Command", enum."Temp Control", enum."Burn in", enum."Auxiliary", enum."Visual Inspec"] items=["Auxiliary", "Temp Sens Cal", "Com Test", "Enable Test", "Speed Command", "Stop Time", "Temp Control", "Burn in", "Visual Inspec", "Empty"]
                              # "Temp control - empty"
                            }
                          }
                        }
                      }
                    }
                  }
                  "Automation" <- w3083
                }
                frame "Verify VR" {
                  w3208 = T1 [] items=["Auxiliary", "Temp Sens Cal", "Com Test", "Enable Test", "Speed Command", "Stop Time", "Temp Control", "Burn in", "Visual Inspec", "Empty"]
                  n1422 = control-ref of="Stop Button"() -> (w3197:refnum<vi>)
                  n1423 = property on="Serial" class="Bool (strict)"(error in=w3205) -> (error out=w3204:errorcluster, "Value"=w3203:bool)  [unwired: 1 in, 1 out]
                  n1424 = control-ref of="Pannel User Message"() -> (w3198:refnum<vi>)
                  n1425 = case shown="True" w3203 {
                    tunnel: w3204 -> [w3213 w3223]
                    tunnel: [T19."Verify VR" w3217] -> w3209
                    tunnel: w3207 -> [_ w3222]
                    tunnel: [w3211 w3216] -> w3206
                    tunnel: [TRUE FALSE] -> w3202
                    frame False {
                      n1426 = call "Display Message to User9"("error in (no error)"=w3213) -> ("error out"=w3211:errorcluster)  [unwired: 9 in, 1 out]
                    }
                    frame True {
                      n1427 = property on="VISA resource name" class="VISAName"() -> ("Value"=w3225:refnum<visa-resource-name>)  [unwired: 2 in, 2 out]
                      n1428 = case shown="\"EBAY\"" w3222 {
                        tunnel: ["5.3.8d" ("write buffer") "5.3.9" ("write buffer")] -> w3220
                        frame "AHU", Default {
                        }
                        frame "EBAY" {
                        }
                      }
                      n1429 = VISA Flush I/O Buffer(VISA resource name=w3225, error in (no error)=w3223) -> (VISA resource name out=w3227:refnum<visa-resource-name>, error out=w3226:errorcluster)  [unwired: 1 in]
                      n1430 = call "SerialMarvinMod.vi"("error in (no error)"=w3226, "write buffer"="VR\r\n", "VISA resource name"=w3227) -> ("error out"=w3216:errorcluster, "read buffer"=w3221:string)  [unwired: 7 in]
                      n1431 = Equal?(x=w3221, y=w3220) -> (x = y?=w3215:bool)
                      n1432 = Select(t=T19."Verify UUT", s=w3215, f=T19."End") -> (s? t:f=w3217:T19)
                    }
                  }
                  n1433 = control-ref of="Motor Speed RPM"() -> (w3195:refnum<vi>)
                  n1434 = call "Write panel message (SubVI).vi"("rpm"=w3195, "PrintTime"=FALSE, "Stop"=w3197, "error in (no error)"=w3206, "Time to wait"=0.1, "Strin"="TESTER BIT TEST OPERATION IN PROCESS", "String in"=w3198) -> ("error out"=w3201:errorcluster)  [unwired: 4 in]
                }
                frame "Verify UUT" {
                  w3255 = FALSE ("Clear Log")
                  w3274 = T1 [] items=["Auxiliary", "Temp Sens Cal", "Com Test", "Enable Test", "Speed Command", "Stop Time", "Temp Control", "Burn in", "Visual Inspec", "Empty"]
                  # "25 C"
                  n1435 = property on="VISA resource name" class="VISAName"() -> ("Value"=w3271:refnum<visa-resource-name>)  [unwired: 2 in, 2 out]
                  n1436 = Equal?(x=w3233, y="EBAY") -> (x = y?=w3231:bool)
                  n1437 = VISA Flush I/O Buffer(VISA resource name=w3271, error in (no error)=w3269) -> (VISA resource name out=w3273:refnum<visa-resource-name>, error out=w3272:errorcluster)  [unwired: 1 in]
                  n1438 = control-ref of="VISA resource name out"() -> (w3266:refnum<vi>)
                  n1439 = call "SerialMarvinMod.vi"("error in (no error)"=w3272, "Clear Log"=w3255, "write buffer"="TA[1]\r\n", "VISA resource name"=w3273) -> ("error out"=w3257:errorcluster, "read buffer"=w3251:string)  [unwired: 6 in]
                  n1440 = case shown="True" w3231 {
                    tunnel: [w3317 w3321] -> w3234
                    tunnel: [i32[] [2] i32[] [1, 2]] -> w3230
                    frame False {
                      # "Cur"
                      n1441 = Byte Array To String(unsigned byte array=u8[] [75, 0, 4, 17, 0, 0, 0, 0] ("appended array")) -> (string=w3318:string)
                      n1442 = Build Array(w3318) -> (w3317:string[])
                    }
                    frame True {
                      # "Cur"
                      # "EBAYFAN"
                      n1443 = Byte Array To String(unsigned byte array=u8[] [75, 0, 4, 18, 0, 0, 0, 0] ("appended array")) -> (string=w3322:string)
                      n1444 = Byte Array To String(unsigned byte array=u8[] [75, 0, 4, 17, 0, 0, 0, 0] ("appended array")) -> (string=w3323:string)
                      n1445 = Build Array(w3322, w3323) -> (w3321:string[])
                    }
                  }
                  n1446 = property class="VISAName"(reference=w3266, error in=w3257) -> (error out=w3267:errorcluster, "Value"=w3268:refnum<visa-resource-name>)  [unwired: 1 out]
                  n1447 = Byte Array To String(unsigned byte array=u8[] [75, 0, 4, 2, 8, 0, 0, 0] ("appended array")) -> (string=w3264:string)
                  n1448 = property on="VISA resource name" class="VISAName"() -> ("Value"=w3262:refnum<visa-resource-name>)  [unwired: 2 in, 2 out]
                  n1449 = VISA Write(VISA resource name=w3268, write buffer=w3264, error in (no error)=w3267) -> (error out=w3259:errorcluster)  [unwired: 2 out]
                  n1450 = call <vilib>:"Clear Errors.vi"("error in (no error)"=w3259) -> ("error out"=w3258:errorcluster)  [unwired: 5 in, 1 out]
                  n1451 = call "Time Delay10"("error in (no error)"=w3258) -> ("error out"=w3236:errorcluster)  [unwired: 10 in]
                  n1452 = VISA Flush I/O Buffer(VISA resource name=w3262, error in (no error)=w3236) -> (VISA resource name out=w3260:refnum<visa-resource-name>, error out=w3261:errorcluster)  [unwired: 1 in]
                  n1453 = call "SerialMarvinMod.vi"("error in (no error)"=w3261, "Clear Log"=w3255, "write buffer"="TA[2]\r\n", "VISA resource name"=w3260) -> ("error out"=w3256:errorcluster, "read buffer"=w3250:string)  [unwired: 6 in]
                  n1454 = call "Time Delay9"("error in (no error)"=w3256) -> ("error out"=w3237:errorcluster)  [unwired: 10 in]
                  n1455 = case shown="True" w3231 {
                    tunnel: w3255 -> [_ w3304]
                    tunnel: [w3298 w3303] -> w3254
                    tunnel: ["" ("read buffer") w3302] -> w3249
                    tunnel: w3237 -> [w3298 w3301]
                    frame False {
                    }
                    frame True {
                      # "K17"
                      n1456 = control-ref of="VISA resource name out"() -> (w3313:refnum<vi>)
                      n1457 = property class="VISAName"(reference=w3313, error in=w3301) -> (error out=w3312:errorcluster, "Value"=w3311:refnum<visa-resource-name>)  [unwired: 1 out]
                      n1458 = Byte Array To String(unsigned byte array=u8[] [75, 0, 4, 2, 0, 0, 1, 0] ("appended array")) -> (string=w3315:string)
                      n1459 = VISA Write(VISA resource name=w3311, write buffer=w3315, error in (no error)=w3312) -> (error out=w3306:errorcluster)  [unwired: 2 out]
                      n1460 = property on="VISA resource name" class="VISAName"() -> ("Value"=w3308:refnum<visa-resource-name>)  [unwired: 2 in, 2 out]
                      n1461 = call <vilib>:"Clear Errors.vi"("error in (no error)"=w3306) -> ("error out"=w3305:errorcluster)  [unwired: 5 in, 1 out]
                      n1462 = call "Time Delay11"("error in (no error)"=w3305) -> ("error out"=w3300:errorcluster)  [unwired: 10 in]
                      n1463 = VISA Flush I/O Buffer(VISA resource name=w3308, error in (no error)=w3300) -> (VISA resource name out=w3310:refnum<visa-resource-name>, error out=w3309:errorcluster)  [unwired: 1 in]
                      n1464 = call "SerialMarvinMod.vi"("error in (no error)"=w3309, "Clear Log"=w3304, "write buffer"="TA[3]\r\n", "VISA resource name"=w3310) -> ("error out"=w3303:errorcluster, "read buffer"=w3302:string)  [unwired: 6 in]
                    }
                  }
                  n1465 = for {
                    tunnel: [w3329] -> w3248 mode=indexing
                    tunnel: w3234 -> [w3327] mode=indexing
                    tunnel: w3254 -> [w3336]
                    tunnel: [w3330] -> w3253
                    tunnel: w3230 -> [w3326] mode=indexing
                    n1466 = call <vilib>:"Clear Errors.vi"("error in (no error)"=w3332) -> ("error out"=w3334:errorcluster)  [unwired: 5 in, 1 out]
                    n1467 = control-ref of="VISA resource name out"() -> (w3337:refnum<vi>)
                    n1468 = property class="VISAName"(reference=w3337, error in=w3336) -> (error out=w3338:errorcluster, "Value"=w3339:refnum<visa-resource-name>)  [unwired: 1 out]
                    n1469 = VISA Write(VISA resource name=w3339, write buffer=w3327, error in (no error)=w3338) -> (VISA resource name out=w3335:refnum<visa-resource-name>, error out=w3333:errorcluster)  [unwired: 1 out]
                    n1470 = while {
                      tunnel: w3334 -> [w3354]
                      tunnel: [w3353] -> _
                      tunnel: w3331 -> [w3351]
                      tunnel: [w3346] -> _
                      tunnel: w3335 -> [w3345]
                      tunnel: [w3344] -> w3330
                      tunnel: [w3343] -> w3329
                      tunnel: w3326 -> [w3342]
                      stop <- w3347 stop-if-true
                      n1471 = VISA Read(VISA resource name=w3345, byte count=u32 1, error in (no error)=w3354) -> (VISA resource name out=w3356:refnum<visa-resource-name>, read buffer=w3357:string, error out=w3355:errorcluster)  [unwired: 1 out]
                      n1472 = String To Byte Array(string=w3357) -> (unsigned byte array=w3360:u8[])
                      n1473 = call <vilib>:"High Resolution Relative Seconds.vi"() -> ("relative seconds"=w3352:dbl)
                      n1474 = Index Array(array=w3360, index=0) -> (element=w3358:u8)
                      n1475 = Subtract(x=w3352, y=w3351) -> (x-y=w3350:dbl)
                      n1476 = case shown="75" w3358 {
                        tunnel: [w3365 w3370] -> w3344
                        tunnel: w3356 -> [w3364 w3379]
                        tunnel: w3355 -> [w3365 w3378]
                        tunnel: [w3364 w3371] -> w3353
                        tunnel: [u32 9999 w3368] -> w3346
                        tunnel: [FALSE w3367] -> w3343
                        tunnel: w3342 -> [_ w3366]
                        frame 0, Default {
                        }
                        frame 75 {
                          n1477 = VISA Read(VISA resource name=w3379, byte count=u32 3, error in (no error)=w3378) -> (VISA resource name out=w3374:refnum<visa-resource-name>, read buffer=w3382:string, error out=w3373:errorcluster)  [unwired: 1 out]
                          n1478 = String To Byte Array(string=w3382) -> (unsigned byte array=w3372:u8[])
                          n1479 = Index Array(array=w3372, index #1=0 ("index")) -> (element #1=w3377:u8, element #2=w3375:u8)  [unwired: 2 in, 1 out]
                          n1480 = Equal?(x=u8 0, y=w3377) -> (x = y?=w3376:bool)
                          n1481 = case shown="True" w3376 {
                            tunnel: [w3385 w3393] -> w3370
                            tunnel: w3375 -> [_ w3400]
                            tunnel: w3374 -> [w3386 w3399]
                            tunnel: w3373 -> [w3385 w3398]
                            tunnel: w3372 -> [_ w3397]
                            tunnel: [w3386 w3395] -> w3371
                            tunnel: [u32 9999 w3389] -> w3368
                            tunnel: [FALSE w3388] -> w3367
                            tunnel: w3366 -> [_ w3387]
                            frame False {
                            }
                            frame True {
                              n1482 = VISA Read(VISA resource name=w3399, byte count=w3400, error in (no error)=w3398) -> (VISA resource name out=w3395:refnum<visa-resource-name>, read buffer=w3394:string, error out=w3393:errorcluster)  [unwired: 1 out]
                              n1483 = String To Byte Array(string=w3394) -> (unsigned byte array=w3396:u8[])
                              n1484 = Insert Into Array(array=w3397, new element=w3396) -> (w3390:u8[])  [unwired: 1 in]
                              n1485 = Index Array(array=w3390, index #1=0 ("index")) -> (element #3=w3391:u8)  [unwired: 2 in, 2 out]
                              n1486 = case shown="15..19" w3391 {
                                tunnel: w3390 -> [_ w3412]
                                tunnel: [u32 9999 w3404] -> w3389
                                tunnel: [FALSE w3405] -> w3388
                                tunnel: w3387 -> [_ w3403]
                                frame 0, Default {
                                }
                                frame 15..19 {
                                n1487 = Index Array(array=w3412, index #1=3 ("index")) -> (element #1=w3411:u8, element #2=w3410:u8, element #3=w3409:u8, element #4=w3408:u8)  [unwired: 3 in]
                                n1488 = Join Numbers(hi=w3410, lo=w3411) -> ((hi.lo)=w3407:u16)
                                n1489 = Join Numbers(hi=w3408, lo=w3409) -> ((hi.lo)=w3406:u16)
                                n1490 = Join Numbers(hi=w3406, lo=w3407) -> ((hi.lo)=w3404:u32)
                                n1491 = case shown="1" w3403 {
                                tunnel: [w3414 w3418] -> w3405
                                tunnel: w3404 -> [w3416 w3417]
                                frame 2, Default {
                                n1492 = Less Or Equal?(x=w3416, y=u32 50) -> (x <= y?=w3414:bool)
                                }
                                frame 1 {
                                n1493 = Greater Or Equal?(x=w3417, y=2200.0) -> (x >= y?=w3418:bool)
                                }
                                }
                                }
                              }
                            }
                          }
                        }
                      }
                      n1494 = Greater Or Equal?(x=w3350, y=5.0) -> (x >= y?=w3348:bool)
                      n1495 = Compound Arithmetic op=OR(w3348, w3343) -> (w3347:bool)
                    }
                    n1496 = call "Time Delay12"("error in (no error)"=w3333) -> ("error out"=w3328:errorcluster)  [unwired: 10 in]
                    n1497 = flat-sequence {
                      tunnel: w3328 -> [w3341]
                      tunnel: [w3341] -> w3332
                      tunnel: [w3340] -> w3331
                      frame #0 {
                        n1498 = call <vilib>:"High Resolution Relative Seconds.vi"() -> ("relative seconds"=w3340:dbl)
                      }
                    }
                  }
                  n1499 = call <vilib>:"Clear Errors.vi"("error in (no error)"=w3253) -> ("error out"=w3252:errorcluster)  [unwired: 5 in, 1 out]
                  n1500 = case shown="False" w3231 {
                    tunnel: w3251 -> [w3284 w3297]
                    tunnel: w3250 -> [w3283 w3296]
                    tunnel: w3249 -> [_ w3295]
                    tunnel: w3248 -> [w3277 w3287]
                    tunnel: [w3276 w3286] -> w3244
                    tunnel: [string[] ["TA[1] OPERATION FAILED!", "TA[2] OPERATION FAILED!", "CURRENT OPERATION FAILED!"] string[] ["TA[1] OPERATION FAILED!", "TA[2] OPERATION FAILED!", "TA[3] OPERATION FAILED!", "EBAY FAN OPERATION FAILED!", "CURRENT OPERATION FAILED!"]] -> w3243
                    frame False {
                      w3280 = 100.0 ("y")
                      n1501 = Fract/Exp String To Number(string=w3284) -> (number=w3282:dbl)  [unwired: 3 in, 1 out]
                      n1502 = Fract/Exp String To Number(string=w3283) -> (number=w3281:dbl)  [unwired: 3 in, 1 out]
                      n1503 = Less Or Equal?(x=w3282, y=w3280) -> (x <= y?=w3279:bool)
                      n1504 = Less Or Equal?(x=w3281, y=w3280) -> (x <= y?=w3278:bool)
                      n1505 = Build Array (concatenate)(w3279, w3278, w3277) -> (w3276:bool[])
                    }
                    frame True {
                      w3291 = 100.0 ("y")
                      n1506 = Fract/Exp String To Number(string=w3297) -> (number=w3294:dbl)  [unwired: 3 in, 1 out]
                      n1507 = Fract/Exp String To Number(string=w3296) -> (number=w3293:dbl)  [unwired: 3 in, 1 out]
                      n1508 = Fract/Exp String To Number(string=w3295) -> (number=w3292:dbl)  [unwired: 3 in, 1 out]
                      n1509 = Less Or Equal?(x=w3294, y=w3291) -> (x <= y?=w3290:bool)
                      n1510 = Less Or Equal?(x=w3293, y=w3291) -> (x <= y?=w3289:bool)
                      n1511 = Less Or Equal?(x=w3292, y=w3291) -> (x <= y?=w3288:bool)
                      n1512 = Build Array (concatenate)(w3290, w3289, w3288, w3287) -> (w3286:bool[])
                    }
                  }
                  n1513 = for {
                    tunnel: w3244 -> [w3426] mode=indexing
                    tunnel: w3243 -> [w3425] mode=indexing
                    shift-right: [w3423] -> w3241
                    shift-left: "" -> [w3424]
                    n1514 = case shown="False" w3426 {
                      tunnel: w3425 -> [w3429 _]
                      tunnel: w3424 -> [w3430 w3431]
                      tunnel: [w3427 w3431] -> w3423
                      frame False {
                        n1515 = Concatenate Strings(w3430, w3429, "\r\n") -> (w3427:string)
                      }
                      frame True {
                      }
                    }
                  }
                  n1516 = And Array Elements(Boolean array=w3244) -> (logical AND=w3235:bool)
                  n1517 = Not(x=w3235) -> (.not. x?=w3238:bool)
                  n1518 = Select(t=T19."Start", s=w3235, f=T19."End") -> (s? t:f=w3246:T19)
                  n1519 = case shown="True" w3235 {
                    tunnel: w3241 -> [w3421 _]
                    tunnel: [w3420 FALSE ("true")] -> w3239
                    frame False {
                      n1520 = One Button Dialog(message=w3421) -> (true=w3420:bool)  [unwired: 1 in]
                    }
                    frame True {
                    }
                  }
                  n1521 = And(x=w3239, y=w3238) -> (x .and. y?=w3240:bool)
                }
              }
            }
            n1522 = Bundle By Name(cluster=T10 {"VISA"="COM1", "Array Test"=[]}, "VISA"=w3058, "Array Test"=w3051) -> (w3053:T10)
            n1523 = property on="Serial" class="Bool (strict)"() -> ("Value"=w3054:bool)  [unwired: 2 in, 2 out]
            n1524 = case shown="False" w3054 {
              tunnel: w3051 -> [w3432 _]
              tunnel: w3053 -> [w3434 w3444]
              tunnel: [w3433 w3444] -> w3052
              frame False {
                n1525 = for {
                  tunnel: w3432 -> [w3443] mode=indexing
                  tunnel: [w3438] -> w3435
                  stop <- w3438 stop-if-true
                  n1526 = Equal?(x=w3443, y=T2."Temp Sens Cal") -> (x = y?=w3440:bool)
                  n1527 = Equal?(x=w3443, y=T2."Enable Test") -> (x = y?=w3439:bool)
                  n1528 = Or(x=w3440, y=w3439) -> (x .or. y?=w3438:bool)
                }
                n1529 = case shown="True" w3435 {
                  tunnel: w3434 -> [w3436 _]
                  tunnel: [w3436 T10 {"VISA"="COM1", "Array Test"=[]}] -> w3433
                  frame False {
                  }
                  frame True {
                    n1530 = call "Display Message to User8"() -> ()  [unwired: 10 in, 2 out]
                  }
                }
              }
              frame True {
              }
            }
            n1531 = Enqueue Element(queue=w3060, element=w3052, error in (no error)=w3057) -> (queue out=w3056:refnum<queue>, error out=w3047:errorcluster)  [unwired: 2 out]
            n1532 = property on="Start" class="Bool (strict)"(error in=w3047, "Value"=FALSE ("Start")) -> (error out=w3046:errorcluster)  [unwired: 1 in, 1 out]
          }
          event "Report", "Stop Button": Value Change {
            w3466 = "Marvin" ("section")
            w3478 = "_"
            # "EBAY 414-8005\nAHU-L (47) P/N 413-8005-1\nAHU-R (63) P/N 413-8005-2"
            n1533 = event-data() -> ("CtlRef"=w3458:refnum<vi>)  [unwired: 1 in, 5 out]
            n1534 = call <vilib>:"Application Directory.vi"() -> ("Application Directory"=w3500:path)
            n1535 = Build Path(base path=w3500, name or relative path="Reports") -> (appended path=w3503:path)
            n1536 = property on="Serial" class="Bool (strict)"() -> ("Value"=w3463:bool)  [unwired: 2 in, 2 out]
            n1537 = call <vilib>:"Open Config Data.vi"("create file if necessary (T)"=FALSE, "configuration file path"=w3472) -> ("refnum"=w3474:T15)  [unwired: 1 in, 8 out]
            n1538 = Get Date/Time String(want seconds? (F)=TRUE) -> (date string=w3505:string)  [unwired: 2 in, 1 out]
            n1539 = Search and Replace String(replace all?=TRUE ("replace all? (F)"), input string=w3505, search string="/") -> (result string=w3477:string)  [unwired: 5 in, 3 out]
            n1540 = property on="Report" class="Bool (strict)"("Value"=FALSE ("Report")) -> ()  [unwired: 2 in, 2 out]
            n1541 = local read "UUT"() -> (w3462:string)
            n1542 = case shown="\"EBAY\", Default" w3462 {
              tunnel: ["REV EBAY" ("key") "REV AHU" ("key")] -> w3461
              frame "EBAY", Default {
              }
              frame "AHU" {
              }
            }
            n1543 = call-poly <vilib>:"Read Key.vi"("section"=w3466, "key"=w3461, "refnum"=w3474) -> ("error out"=w3468:errorcluster, "value"=w3471:string, "refnum out"=w3470:T15)  [unwired: 5 in, 1 out]
            n1544 = call-poly <vilib>:"Read Key.vi"("section"=w3466, "error in (no error)"=w3468, "key"="Tester Software Ver", "refnum"=w3470) -> ("error out"=w3465:errorcluster, "value"=w3464:string, "refnum out"=w3469:T15)  [unwired: 4 in, 1 out]
            n1545 = call <vilib>:"Close Config Data.vi"("error in (no error)"=w3465, "refnum"=w3469) -> ()  [unwired: 8 in, 2 out]
            n1546 = control-ref of="ATR"() -> (w3512:refnum<vi>)
            n1547 = Concatenate Strings("  Rev-" ("string"), w3471) -> (w3476:string)
            n1548 = property class="Bool (strict)"(reference=w3458) -> ("BoolText.Text"=w3457:string)  [unwired: 1 in, 2 out]
            n1549 = Equal?(x=w3457, y="Report") -> (x = y?=w3452:bool)
            n1550 = case shown="False" w3463 {
              tunnel: w3489 -> [w3538 w3561]
              tunnel: ["N_A" ("read buffer") w3545] -> w3479
              tunnel: [w3542 w3549] -> w3488
              tunnel: w3485 -> [_ w3559]
              tunnel: [w3541 w3552] -> w3484
              tunnel: [w3541 w3550] -> w3482
              tunnel: [w3541 w3548] -> w3481
              tunnel: ["N_A" w3547] -> w3460
              tunnel: w3452 -> [w3537 _]
              frame False {
                w3541 = "N/A" ("read buffer")
                n1551 = case shown="True" w3537 {
                  tunnel: [w3543 w3544] -> w3542
                  tunnel: w3538 -> [w3543 _]
                  frame False {
                  }
                  frame True {
                    n1552 = call "Display Message to User12"() -> ("error out"=w3544:errorcluster)  [unwired: 10 in, 1 out]
                  }
                }
              }
              frame True {
                n1553 = call <vilib>:"Clear Errors.vi"("error in (no error)"=w3561) -> ("error out"=w3563:errorcluster)  [unwired: 5 in, 1 out]
                n1554 = VISA Flush I/O Buffer(VISA resource name=w3559, error in (no error)=w3563) -> (VISA resource name out=w3553:refnum<visa-resource-name>, error out=w3564:errorcluster)  [unwired: 1 in]
                n1555 = call "SerialMarvinMod.vi"("error in (no error)"=w3564, "write buffer"="SN\r\n", "VISA resource name"=w3553) -> ("error out"=w3560:errorcluster, "read buffer"=w3545:string)  [unwired: 7 in]
                n1556 = call <vilib>:"Clear Errors.vi"("error in (no error)"=w3560) -> ("error out"=w3554:errorcluster)  [unwired: 5 in, 1 out]
                n1557 = VISA Flush I/O Buffer(VISA resource name=w3553, error in (no error)=w3554) -> (VISA resource name out=w3555:refnum<visa-resource-name>, error out=w3556:errorcluster)  [unwired: 1 in]
                n1558 = call "SerialMarvinMod.vi"("error in (no error)"=w3556, "write buffer"="VR\r\n", "VISA resource name"=w3555) -> ("error out"=w3558:errorcluster, "read buffer"=w3552:string)  [unwired: 7 in]
                n1559 = call <vilib>:"Clear Errors.vi"("error in (no error)"=w3558) -> ("error out"=w3551:errorcluster)  [unwired: 5 in, 1 out]
                n1560 = property on="UUT" class="DigNum (strict)"(error in=w3551) -> (error out=w3549:errorcluster, "Value"=w3546:u8)  [unwired: 1 in, 1 out]
                n1561 = case shown="63" w3546 {
                  tunnel: ["EBAY 414-8005            " "AHU-L (47) 413-8005-1" "AHU-R (63) 413-8005-2"] -> w3550
                  tunnel: ["414-8005-95" " 413-8005-1-47" " 413-8005-2-63"] -> w3548
                  tunnel: ["414-8005_95_EBAY" " 413-8005_47_AHU" " 413-8005_63_AHU"] -> w3547
                  frame 95, Default {
                    (unwired) "AHU-R (63) 413-8005-2"
                  }
                  frame 47 {
                  }
                  frame 63 {
                  }
                }
              }
            }
            n1562 = call <vilib>:"Check if File or Folder Exists.vi"("error in (no error)"=w3488, "path"=w3503) -> ("error out"=w3501:errorcluster, "file or folder exists?"=w3504:bool, "dup path"=w3502:path)  [unwired: 7 in]
            n1563 = case shown="False" w3504 {
              tunnel: w3501 -> [w3577 w3578]
              tunnel: w3502 -> [w3576 w3579]
              tunnel: [w3575 w3579] -> w3510
              tunnel: [w3574 w3578] -> w3506
              frame False {
                n1564 = Create Folder(path (use dialog)=w3576, error in=w3577) -> (created path=w3575:path, error out=w3574:errorcluster)  [unwired: 1 in, 1 out]
              }
              frame True {
              }
            }
            n1565 = property on="Logger Path" class="Path"(error in=w3506, "Value"=w3510, "StartPath"=w3510) -> (error out=w3507:errorcluster)  [unwired: 1 in, 1 out]
            n1566 = Concatenate Strings("ATR" ("string"), w3460, w3478, w3479, w3478, w3477, ".docx" ("string")) -> (w3451:string)
            n1567 = property on="Logger Path" class="Path"(error in=w3507) -> (error out=w3508:errorcluster, "StartPath"=w3447:path)  [unwired: 1 in, 1 out]
            n1568 = Build Path(base path=w3447, name or relative path=w3451) -> (appended path=w3449:path)
            n1569 = while {
              tunnel: w3451 -> [w3520]
              tunnel: w3447 -> [w3517]
              shift-right: [w3519] -> w3450
              shift-left: w3449 -> [w3518]
              shift-right: [w3515] -> w3445
              shift-left: w3446 -> [w3516]
              tunnel: w3508 -> [w3521]
              tunnel: [w3522] -> w3509
              stop <- w3514 continue-if-true
              n1570 = call <vilib>:"Check if File or Folder Exists.vi"("error in (no error)"=w3521, "path"=w3518) -> ("error out"=w3522:errorcluster, "file or folder exists?"=w3514:bool)  [unwired: 7 in, 1 out]
              n1571 = case shown="True" w3514 {
                tunnel: w3520 -> [_ w3534]
                tunnel: w3516 -> [_ w3526]
                tunnel: [w3524 w3531] -> w3519
                tunnel: w3518 -> [w3524 _]
                tunnel: w3517 -> [_ w3532]
                tunnel: [1 w3525] -> w3515
                frame False {
                }
                frame True {
                  w3527 = ".docx" ("search string")
                  n1572 = Search and Replace String(input string=w3534, search string=w3527) -> (result string=w3533:string)  [unwired: 6 in, 3 out]
                  n1573 = Number To Decimal String(number=w3526) -> (decimal integer string=w3529:string)  [unwired: 1 in]
                  n1574 = call <vilib>:"Space Constant.vi"() -> ("String"=w3528:string)
                  n1575 = Concatenate Strings(w3533, w3528, w3529, w3527) -> (w3530:string)
                  n1576 = Build Path(base path=w3532, name or relative path=w3530) -> (appended path=w3531:path)
                  n1577 = Increment(x=w3526) -> (x+1=w3525:i32)
                }
              }
            }
            n1578 = call "HeaderuRayon.vi"("Tester Software Ver"=w3464, "UUTHeader"=w3462, "UUT"=w3482, "S/N"=w3479, "VR"=w3484, "Oper."=w3483) -> ("HEADER1"=w3511:string)
            n1579 = Open/Create/Replace File(file path (use dialog)=w3450, error in=w3509, operation (0:open)=T20."create") -> (error out=w3494:errorcluster)  [unwired: 3 in, 2 out]
            n1580 = property class="Tbl (strict)"(reference=w3512, error in=w3494) -> (error out=w3486:errorcluster, "Value"=w3513:string[][])  [unwired: 1 out]
            n1581 = call "MarvinReport.vi"("HEADER1"=w3511, "ATR Or"=w3512, "Steps   pfull"=w3513, "Footer UUT"=w3481, "pageNum"=3, "FILE NAME"=w3451, "Report Folder"=w3450, "error in (no error)"=w3486, "REV"=w3476, "Test-Conductor"=w3483) -> ("error out"=w3487:errorcluster)  [unwired: 4 in, 1 out]
            n1582 = Select(t=T12."MainProgram", s=w3452, f=T12."Stop") -> (s? t:f=w3453:T12)
          }
          event "Help Button": Value Change {
            n1583 = event-data() -> ()  [unwired: 1 in, 6 out]
            n1584 = vi-ref "Help.vi"() -> (w3590:refnum<vi>)
            n1585 = invoke class="VI" method="FP.Open"(reference=w3590, error in=w3588, "Activate"=TRUE ("Activate?"), "State"=T18."Standard") -> (error out=w3589:errorcluster)  [unwired: 1 in, 4 out]
            n1586 = call "Help.vi"("error in"=w3589) -> ("error out"=w3581:errorcluster)  [unwired: 7 in]
            n1587 = property on="Help Button" class="Bool (strict)"(error in=w3581, "Value"=FALSE ("Help Button")) -> ()  [unwired: 1 in, 2 out]
          }
          event "Serial Com": Value Change {
            n1588 = event-data() -> ()  [unwired: 1 in, 6 out]
            n1589 = property on="Serial Com" class="Bool"(error in=w3599, "Visible"=FALSE) -> (error out=w3603:errorcluster)  [unwired: 1 in, 1 out]
            n1590 = property on="VISA resource name" class="VISAName"(error in=w3603, "Visible"=TRUE) -> (error out=w3600:errorcluster)  [unwired: 1 in, 1 out]
          }
          event "VISA resource name": Value Change {
            w3606 = T13."Enabled" ("Disabled")
            n1591 = event-data() -> ()  [unwired: 1 in, 6 out]
            n1592 = control-ref of="This VI"() -> (w3620:refnum<vi>)
            n1593 = property on="Pannel User Message" class="Str"(error in=w3609, "Value"="Serial conection in process" ("Pannel User Message")) -> ()  [unwired: 1 in, 2 out]
            n1594 = call "Serial InitMarvin.vi"("error in (no error)"=w3609, "VI reference (current VI)"=w3620, "VISA Refnum in"="VISA resource name") -> ("error out"=w3627:errorcluster, "Boolean"=w3608:bool)  [unwired: 7 in]
            n1595 = property on="Serial" class="Bool (strict)"(error in=w3627, "Value"=w3608) -> (error out=w3624:errorcluster)  [unwired: 1 in, 1 out]
            n1596 = property on="VISA resource name" class="VISAName"(error in=w3624, "Visible"=FALSE) -> (error out=w3623:errorcluster)  [unwired: 1 in, 1 out]
            n1597 = property on="Serial Com" class="Bool"(error in=w3623, "Visible"=TRUE) -> (error out=w3619:errorcluster)  [unwired: 1 in, 1 out]
            n1598 = case shown="True" w3608 {
              tunnel: w3619 -> [w3629 w3645]
              tunnel: [w3629 w3639] -> w3618
              tunnel: "VISA resource name" -> [_ w3641]
              frame False {
              }
              frame True {
                n1599 = call "SerialMarvinMod.vi"("error in (no error)"=w3645, "Clear Log"=FALSE, "write buffer"="SN\r\n", "VISA resource name"=w3641) -> ("error out"=w3640:errorcluster, "read buffer"=→"Curret SN":string)  [unwired: 6 in]
                n1600 = call "SerialMarvinMod.vi"("error in (no error)"=w3640, "Clear Log"=FALSE, "write buffer"="AO[1]\r\n", "VISA resource name"=w3641) -> ("error out"=w3639:errorcluster, "read buffer"=w3632:string)  [unwired: 6 in]
                n1601 = control-ref of="ATR"() -> (w3630:refnum<vi>)
                n1602 = property class="Tbl (strict)"(reference=w3630) -> ("Value"=w3635:string[][])  [unwired: 1 in, 2 out]
                n1603 = Index Array(array=w3635, index (col)=0 ("disabled index (col)")) -> (element=w3637:string[])  [unwired: 1 in]
                n1604 = call "Find_Number_LineMARVIN.vi"("Test Paragraph"="7.5.5.1", "Row Headers[]"=w3637) -> ("Line number"=w3634:i32)  [unwired: 3 in, 3 out]
                n1605 = Replace Array Subset(array=w3635, new element=w3632, index (row)=w3634, index (col)=5 ("disabled index (col)")) -> (w3631:string[][])
                n1606 = property class="Tbl (strict)"(reference=w3630, "Value"=w3631) -> ()  [unwired: 1 in, 2 out]
              }
            }
            n1607 = call <vilib>:"Clear Errors.vi"("error in (no error)"=w3618) -> ("error out"=w3628:errorcluster)  [unwired: 5 in, 1 out]
            n1608 = case shown="True" w3608 {
              tunnel: w3628 -> [w3717 w3721]
              tunnel: [w3717 w3720] -> w3612
              tunnel: "VISA resource name" -> [w3716 w3719]
              tunnel: [w3716 w3718] -> w3613
              frame False {
              }
              frame True {
                n1609 = VISA Flush I/O Buffer(VISA resource name=w3719, error in (no error)=w3721) -> (VISA resource name out=w3718:refnum<visa-resource-name>, error out=w3720:errorcluster)  [unwired: 1 in]
              }
            }
            n1610 = case shown="True" w3608 {
              tunnel: w3612 -> [w3649 w3652]
              tunnel: [w3649 w3651] -> w3611
              tunnel: [FALSE ("Yes") w3650] -> w3610
              frame False {
              }
              frame True {
                n1611 = call "Display Message to User2"("error in (no error)"=w3652) -> ("error out"=w3651:errorcluster, "Yes"=w3650:bool)  [unwired: 9 in]
              }
            }
            n1612 = case shown="True" w3610 {
              tunnel: w3611 -> [w3653 w3655]
              tunnel: [w3653 w3659] -> w3605
              frame False {
              }
              frame True {
                w3656 = T13."Disabled and Grayed Out" ("Disabled")
                n1613 = property on="Serial" class="Bool (strict)"() -> ("Value"=w3657:bool)  [unwired: 2 in, 2 out]
                n1614 = property on="VISA resource name" class="VISAName"() -> ("Value"=w3658:refnum<visa-resource-name>)  [unwired: 2 in, 2 out]
                n1615 = case shown="True" w3657 {
                  selector: w3657 -> [_ w3700]
                  tunnel: w3655 -> [w3661 w3690]
                  tunnel: w3658 -> [_ w3670]
                  tunnel: [w3660 w3669] -> w3659
                  frame False {
                    n1616 = call "Display Message to User3"("error in (no error)"=w3661) -> ("error out"=w3660:errorcluster)  [unwired: 9 in, 1 out]
                  }
                  frame True {
                    w3677 = "Set parameters in process..." ("Strin")
                    n1617 = control-ref of="VISA resource name out"() -> (w3699:refnum<vi>)
                    n1618 = control-ref of="Stop Button"() -> (w3675:refnum<vi>)
                    n1619 = control-ref of="Motor Speed RPM"() -> (w3664:refnum<vi>)
                    n1620 = control-ref of="Pannel User Message"() -> (w3676:refnum<vi>)
                    n1621 = property on="UUT" class="Str"(error in=w3690) -> (error out=w3685:errorcluster, "Value"=w3689:string)  [unwired: 1 in, 1 out]
                    n1622 = Equal?(x=w3689, y="EBAY") -> (x = y?=w3687:bool)
                    n1623 = Byte Array To String(unsigned byte array=u8[] [75, 0, 4, 2, 0, 0, 0, 0] ("appended array")) -> (string=w3698:string)
                    n1624 = Byte Array To String(unsigned byte array=u8[] [75, 0, 4, 2, 0, 0, 0, 0] ("appended array")) -> (string=w3694:string)
                    n1625 = Byte Array To String(unsigned byte array=u8[] [75, 0, 4, 2, 0, 0, 16, 0] ("appended array")) -> (string=w3672:string)
                    n1626 = case shown="False" w3687 {
                      tunnel: [w3705 u16 95 ("Param to Set in")] -> w3686
                      tunnel: w3685 -> [w3702 w3714]
                      tunnel: [w3701 w3714] -> w3684
                      frame False {
                        n1627 = while {
                          tunnel: [w3709] -> w3703
                          tunnel: w3702 -> [w3708]
                          tunnel: [w3707] -> w3701
                          stop <- w3713 stop-if-true
                          n1628 = call "AHU #"("error in (no error)"=w3708) -> ("47"=w3709:bool, "63"=w3712:bool, "OK"=w3710:bool, "error out"=w3707:errorcluster)  [unwired: 15 in]
                          n1629 = Exclusive Or(1:w3712, 2:w3709) -> (0:w3711:bool)
                          n1630 = And(x=w3711, y=w3710) -> (x .and. y?=w3713:bool)
                        }
                        n1631 = Select(t=u16 47 ("Param to Set in"), s=w3703, f=u16 63 ("Param to Set in")) -> (s? t:f=w3705:u16)
                      }
                      frame True {
                      }
                    }
                    n1632 = property class="VISAName"(reference=w3699, error in=w3684) -> (error out=w3696:errorcluster, "Value"=w3674:refnum<visa-resource-name>)  [unwired: 1 out]
                    n1633 = VISA Write(VISA resource name=w3674, write buffer=w3698, error in (no error)=w3696) -> (VISA resource name out=w3692:refnum<visa-resource-name>, error out=w3683:errorcluster)  [unwired: 1 out]
                    n1634 = call "Write panel message (SubVI).vi"(4:"rpm"=w3664, 5:"rpm"=FALSE ("rpm"), "PrintTime"=FALSE, "Stop"=w3675, "error in (no error)"=w3683, "Time to wait"=0.2, "Strin"=w3677, "String in"=w3676) -> ("error out"=w3682:errorcluster)  [unwired: 3 in]
                    n1635 = call "SetParam.vi"("RS"=w3700, "error in (no error)"=w3682, "Param to Set in"=w3686, "Visa"=w3670) -> ("error out"=w3681:errorcluster)  [unwired: 7 in]
                    n1636 = VISA Write(VISA resource name=w3674, write buffer=w3672, error in (no error)=w3681) -> (error out=w3680:errorcluster)  [unwired: 2 out]
                    n1637 = call "Write panel message (SubVI).vi"("rpm"=w3664, "Stop"=w3675, "error in (no error)"=w3680, "Time to wait"=15.0, "Strin"=w3677, "String in"=w3676) -> ("error out"=w3679:errorcluster)  [unwired: 5 in]
                    n1638 = call <vilib>:"Clear Errors.vi"("error in (no error)"=w3679) -> ("error out"=w3693:errorcluster)  [unwired: 5 in, 1 out]
                    n1639 = VISA Write(VISA resource name=w3692, write buffer=w3694, error in (no error)=w3693) -> (error out=w3671:errorcluster)  [unwired: 2 out]
                    n1640 = call "Serial.vi"("error in (no error)"=w3671, "Clear Log"=FALSE, "write buffer"="AO[1]\r\n", "VISA resource name"=w3670) -> ("error out"=w3669:errorcluster, "read buffer"=w3666:string)  [unwired: 5 in, 1 out]
                    n1641 = Equal?(x=w3666, y="") -> ()  [unwired: 1 out]
                  }
                }
                n1642 = property on="Start" class="Bool (strict)"(error in=w3655, "DisabledEnum"=w3656) -> (error out=w3654:errorcluster)  [unwired: 1 in, 1 out]
                n1643 = property on="Report" class="Bool (strict)"(error in=w3654, "DisabledEnum"=w3656) -> ()  [unwired: 1 in, 2 out]
              }
            }
            n1644 = property on="Start" class="Bool (strict)"(error in=w3605, "DisabledEnum"=w3606) -> (error out=w3604:errorcluster)  [unwired: 1 in, 1 out]
            n1645 = property on="Report" class="Bool (strict)"(error in=w3604, "DisabledEnum"=w3606) -> ()  [unwired: 1 in, 2 out]
          }
          event "Refresh Button": Value Change {
            n1646 = event-data() -> ()  [unwired: 1 in, 6 out]
            n1647 = property on="Refresh Button" class="Bool (strict)"("Value"=FALSE ("Refresh Button")) -> ()  [unwired: 2 in, 2 out]
          }
          event Panel Close? {
            w3731 = TRUE ("Stop Button")
            n1648 = event-data() -> ("VIRef"=w3733:refnum<vi>)  [unwired: 1 in, 3 out]
            n1649 = Close Reference(reference=w3733) -> ()  [unwired: 1 in, 1 out]
            n1650 = property on="Stop Button" class="Bool (strict)"(error in=w3732, "Val(Sgnl)"=w3731, "Value"=w3731) -> ()  [unwired: 1 in, 2 out]
            n1651 = event-data("Discard?"=TRUE) -> ()  [unwired: 1 in, 1 out]
            "ClosePanel" <- w3731
          }
          event "Settings": Value Change {
            n1652 = event-data() -> ()  [unwired: 1 in, 6 out]
            n1653 = disable-structure shown="Enabled" {
              disable-tunnel: [w3754 w3757] -> w3742
              disable-tunnel: [w3753 w3757] -> w3741
              frame Disabled {
                n1654 = call "Temperature calibration settings"() -> ("Password"=w3756:dbl, "OK"=w3754:bool)  [unwired: 17 in, 1 out]
                n1655 = Equal?(x=w3756, y=1234.0) -> (x = y?=w3753:bool)
              }
              frame Enabled {
                w3757 = TRUE ("OK")
              }
            }
            n1656 = property on="Serial" class="Bool (strict)"(error in=w3747) -> (error out=w3745:errorcluster, "Value"=w3748:bool)  [unwired: 1 in, 1 out]
            n1657 = Compound Arithmetic op=AND(w3748, w3742, w3741) -> (w3743:bool)
            n1658 = case shown="True" w3743 {
              tunnel: w3745 -> [w3759 w3764]
              tunnel: w3746 -> [_ w3763]
              tunnel: [w3758 w3762] -> w3744
              frame False {
                n1659 = flat-sequence {
                  tunnel: w3759 -> [w3760]
                  tunnel: [w3760] -> w3758
                  frame #0 {
                    n1660 = One Button Dialog(message="Please establish RS connection.") -> ()  [unwired: 1 in, 1 out]
                  }
                }
              }
              frame True {
                n1661 = call "Calibration (SubVI).vi"("error constant"=w3764) -> ("error constant 2"=w3766:errorcluster, "Val"=w3774:dbl[], "K"=w3775:u32[])  [unwired: 8 in]
                n1662 = Concatenate Strings("EP=1\r\nAO" ("string"), "[", "1" ("string"), "]=0", "\r\n" ("write buffer")) -> (w3773:string)
                n1663 = call "SerialMarvinMod.vi"("error in (no error)"=w3766, "Clear Log"=FALSE, "write buffer"=w3773, "VISA resource name"=w3763) -> ("error out"=w3765:errorcluster)  [unwired: 6 in, 1 out]
                n1664 = for {
                  tunnel: w3775 -> [w3825] mode=indexing
                  tunnel: w3763 -> [w3820]
                  tunnel: w3774 -> [w3818] mode=indexing
                  tunnel: [w3809] -> w3808 mode=indexing
                  tunnel: [w3817] -> w3776
                  tunnel: w3765 -> [w3815]
                  tunnel: [w3813] -> w3782
                  n1665 = control-ref of="VISA resource name out"() -> (w3822:refnum<vi>)
                  n1666 = To Unsigned Long Integer(number=w3825) -> (unsigned 32bit integer=w3827:u32)
                  n1667 = Split Number(x=w3827) -> (hi(x)=w3832:u16, lo(x)=w3833:u16)
                  n1668 = Split Number(x=w3833) -> (hi(x)=w3831:u8, lo(x)=w3830:u8)
                  n1669 = Split Number(x=w3832) -> (hi(x)=w3829:u8, lo(x)=w3828:u8)
                  n1670 = property class="VISAName"(reference=w3822, error in=w3815) -> (error out=w3816:errorcluster, "Value"=w3813:refnum<visa-resource-name>)  [unwired: 1 out]
                  n1671 = Build Array(u8 75, u8 0 ("element"), u8 4 ("Length"), u8 2, w3830, w3831, w3828, w3829) -> (w3824:u8[])
                  n1672 = Byte Array To String(unsigned byte array=w3824) -> (string=w3823:string)
                  n1673 = Concatenate Strings("TA" ("string"), "[", "5" ("string"), "]", "\r\n" ("write buffer")) -> (w3837:string)
                  n1674 = VISA Write(VISA resource name=w3813, write buffer=w3823, error in (no error)=w3816) -> (error out=w3819:errorcluster)  [unwired: 2 out]
                  n1675 = call "Wait_Sec.vi"("Delay Time (sec)"=2.0, "error out"=w3819) -> ("error in"=w3811:errorcluster)  [unwired: 2 in]
                  n1676 = call "SerialMarvinMod.vi"("error in (no error)"=w3811, "Clear Log"=FALSE, "write buffer"=w3837, "VISA resource name"=w3820) -> ("error out"=w3817:errorcluster, "read buffer"=w3814:string)  [unwired: 6 in]
                  n1677 = Fract/Exp String To Number(string=w3814) -> (number=w3812:dbl)  [unwired: 3 in, 1 out]
                  n1678 = Subtract(x=w3812, y=w3818) -> (x-y=w3809:dbl)
                }
                n1679 = To Unsigned Long Integer(number=u32 0) -> (unsigned 32bit integer=w3794:u32)
                n1680 = Split Number(x=w3794) -> (hi(x)=w3800:u16, lo(x)=w3801:u16)
                n1681 = Split Number(x=w3801) -> (hi(x)=w3799:u8, lo(x)=w3798:u8)
                n1682 = Split Number(x=w3800) -> (hi(x)=w3797:u8, lo(x)=w3796:u8)
                n1683 = Build Array(u8 75, u8 0 ("element"), u8 4 ("Length"), u8 2, w3798, w3799, w3796, w3797) -> (w3792:u8[])
                n1684 = Byte Array To String(unsigned byte array=w3792) -> (string=w3805:string)
                n1685 = Add Array Elements(numeric array=w3808) -> (sum=w3807:dbl)
                n1686 = Divide(x=w3807, y=4.0) -> (x/y=w3777:dbl)
                n1687 = Number To Fractional String(number=w3777, precision (6)=i16 4) -> (F-format string=w3778:string)  [unwired: 2 in]
                "Cal Value" <- w3778
                n1688 = Concatenate Strings("EP=1\r\nAO" ("string"), "[", "1" ("string"), "]=", w3778, "\r\n" ("write buffer")) -> (w3786:string)
                n1689 = VISA Write(VISA resource name=w3782, write buffer=w3805, error in (no error)=w3776) -> (error out=w3783:errorcluster)  [unwired: 2 out]
                n1690 = call "SerialMarvinMod.vi"("error in (no error)"=w3783, "Clear Log"=FALSE, "write buffer"=w3786, "VISA resource name"=w3763) -> ("error out"=w3781:errorcluster)  [unwired: 6 in, 1 out]
                n1691 = call "SerialMarvinMod.vi"("error in (no error)"=w3781, "write buffer"="AO[1]\r\n", "VISA resource name"=w3763) -> ("error out"=w3762:errorcluster, "read buffer"=w3779:string)  [unwired: 7 in]
                n1692 = Equal?(x=w3778, y=w3779) -> ()  [unwired: 1 out]
              }
            }
          }
        }
        n1693 = Equal?(x="", y=w2831) -> (x = y?=w2833:bool)
        n1694 = Select(t=w2832, s=w2833, f=w2831) -> (s? t:f=w2830:string)
      }
      frame "Initialize" {
        w3848 = T13."Enabled" ("Disabled")
        w3857 = refnum<visa-resource-name> "COM1" ("VISA resource name")
        w3843 = FALSE ("Visible")
        n1695 = disable-structure shown="Disabled" {
          frame Disabled {
            n1696 = local write "UUT"("" ("UUT")) -> ()
          }
          frame Enabled {
          }
        }
        n1697 = property on="Serial Com" class="Bool"(error in=errorcluster {"status"=FALSE, "code"=0, "source"=""} ("error out"), "Visible"=TRUE) -> (error out=w3861:errorcluster)  [unwired: 1 in, 1 out]
        n1698 = property on="VISA resource name" class="VISAName"(error in=w3861, "Visible"=w3843, "Value"=w3857) -> (error out=w3849:errorcluster)  [unwired: 1 in, 1 out]
        n1699 = property on="Stop Burn-in" class="Bool"(error in=w3849, "Visible"=w3843) -> (error out=w3844:errorcluster)  [unwired: 1 in, 1 out]
        n1700 = flat-sequence {
          tunnel: w3844 -> [w3865]
          tunnel: [w3864] -> w3855
          tunnel: [w3867] -> w3854
          tunnel: w3855 -> [w3867]
          tunnel: [w3880] -> w3853
          tunnel: w3854 -> [w3881]
          tunnel: [w3881] -> w3846
          frame #0 {
            n1701 = control-ref of="This VI"() -> (w3866:refnum<vi>)
            n1702 = invoke class="VI" method="Default Vals.Reinit All"(reference=w3866, error in=w3865) -> (error out=w3864:errorcluster)  [unwired: 1 in, 2 out]
          }
          frame #1 {
            w3871 = u32 4294967295  # AccMask
            w3870 = T6 0 items=["使用Flash参数", "使用界面设置参数"] ("InitFlag")
            w3868 = T8 0 items=["normal operation", "Listen-only mode", "test mode"]  # Mode
            w3869 = T7 3 items=["接收所有类型"=1, "只接收标准帧"=2, "只接收扩展帧"=3] ("Fliter")
            w3875 = u8 10 items=["5k bps"=1, "10k bps"=2, "20k bps"=3, "40k bps"=4, "50k bps"=5, "80k bps"=6, "100k bps"=7, "125k bps"=8, "200k bps"=9, "250k bps"=10, "400k bps"=11, "500k bps"=12, "666k bps"=13, "800k bps"=14, "1000k bps"=15, "33.33k bps"=16, "66.66k bps"=17, "83.33k bps"=18]  # kBaudRate
            w3872 = u32 0  # AccCode
            w3873 = T4 4 items=["USB-CAN"=3, "USB-CAN2"=4] ("DevType")
            w3874 = T9 {"DevType"=3, "DevIndex"=0, "CanIndex"=0, "VCI_INIT_CONFIG"={"AccCode"=0, "AccMask"=0, "InitFlag"=1, "Fliter"=7, "Timing0"=0, "Timing1"=0, "Mode"=0}}  # Config
            # "CANalystII"
            n1703 = call "Demo_GetT0T1.vi"("kBaudRate"=w3875) -> ("Timing0"=w3877:u8, "Timing1"=w3878:u8)
            n1704 = Bundle By Name(cluster=w3874, "DevType"=w3873, "CanIndex"="Channel 2", "VCI_INIT_CONFIG.AccCode"=w3872, "VCI_INIT_CONFIG.AccMask"=w3871, "VCI_INIT_CONFIG.InitFlag"=w3870, "VCI_INIT_CONFIG.Fliter"=w3869, "VCI_INIT_CONFIG.Timing0"=w3877, "VCI_INIT_CONFIG.Timing1"=w3878, "VCI_INIT_CONFIG.Mode"=w3868) -> (→"Config_CANAT":T9)
          }
          frame #2 {
            w3882 = u16 284 items=["1M"=20, "500K"=28, "250K"=284, "125K"=796, "100K"=17199, "50K"=18223, "20K"=21295, "10K"=26415, "5K"=32639] ("baud in")
            n1705 = control-ref of="Config_CANAT"() -> (w3880:refnum<vi>)
            n1706 = call "ChangeCANBaud.vi"("baud in"=w3882, "reference"=w3880) -> ()
            n1707 = call "InitCAN_ATII.vi"("Config"=w3880) -> ("Sts"=→"CAN Status":bool)
          }
        }
        n1708 = Wait (ms)(milliseconds to wait=u32 150) -> ()  [unwired: 1 out]
        n1709 = property on="Start" class="Bool (strict)"(error in=w3846, "DisabledEnum"=w3848) -> (error out=w3847:errorcluster)  [unwired: 1 in, 1 out]
        n1710 = property on="Report" class="Bool (strict)"(error in=w3847, "DisabledEnum"=w3848) -> ()  [unwired: 1 in, 2 out]
        "Serial" <- FALSE ("Serial Status")
      }
    }
    "Pannel User Message" <- w2512
  }
